vi "Civ idle2-2.vi"() -> ()   [LabVIEW 2013]
uses:
  <vilib>/Analysis/Matrix/Numeric/Conversions/Matrix To Array - RM.vi
  <vilib>/Analysis/Matrix/NI_Matrix.lvlib
panel:
  out "SP income":dbl
  out "EP income":dbl
  out "Land conversion rate":dbl
  out "BP income":dbl
  in  "Ticks/s":i32
  out "Gold upkeep":dbl
  out "Gold income/s":dbl format="%#_13g"
  out "BP upkeep":dbl
  out "Trading level":i32
  out "Build points":dbl
  out "Gold":dbl format="%#_13g"
  in  "?":T1(tab)
  in  "%Crafters":dbl
  in  "%Engineers":dbl
  in  "%Scientists":dbl
  in  "%Builders":dbl
  in  "%Warriors":dbl
  in  "%Hunters":dbl
  in  "Taxes level 0":bool
  in  "Taxes level 1":bool
  in  "Taxes level 2":bool
  in  "Taxes level 3":bool
  out "Taxation\nlevel":dbl format="%#_13g"
  in  "Taxes level 4":bool
  out "Food consumption\nmultiplier":dbl
  out "Food dissent mod":dbl
  in  "Normal food\nconsumption":bool
  in  "Highest food\nconsumption":bool
  in  "Higher food\nconsumption":bool
  out "Military\nScience level":i32
  out "Governance\nlevel":i32
  in  "Military science":bool
  in  "Governance":bool
  in  "Physics":bool
  in  "Construction":bool
  out "Physics level":i32
  out "Construction\nlevel":i32
  out "Economics\nlevel":i32
  in  "Economics":bool
  in  "Biology":bool
  out "Biology\nlevel":i32
  out "# of level 1 sciences":i32
  out "# of level 2 sciences":i32
  out "# of level 3 sciences":i32
  out "# of level 4 sciences":i32
  out "# of level 5 sciences":i32
  out "# of level 6 sciences":i32
  out "# of level 7 sciences":i32
  out "# of level 8 sciences":i32
  out "# of level 9 sciences":i32
  out "# of level 10 sciences":i32
  out "Production\nlevel":i32
  in  "Production":bool
  out "Spear level":i32
  out "Net level":i32
  in  "Sharpened stick":bool
  in  "Net 1":bool
  in  "Net 2":bool
  in  "Stone\nspear":bool
  in  "Bronze\nSpear":bool
  in  "Iron\nSpear":bool
  out "Bow level":i32
  in  "Bow 1":bool
  in  "Bow 2":bool
  out "Boat level":i32
  in  "Raft":bool
  in  "Trireme":bool
  out "Construction\ntools level":i32
  in  "Stone tools":bool
  in  "Basic\nmetal\ntools":bool
  out "Medicine level":i32
  in  "Medicine 1":bool
  in  "Medicine 2":bool
  in  "Medicine 3":bool
  in  "Advanced\nmetal\ntools":bool
  in  "Longbow":bool
  in  "Farming 1":bool
  out "Farming level":i32
  in  "Farming 2":bool
  out "Writing level":i32
  in  "Writing level 3":bool
  in  "Writing level 2":bool
  in  "Writing level 1":bool
  out "Animal\ndomestication\nlevel":i32
  in  "Livestock":bool
  in  "Selective\nbreeding":bool
  in  "Horses":bool
  out "Sword level":i32
  in  "Steel sword":bool
  in  "Iron sword":bool
  in  "Bronze sword":bool
  out "Tax method\nlevel":i32
  in  "Income tax":bool
  in  "Sales tax":bool
  in  "Tariffs":bool
  out "Siege weapon\nlevel":i32
  out "Chariot level":i32
  in  "Reinforced\nchariot":bool
  in  "Simple\nchariot":bool
  in  "Caravan":bool
  in  "Trebuchet":bool
  in  "Catapult":bool
  in  "Ballista":bool
  in  "Cannon":bool
  in  "Howitzer":bool
  in  "Rocket artillery":bool
  in  "Democracy":bool
  in  "Theocracy":bool
  in  "Warrior\nSociety":bool
  in  "Democracy 2":bool
  in  "Theocracy 2":bool
  in  "Warrior\nSociety 2":bool
  in  "Kingdom":bool
  in  "Republic":bool
  in  "Confederacy":bool
  in  "Senate":bool
  in  "Caste system":bool
  in  "Feudalism":bool
  out "Brick house level":i32
  out "Road level":i32
  out "Hut level":i32
  in  "Hut level 0":bool
  in  "Hut level 1":bool
  in  "Hut level 2":bool
  in  "Hut level 3":bool
  out "Road invested points":dbl
  out "Hut invested points":dbl
  in  "Road level 0":bool
  in  "Road level 3":bool
  in  "Road level 2":bool
  in  "Road level 1":bool
  out "Aqueduct level":i32
  out "Circus\ninvested points":dbl
  out "Circus/arena level":i32
  out "Aqueduct\ninvested points":dbl
  out "Harbor\ninvested points":dbl
  out "Harbor level":i32
  out "School invested points":dbl
  in  "School\nlevel 1":bool
  in  "School\nlevel 2":bool
  in  "School\nlevel 3":bool
  in  "School\nlevel 0":bool
  out "School level":i32
  in  "Wall level 1":bool
  in  "Wall level 2":bool
  in  "Wall level 3":bool
  in  "Wall level 0":bool
  out "Barracks level":i32
  out "Walls level":i32
  out "Wall invested points":dbl
  out "Barracks\ninvested points":dbl
  in  "Barracks\nlevel 3":bool
  in  "Barracks\nlevel 1":bool
  in  "Barracks\nlevel 0":bool
  in  "Barracks\nlevel 2":bool
  out "University level":i32
  in  "University\nlevel 0":bool
  in  "University\nlevel 3":bool
  in  "University\nlevel 2":bool
  in  "University\nlevel 1":bool
  out "University\ninvested points":dbl
  out "Mansion level":i32
  out "Temple level":i32
  out "Mansion\ninvested points":dbl
  out "Temple\ninvested points":dbl
  in  "Make Tier 2\nproducts":bool
  out "Tier 2\nproducts\nupkeep":dbl format="%#_13g"
  out "Tier 3\nproducts\nupkeep":dbl format="%#_13g"
  out "Tier 4\nproducts\nupkeep":dbl format="%#_13g"
  out "Tier 1\nproducts":dbl format="%#_13g"
  out "Tier 2\nproducts":dbl format="%#_13g"
  out "Tier 3\nproducts":dbl format="%#_13g"
  out "Tier 4\nproducts":dbl format="%#_13g"
  out "Tier 1\nproducts\nupkeep":dbl format="%#_13g"
  in  "Make Tier3\nproducts":bool
  in  "Make Tier 4\nproducts":bool
  out "hunting b":dbl
  out "hunting a":dbl
  out "warrior a":dbl
  out "warrior b":dbl
  out "warrior c":dbl
  out "1-Dissent/100":dbl format="%#_13g"
  out "Dissent multiplier":dbl
  out "Land conv mult":dbl
  out "Warrior b Gov mult":dbl
  out "Gov Economy\nbuildings mod":dbl
  out "-dissent per\nmilitary building":dbl
  out "Temp land change/s":dbl
  out "Year":i32
  out "Day":i32
  out "Military Modifier":dbl format="%#_13g"
  out "Taxation\nModifier":dbl format="%#_13g"
  out "Non-land production multiplier":dbl
  out "Hut non-land prod mod":dbl
  out "Hut upkeep":dbl
  out "Hut dissent mod":dbl
  out "Dissent addition modifiers":dbl
  out "Road land prod mod":dbl
  out "Road upkeep":dbl
  out "Road expansion bonus":dbl
  out "Trading level no mod":i32
  out "Taxes dissent mod":dbl
  out "Barracks military bonus":dbl
  out "Barracks upkeep":dbl
  out "Wall upkeep":dbl
  out "Wall dissent mod":dbl
  out "Construction multiplier":dbl
  out "Wall warrior % equivalent":dbl
  out "Gov building\nupkeep mod":dbl
  out "School dissent mod":dbl
  out "School upkeep":dbl
  out "School engineer equivalent":dbl
  out "School SP/EP multiplier":dbl
  out "Medicine dissent mod":i32
  out "Gov populist\nbuildings mod":dbl
  out "Gov elitist\nbuildings mod":dbl
  out "University SP multiplier":dbl
  out "University dissent mod":dbl
  out "University upkeep":dbl
  out "University scientist equivalent":dbl
  out "food income":dbl
  out "Aqueduct dissent mod":dbl
  out "Aqueduct upkeep":dbl
  out "Mansion dissent mod":dbl
  out "Mansion upkeep":dbl
  out "Harbor dissent mod":dbl
  out "Harbor upkeep":dbl
  out "Circus dissent mod":dbl
  out "Circus upkeep":dbl
  out "Temple dissent mod":dbl
  out "Temple upkeep":dbl
  out "Harbor military mod":dbl
  out "SP/EP multiplier":dbl
  out "Government":string
  out "Dissent":dbl
  out "SP":dbl
  out "EP":dbl
  in  "Percentage or absolute":bool
  out "Engineers":i32
  out "Crafters":i32
  out "Scientists":i32
  in  "#Merchants":dbl
  in  "Assign Merchant":bool
  in  "#Engineers":dbl
  in  "Assign Engineer":bool
  in  "#Scientists":dbl
  in  "Assign Scientist":bool
  out "Warriors":i32
  in  "Assign Builder":bool
  in  "#Builders":dbl
  out "Builders":i32
  in  "Assign Warrior":bool
  in  "#Warriors":dbl
  out "Unassigned workers":i32
  in  "Assign Hunters":bool
  in  "#Hunters":dbl
  in  "# people":i32
  in  "Increase\nPopulation":bool
  out "Conquered\nland":dbl
  out "Max hunters":i32
  out "Hunters":i32
  out "Food/s":dbl
  out "Permanent\nland":dbl
  out "People":i64
  in  "Stop Loop":bool
  out "Food":dbl
  # "Produces food, but your permanent land cannot support too many hunters"
  # "Conquers land, starting at 1km^2 per warrior, but has diminishing returns"
  # "Produces 1 BP/s, needed for buildings\nand for building upkeep"
  # "Produces 0.1 SP/s, used for abstract research which unlock upgrades and provide bonuses"
  # "Produces 0.1 EP/s, used for designing useful tools and upgrades"
  # "Produces Products, used mostly for late game upgrades.  Production scales with permanent land"
  # "Medium income from population, 8% dissent modifier"
  # "High income from population, 15% dissent modifier"
  # "Highest  income from population, 25% dissent modifier"
  # "No income from population, no dissent modifier"
  # "Low income from population, 3% dissent modifier"
  # "2 food/s/person,\n-10% dissent"
  # "1 food/s/person, no dissent mod"
  # "1.5 food/s/person,\n-5% dissent"
  # "Requires Governance 2"
  # "Each level costs 1000 *10^current level SP"
  # "Reduces diminishing returns \nfrom military size, unlocks \nnew weapons/tactics"
  # "Slightly decreases dissent,\nunlocks new governments"
  # "Increases EP and SP generation, \nunlocks various upgrades"
  # "Decreases building upkeep costs,\nunlocks buildings"
  # "Increase gold generation,\nunlocks gold and taxation"
  # "Increase food production,\nunlocks farming and medicine"
  # "Increases production by 20%\nper tier per level"
  # "Costs 2,000EP\nHunters and warriors are more effective"
  # "Costs 10,000EP\nRequires military 1,\nHunters and warriors are more effective"
  # "Costs 50,000EP\nRequires military 2,\nWarriors are more effective"
  # "Costs 2,000,000EP\nRequires military 4,\nWarriors are more effective"
  # "Costs 10,000EP\nHunters can produce more food"
  # "Costs 100,000EP\nHunters can produce more food"
  # "Costs 100,000EP\nRequires military 3,\nWarriors are much more effective, hunters can produce more food"
  # "Costs 300,000EP\nRequires military 3, physics 3\nWarriors and Hunters are more effective"
  # "Costs 30M EP\nRequires military 5, physics 4\nWarriors are more effective"
  # "Costs 300,000EP\nRequires physics 3,\nImproves trade and hunting"
  # "Costs 3,000,000EP\nRequires physics 4, military 3\nImproves trade and warriors"
  # "Costs 30,000EP\nRequires physics 2, construction 2\nBuilders produce 0.5 more BP/s"
  # "Costs 500,000EP\nRequires physics 3,\nconstruction 3,Builders produce 0.5 more BP/s"
  # "Costs 200M EP\nRequires physics 5,\nconstruction 5,Builders produce 1 more BP/s"
  # "Costs 30,000EP\nRequires biology 2,\nreduces dissent by another 1% (2% total)"
  # "Costs 3M EP\nRequires biology 4,\nreduces dissent by another 2% (4% total)"
  # "Costs 3,000EP\nRequires biology 1,\nreduces dissent by 1%"
  # "Costs 10M EP\nRequires Biology 3\nRenames hunters to farmers, massive improvements to food production, increases food from tribute"
  # "Costs 100M EP\nRequires Biology 4\nLarge improvements to food production, increases food from tribute"
  # "Costs 10k EP\nImproves EP and SP production by 10%"
  # "Costs 1M EP\nImproves EP and SP production by 10%"
  # "Costs 100M EP\nImproves EP and SP production by 10%"
  # "Costs 30M EP\nRequires Biology 3\nImproves warrior effectiveness,  builder BP/s by 0.5"
  # "Costs 30k EP\nRequires Biology 1\nImproves hunter food production"
  # "Costs 1M EP\nRequires Biology 2\nImproves warrior effectiveness,  builder BP/s by 0.5"
  # "Costs 1M EP\nRequires Military 3\nImproves warrior effectiveness"
  # "Costs 30M EP\nRequires Military 4\nImproves warrior effectiveness"
  # "Costs 1B EP\nRequires Military 6\nImproves warrior effectiveness"
  # "Costs 1M EP\nRequires Economics 3\nImproves taxation effectiveness by 50%"
  # "Costs 30M EP\nRequires Economics 4\nImproves taxation effectiveness by 50%"
  # "Costs 1B EP\nRequires Economics 6\nImproves taxation effectiveness by 50%"
  # "Costs 500k EP\nRequires Military 3, Physics 3, Improves warrior effectiveness"
  # "Costs 5M EP\nRequires Military 3, Physics 4, Improves warrior effectiveness"
  # "Costs 10M EP\nRequires Economics 4, Physics 4, Increases trade level"
  # "Costs 5M EP\nRequires Military 3, Physics 4, Improves\nwarrior effectiveness"
  # "Costs 30M EP\nRequires Military 3, Physics 5, Improves\nwarrior effectiveness"
  # "Costs 300M EP\nRequires Military 4, Physics 6, Improves\nwarrior effectiveness"
  # "Costs 3B EP\nRequires Military 6, Physics 7, Improves\nwarrior effectiveness"
  # "Costs 30B EP\nRequires Military 7, Physics 8, Improves\nwarrior effectiveness"
  # "Costs 300B EP\nRequires Military 8, Physics 9, Improves\nwarrior effectiveness"
  # "Costs 1000SP\nRequires Governance 1"
  # "Costs 25000SP\nRequires Governance 2"
  # "Costs 5M SP\nRequires Governance 4"
  # "Reduces dissent by 2,4,6%\nImproves non-land production by 10,20,30%\nRequires Construction 1"
  # "Upkeep:        0                          0.01BP                0.03BP              0.15BP"
  # "Cost:             0                          10k   BP              30k BP            150k BP"
  # "Increases trade level by 1,2,3\nImproves land production\n by 10,20,30%\nImproves land conversion\nrate by 20,50,100%\nRequires Construction 1"
  # "Upkeep:        0                          0.02BP                0.06BP              0.2BP"
  # "Cost:             0                          50k BP              150k BP             500k BP"
  # "Increases military effectiveness (b) by 10,20,30%\nRequires Construction 2, Military 2"
  # "Upkeep:        0                          0.001GP             0.003GP             0.01GP"
  # "Cost:             0                          100k BP             300k BP              1M BP"
  # "Adds to the base strength of your military, giving the equivalent of 2,4,6% of your population as warriors\nReduces dissent by 2,4,6%\nRequires Construction 3, Military 2"
  # "Upkeep:        0                          0.002GP            0.006GP            0.02GP"
  # "Cost:             0                          1M BP              3M BP               10M BP"
  # "Provides a 5,10,15% bonus to SP/EP production, reduces dissent by 1,2,3%, adds 1,2,3% of population to base  engineer\nRequires Construction 2, Governance 2"
  # "Upkeep:        0                          0.001GP             0.003GP           0.01GP"
  # "Cost:              0                          200k BP             600k BP            2M BP"
  # "Provides a 5,10,15% bonus to SP/EP production, reduces dissent by 1,2,3%, adds 1,2,3% of population to base  engineer\nRequires Construction 2, Governance 2"
  # "Upkeep:        0                          0.005GP             0.015GP          0.05GP"
  # "Cost:              0                          600k BP             2M BP             5M BP"
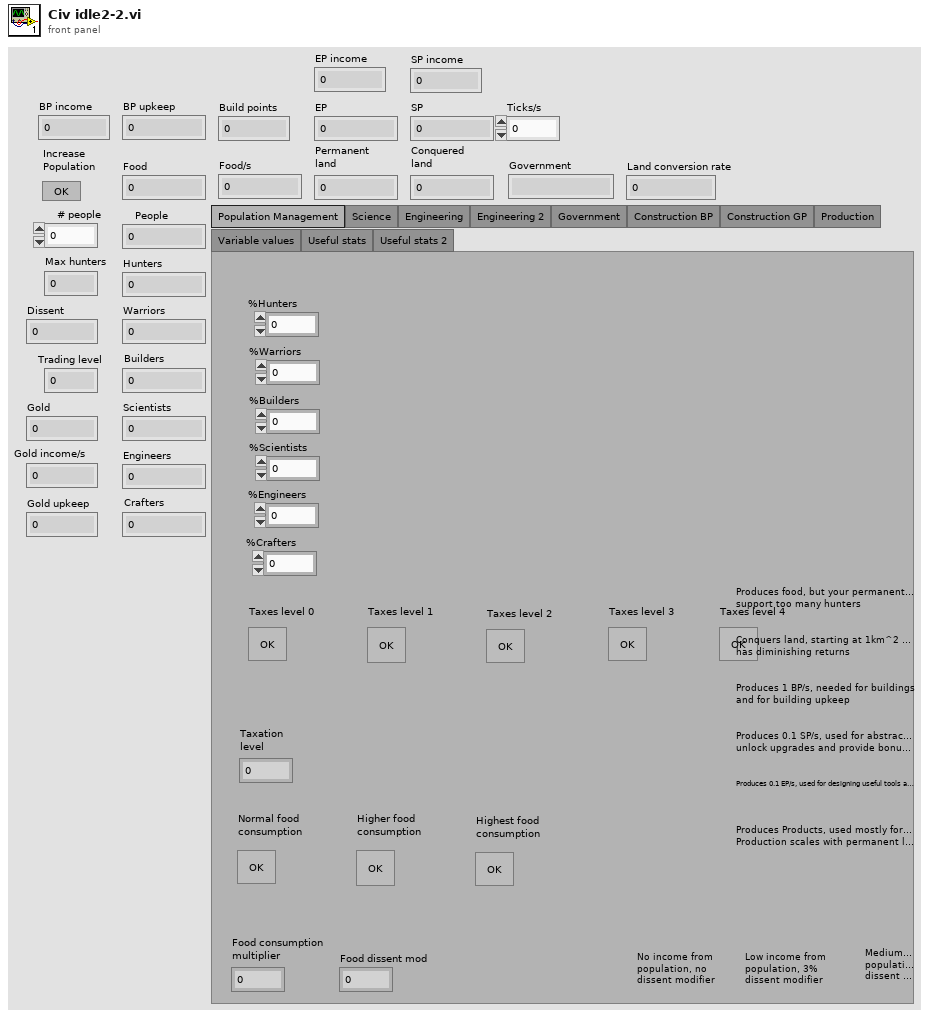
[diagram p1: front panel]
types:
  T1 = enum32{"Population Management", "Science", "Engineering", "Engineering 2", "Government", "Construction BP", "Construction GP", "Production", "Variable values", "Useful stats", "Useful stats 2"}
  T2 = typedef "NI_Matrix.lvlib/RealMatrix.ctl" = dbl[][]
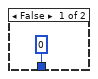
[diagram p2: hidden frame]
diagram:
  n1 = while {
    i -> [w1520]
    stop <- "Stop Loop" stop-if-true
    w168 = 10000000 ("y")
    w179 = 10000000 ("y")
    w200 = 10000000 ("y")
    w237 = 10000000 ("y")
    w226 = 5000000 ("y")
    w217 = 500000 ("y")
    w270 = 10000000 ("y")
    w281 = 5000000 ("y")
    w290 = 500000 ("y")
    w306 = 1000000000 ("y")
    w317 = 30000000 ("y")
    w326 = 1000000 ("y")
    w384 = 1000000000 ("y")
    w373 = 30000000 ("y")
    w364 = 1000000 ("y")
    w393 = 30000000 ("y")
    w404 = 1000000 ("y")
    w413 = 30000 ("y")
    w444 = 100000000 ("y")
    w433 = 1000000 ("y")
    w424 = 10000 ("y")
    w473 = 1 ("y")
    w465 = 2 ("y")
    w464 = 1.5 ("y")
    w508 = 0 ("y")
    w509 = 3 ("y")
    w528 = 2 ("y")
    w529 = 1 ("y")
    w568 = 30000000 ("y")
    w584 = 500000 ("y")
    w602 = 3000000 ("y")
    w613 = 30000 ("y")
    w628 = 3000 ("y")
    w685 = 0 ("y")
    w684 = 3 ("y")
    w665 = 2 ("y")
    w664 = 1 ("y")
    w711 = "Senate" ("y")
    w735 = "Caste system" ("y")
    w748 = "Feudalism" ("y")
    w786 = "Kingdom" ("y")
    w762 = "Republic" ("y")
    w749 = "Confederacy" ("y")
    w801 = 3 ("y")
    w818 = 500000 ("y")
    w829 = 30000 ("y")
    w877 = 0 ("y")
    w878 = 3 ("y")
    w897 = 2 ("y")
    w898 = 1 ("y")
    w941 = 0 ("y")
    w942 = 3 ("y")
    w961 = 2 ("y")
    w962 = 1 ("y")
    w1004 = 0 ("y")
    w1005 = 3 ("y")
    w1020 = 2 ("y")
    w1021 = 1 ("y")
    w1126 = 3 ("y")
    w1137 = 2 ("y")
    w1175 = 0 ("y")
    w1174 = 3 ("y")
    w1155 = 2 ("y")
    w1154 = 1 ("y")
    w1195 = 0 ("y")
    w1196 = 1 ("y")
    w1208 = 100000000 ("y")
    w1235 = 10000000 ("y")
    w1258 = 3000000 ("y")
    w1269 = 300000 ("y")
    w1301 = 300000 ("y")
    w1327 = 100000 ("y")
    w1330 = 2000000 ("y")
    w1329 = 50000 ("y")
    w1393 = "Warrior Society 2" ("y")
    w1417 = "Theocracy 2" ("y")
    w1430 = "Democracy 2" ("y")
    w1437 = "Warrior Society" ("y")
    w1450 = "Theocracy" ("y")
    w1466 = "Democracy" ("y")
    w1490 = 2000 ("y")
    # "Constructions initial build"
    # "SCIENCES"
    # "GOVERNMENTS"
    # "ENGINEERING"
    n2 = local read "Food consumption\nmultiplier"() -> (w474:dbl)
    n3 = local read "Barracks\ninvested points"() -> (w1036:dbl)
    n4 = local read "Wall invested points"() -> (w921:dbl)
    n5 = local read "Food consumption\nmultiplier"() -> (w466:dbl)
    n6 = local read "Governance\nlevel"() -> (w471:i32)
    n7 = local read "Military\nScience level"() -> (w863:i32)
    n8 = local read "Governance\nlevel"() -> (w479:i32)
    n9 = local read "Construction\nlevel"() -> (w1186:i32)
    n10 = local read "Construction\nlevel"() -> (w889:i32)
    n11 = local read "Construction\nlevel"() -> (w1163:i32)
    n12 = local read "Military\nScience level"() -> (w850:i32)
    n13 = local read "Construction\nlevel"() -> (w866:i32)
    n14 = local read "Build points"() -> (w917:dbl)
    n15 = local read "Barracks level"() -> (w1181:i32)
    n16 = local read "Build points"() -> (w1040:dbl)
    n17 = local read "Military\nScience level"() -> (w844:i32)
    n18 = local read "Walls level"() -> (w871:i32)
    n19 = local read "Build points"() -> (w1180:dbl)
    n20 = local read "Build points"() -> (w872:dbl)
    n21 = local read "Walls level"() -> (w894:i32)
    n22 = local read "Barracks level"() -> (w1158:i32)
    n23 = Subtract(x=3000000 ("y"), y=w921) -> (x-y=w914:dbl)
    n24 = Subtract(x=300000 ("y"), y=w1036) -> (x-y=w1043:dbl)
    n25 = Greater Or Equal?(x=w479, y=2) -> (x >= y?=w481:bool)
    n26 = And(x="Normal food\nconsumption", y=w481) -> (x .and. y?=w477:bool)
    n27 = Greater Or Equal?(x=w471, y=2) -> (x >= y?=w483:bool)
    n28 = And(x="Highest food\nconsumption", y=w483) -> (x .and. y?=w469:bool)
    n29 = local read "Food consumption\nmultiplier"() -> (w455:dbl)
    n30 = local read "Ticks/s"() -> (w792:i32)
    n31 = Not Equal?(x=w474, y=w473) -> (x != y?=w476:bool)
    n32 = And(x=w476, y=w477) -> (x .and. y?=w475:bool)
    n33 = Max & Min(x=w914, y=0.0) -> (max(x,y)=w919:dbl)  [unwired: 1 out]
    n34 = Greater Or Equal?(x=w863, y=2) -> (x >= y?=w861:bool)
    n35 = Not Equal?(x=w466, y=w465) -> (x != y?=w468:bool)
    n36 = And(x=w468, y=w469) -> (x .and. y?=w467:bool)
    n37 = Max & Min(x=w1043, y=0.0) -> (max(x,y)=w1038:dbl)  [unwired: 1 out]
    n38 = Greater Or Equal?(x=w917, y=w919) -> (x >= y?=w918:bool)
    n39 = local read "Military\nScience level"() -> (w857:i32)
    n40 = Greater Or Equal?(x=w1040, y=w1038) -> (x >= y?=w1039:bool)
    n41 = for {
      N: 1 -> [_]
      tunnel: [w2227] -> w1144 mode=indexing
      n42 = local read "Production\nlevel"() -> (w2223:i32)
      n43 = local read "Permanent\nland"() -> (w2224:dbl)
      n44 = local read "Construction multiplier"() -> (w2253:dbl)
      n45 = local read "University scientist equivalent"() -> (w2240:dbl)
      n46 = local read "Taxation\nlevel"() -> (w2290:dbl)
      n47 = local read "1-Dissent/100"() -> (w2222:dbl)
      n48 = local read "Conquered\nland"() -> (w2305:dbl)
      n49 = local read "Non-land production multiplier"() -> (w2198:dbl)
      n50 = local read "Tier 2\nproducts"() -> (w2213:dbl)
      n51 = local read "Government"() -> (w2308:string)
      n52 = local read "University SP multiplier"() -> (w2237:dbl)
      n53 = local read "Economics\nlevel"() -> (w2291:i32)
      n54 = local read "SP/EP multiplier"() -> (w2246:dbl)
      n55 = local read "People"() -> (w2227:i64)
      n56 = local read "Conquered\nland"() -> (w2294:dbl)
      n57 = local read "Crafters"() -> (w2228:i32)
      n58 = local read "Economics\nlevel"() -> (w2296:i32)
      n59 = local read "Trading level"() -> (w2295:i32)
      n60 = local read "Non-land production multiplier"() -> (w2279:dbl)
      n61 = local read "School engineer equivalent"() -> (w2249:dbl)
      n62 = local read "Taxation\nModifier"() -> (w2288:dbl)
      n63 = local read "Tax method\nlevel"() -> (w2231:i32)
      n64 = local read "1-Dissent/100"() -> (w2281:dbl)
      n65 = local read "Physics level"() -> (w2282:i32)
      n66 = local read "Tier 2\nproducts\nupkeep"() -> (w2204:dbl)
      n67 = Power Of X(1:w2227, 2:-0.5 ("y")) -> (0:w2225:dbl)
      n68 = Power Of X(1:1.2 ("x"), 2:w2223) -> (0:w2212:dbl)
      n69 = case shown="\"Tribe\", Default" w2308 {
        tunnel: w2227 -> [w2356 w2368 w2377 w2393 w2398 w2417 w2427 w2449 w2463 w2485 w2498 w2516 w2536 _ _ _ _ _ _ _ _ _ _ _ _ _ _ _]
        tunnel: w2224 -> [_ w2370 w2378 _ _ _ _ w2454 w2462 _ w2503 _ w2533 _ _ _ _ _ _ _ _ _ _ _ _ _ _ _]
        tunnel: [w2359 w2366 w2376 w2389 w2401 w2410 w2429 w2446 w2461 w2481 w2491 w2509 w2525 _ _ _ _ _ _ _ _ _ _ _ _ _ _ _] -> w2306
        tunnel: w2305 -> [_ _ _ _ _ w2421 w2428 w2453 _ _ w2502 w2519 _ _ _ _ _ _ _ _ _ _ _ _ _ _ _ _]
        tunnel: [1 0.85 0.7 1 1 2 3 1.5 ("y") 1.0 ("y") 2.0 ("y") 3.0 ("y") 6.0 ("y") 0.7 ("y") _ _ _ _ _ _ _ _ _ _ _ _ _ _ _] -> w2304
        tunnel: [1.0 2.0 4.0 1.0 1.0 0.2 0.05 1.5 ("y") 3.0 ("y") 1.0 ("y") 0.1 ("y") 0.025 ("y") 8.0 ("y") _ _ _ _ _ _ _ _ _ _ _ _ _ _ _] -> w2303
        tunnel: [1 1 1 0.5 0.333 1 1 1.0 ("y") 0.5 ("y") 0.5 ("y") 1.0 ("y") 1.0 ("y") 1.0 ("y") _ _ _ _ _ _ _ _ _ _ _ _ _ _ _] -> w2261
        tunnel: [1.0 ("y") 1.5 ("y") 2.0 ("y") 0.5 ("y") 0.33 ("y") 0.5 ("y") 0.5 ("y") 1.25 ("y") 2.0 ("y") 1.0 ("y") 0.5 ("y") 0.5 ("y") 2.5 ("y") _ _ _ _ _ _ _ _ _ _ _ _ _ _ _] -> w2252
        tunnel: [1.0 ("y") 0.75 ("y") 0.5 ("y") 1.5 ("y") 2.0 ("y") 1.5 ("y") 1.5 ("y") 1.25 ("y") 0.5 ("y") 1.0 ("y") 1.5 ("y") 2.0 ("y") 0.5 ("y") _ _ _ _ _ _ _ _ _ _ _ _ _ _ _] -> w2245
        tunnel: [0.0 ("y") _ _ 0.5 ("y") 0.5 ("y") 1.0 ("y") 1.0 ("y") 1.0 ("y") _ 0.5 ("y") 1.0 ("y") 0.0 ("y") 0.0 ("y") _ _ _ _ _ _ _ _ _ _ _ _ _ _ _] -> w2244
        tunnel: [1.0 ("y") _ _ _ _ _ _ 1.25 ("y") 1.5 ("y") 0.7 ("y") 0.5 ("y") 0.5 ("y") 1.0 ("y") _ _ _ _ _ _ _ _ _ _ _ _ _ _ _] -> w2243
        frame "Tribe", Default {
          n70 = Divide(x=w2356, y=i64 2) -> (x/y=w2354:dbl)
          n71 = Subtract(x=w2354, y=i64 50) -> (x-y=w2359:dbl)
        }
        frame "Democracy" {
          n72 = Square Root(x=w2370) -> (sqrt(x)=w2369:dbl)
          n73 = Divide(x=w2368, y=w2369) -> (x/y=w2367:dbl)
          n74 = Square Root(x=w2367) -> (sqrt(x)=w2372:dbl)
          n75 = Multiply(x=2, y=w2372) -> (x*y=w2366:dbl)
        }
        frame "Democracy 2" {
          n76 = Square Root(x=w2378) -> (sqrt(x)=w2382:dbl)
          n77 = Divide(x=w2377, y=w2382) -> (x/y=w2381:dbl)
          n78 = Square Root(x=w2381) -> (sqrt(x)=w2376:dbl)
        }
        frame "Theocracy" {
          n79 = Y-th Root of X(1:w2393, 2:i64 3 ("y")) -> (0:w2390:dbl)
          n80 = Add(x=w2390, y=15.0) -> (x+y=w2389:dbl)
        }
        frame "Theocracy 2" {
          n81 = Y-th Root of X(1:w2398, 2:3.5 ("y")) -> (0:w2404:dbl)
          n82 = Add(x=w2404, y=15.0) -> (x+y=w2401:dbl)
        }
        frame "Warrior Society" {
          n83 = Square Root(x=w2417) -> (sqrt(x)=w2414:dbl)
          n84 = Y-th Root of X(1:w2421, 2:3.0 ("y")) -> (0:w2420:dbl)
          n85 = Multiply(x=0.5, y=w2414) -> (x*y=w2413:dbl)
          n86 = Add(x=w2413, y=10.0) -> (x+y=w2412:dbl)
          n87 = Multiply(x=w2420, y=2.0) -> (x*y=w2411:dbl)
          n88 = Subtract(x=w2412, y=w2411) -> (x-y=w2410:dbl)
        }
        frame "Warrior Society 2" {
          n89 = Square Root(x=w2427) -> (sqrt(x)=w2437:dbl)
          n90 = Y-th Root of X(1:w2428, 2:2.5 ("y")) -> (0:w2433:dbl)
          n91 = Multiply(x=0.4, y=w2437) -> (x*y=w2438:dbl)
          n92 = Add(x=w2438, y=10.0) -> (x+y=w2439:dbl)
          n93 = Multiply(x=w2433, y=1.0) -> (x*y=w2440:dbl)
          n94 = Subtract(x=w2439, y=w2440) -> (x-y=w2429:dbl)
        }
        frame "Senate" {
          n95 = Multiply(x=w2454, y=w2453) -> (x*y=w2452:dbl)
          n96 = Power Of X(1:w2452, 2:0.3 ("y")) -> (0:w2450:dbl)
          n97 = Divide(x=w2449, y=w2450) -> (x/y=w2448:dbl)
          n98 = Y-th Root of X(1:w2448, 2:2.0 ("y")) -> (0:w2444:dbl)
          n99 = Multiply(x=1.5, y=w2444) -> (x*y=w2446:dbl)
        }
        frame "Republic" {
          n100 = Power Of X(1:w2462, 2:0.6 ("y")) -> (0:w2468:dbl)
          n101 = Divide(x=w2463, y=w2468) -> (x/y=w2467:dbl)
          n102 = Y-th Root of X(1:w2467, 2:2.0 ("y")) -> (0:w2464:dbl)
          n103 = Multiply(x=1.5, y=w2464) -> (x*y=w2461:dbl)
        }
        frame "Kingdom" {
          n104 = Power Of X(1:w2485, 2:0.2564 ("y")) -> (0:w2482:dbl)
          n105 = Add(x=w2482, y=5.0) -> (x+y=w2481:dbl)
        }
        frame "Feudalism" {
          n106 = Multiply(x=w2503, y=w2502) -> (x*y=w2501:dbl)
          n107 = Y-th Root of X(1:w2498, 2:3.0 ("y")) -> (0:w2497:dbl)
          n108 = Y-th Root of X(1:w2501, 2:7.0 ("y")) -> (0:w2492:dbl)
          n109 = Divide(x=w2497, y=2.0) -> (x/y=w2495:dbl)
          n110 = Add(x=w2495, y=5.0) -> (x+y=w2493:dbl)
          n111 = Subtract(x=w2493, y=w2492) -> (x-y=w2491:dbl)
        }
        frame "Caste system" {
          n112 = Y-th Root of X(1:w2516, 2:3.5 ("y")) -> (0:w2515:dbl)
          n113 = Y-th Root of X(1:w2519, 2:4.5 ("y")) -> (0:w2510:dbl)
          n114 = Multiply(x=w2515, y=0.7) -> (x*y=w2513:dbl)
          n115 = Add(x=w2513, y=10.0) -> (x+y=w2511:dbl)
          n116 = Subtract(x=w2511, y=w2510) -> (x-y=w2509:dbl)
        }
        frame "Confederacy" {
          n117 = Power Of X(1:w2536, 2:0.9 ("y")) -> (0:w2534:dbl)
          n118 = Square Root(x=w2533) -> (sqrt(x)=w2537:dbl)
          n119 = Divide(x=w2534, y=w2537) -> (x/y=w2526:dbl)
          n120 = Power Of X(1:w2526, 2:0.55 ("y")) -> (0:w2525:dbl)
        }
        frame "Imperialism" {
        }
        frame "Empire" {
        }
        frame "Free market capitalism" {
        }
        frame "Corporatism" {
        }
        frame "Fascism" {
        }
        frame "Communist dictatorship" {
        }
        frame "Socialism" {
        }
        frame "Advanced democracy?" {
        }
        frame "Advanced imperialism?" {
        }
        frame "Meritocracy" {
        }
        frame "Genetically optimized workforce" {
        }
        frame "Future democracy?" {
        }
        frame "Hivemind" {
        }
        frame "AI overlord" {
        }
        frame "Robots do all work" {
        }
      }
      n121 = local read "Build points"() -> (w2255:dbl)
      n122 = local read "Build points"() -> (w2262:dbl)
      n123 = Compound Arithmetic op=MULTIPLY(w2228, w2198, w2225, w2224, w2212, w2222, 0.001 ("x")) -> (w2220:dbl)
      n124 = local read "Builders"() -> (w2264:i32)
      n125 = local read "Tier 3\nproducts"() -> (w2210:dbl)
      n126 = local read "Tier 1\nproducts"() -> (w2219:dbl)
      n127 = local read "Tier 1\nproducts\nupkeep"() -> (w2216:dbl)
      n128 = Add(x=w2220, y=w2219) -> (x+y=w2217:dbl)
      n129 = local read "Dissent"() -> (w2300:dbl)
      n130 = local read "Tier 3\nproducts\nupkeep"() -> (w2202:dbl)
      n131 = local read "Tier 4\nproducts\nupkeep"() -> (w2201:dbl)
      n132 = Power Of X(1:2 ("x"), 2:w2231) -> (0:w2229:dbl)
      n133 = Compound Arithmetic op=MULTIPLY(w2296, w2295, w2294, 0.001 ("value")) -> (w2260:dbl)
      n134 = local write "Gov populist\nbuildings mod"(w2252) -> ()
      n135 = local write "-dissent per\nmilitary building"(w2244) -> ()
      n136 = Compound Arithmetic op=MULTIPLY(w2227, w2291, w2290, w2288, 0.0005 ("value"), w2229) -> (w2259:dbl)
      n137 = local write "Gov elitist\nbuildings mod"(w2245) -> ()
      n138 = local read "Gold"() -> (w2292:dbl)
      n139 = Power Of X(1:1.1 ("x"), 2:w2282) -> (0:w2266:dbl)
      n140 = Subtract(x=w2217, y=w2216) -> (x-y=w2197:dbl)
      n141 = Divide(x=w2255, y=10.0) -> (x/y=w2254:dbl)
      n142 = Compound Arithmetic op=ADD(w2292, w2260, w2259) -> (w2283:dbl)
      n143 = Divide(x=w2300, y=100.0) -> (x/y=w2302:dbl)
      n144 = Compound Arithmetic op=MULTIPLY(w2266, w2281, 0.1, w2279, w2246) -> (w2267:dbl)
      n145 = Divide(x=w2267, y=w2266) -> (x/y=w2265:dbl)
      n146 = Compound Arithmetic op=MULTIPLY(w2265, 10.0 ("value"), w2264, w2253, w2246) -> (w2251:dbl)
      n147 = Add(x=w2251, y=w2262) -> (x+y=w2263:dbl)
      n148 = Less?(x=w2283, y=-50.0) -> (x < y?=w2286:bool)
      n149 = local read "Tier 4\nproducts"() -> (w2207:dbl)
      n150 = Greater?(x=w2197, y=0.0) -> (0:w2195:bool)
      n151 = Subtract(x=1.0, y=w2302) -> (x-y=w2298:dbl)
      n152 = Add(x=w2260, y=w2259) -> (x+y=w2258:dbl)
      n153 = local read "Dissent addition modifiers"() -> (w2275:dbl)
      n154 = local read "Engineers"() -> (w2248:i32)
      n155 = And(x="Make Tier 2\nproducts", y=w2195) -> (x .and. y?=w2193:bool)
      n156 = local write "Build points"(w2263) -> ()
      n157 = local write "Gold income/s"(w2258) -> ()
      n158 = case shown="True" w2286 {
        tunnel: w2283 -> [_ w2344]
        tunnel: w2227 -> [_ w2348]
        tunnel: [0 w2345] -> w2272
        frame False {
        }
        frame True {
          n159 = Negate(x=w2344) -> (-x=w2343:dbl)
          n160 = Divide(x=w2343, y=w2348) -> (x/y=w2347:dbl)
          n161 = Max & Min(x=w2347, y=20.0) -> (min(x,y)=w2345:dbl)  [unwired: 1 out]
        }
      }
      n162 = local read "Scientists"() -> (w2241:i32)
      n163 = local write "Gold"(w2283) -> ()
      n164 = Less?(x=w2254, y=-50.0) -> (x < y?=w2274:bool)
      n165 = local write "1-Dissent/100"(w2298) -> ()
      n166 = local read "Dissent multiplier"() -> (w2307:dbl)
      n167 = local write "Warrior b Gov mult"(w2304) -> ()
      n168 = Multiply(x=w2306, y=w2307) -> (x*y=w2277:dbl)
      n169 = case shown="True" w2193 {
        tunnel: w2197 -> [w2328 w2334]
        tunnel: w2212 -> [_ w2331]
        tunnel: [w2328 w2330] -> w2218
        tunnel: [0.0 w2329] -> w2214
        frame False {
        }
        frame True {
          n170 = Divide(x=100.0 ("y"), y=w2331) -> (x/y=w2333:dbl)
          n171 = Quotient & Remainder(x=w2334, y=w2333) -> (x-y*floor(x/y)=w2330:dbl, floor(x/y)=w2329:dbl)
        }
      }
      n172 = Add(x=w2214, y=w2213) -> (x+y=w2205:dbl)
      n173 = Subtract(x=w2205, y=w2204) -> (x-y=w2191:dbl)
      n174 = Greater?(x=w2191, y=0.0) -> (0:w2190:bool)
      n175 = And(x="Make Tier3\nproducts", y=w2190) -> (x .and. y?=w2188:bool)
      n176 = case shown="True" w2188 {
        tunnel: w2191 -> [w2320 w2326]
        tunnel: w2212 -> [_ w2323]
        tunnel: [w2320 w2322] -> w2211
        tunnel: [0.0 w2321] -> w2209
        frame False {
        }
        frame True {
          n177 = Divide(x=100.0 ("y"), y=w2323) -> (x/y=w2325:dbl)
          n178 = Quotient & Remainder(x=w2326, y=w2325) -> (x-y*floor(x/y)=w2322:dbl, floor(x/y)=w2321:dbl)
        }
      }
      n179 = local write "Tier 2\nproducts"(w2211) -> ()
      n180 = Add(x=w2209, y=w2210) -> (x+y=w2203:dbl)
      n181 = Subtract(x=w2203, y=w2202) -> (x-y=w2183:dbl)
      n182 = Greater?(x=w2183, y=0.0) -> (0:w2187:bool)
      n183 = And(x="Make Tier 4\nproducts", y=w2187) -> (x .and. y?=w2184:bool)
      n184 = case shown="True" w2184 {
        tunnel: w2183 -> [w2312 w2318]
        tunnel: w2212 -> [_ w2316]
        tunnel: [w2312 w2315] -> w2208
        tunnel: [0.0 w2314] -> w2200
        frame False {
        }
        frame True {
          n185 = Divide(x=100.0 ("y"), y=w2316) -> (x/y=w2313:dbl)
          n186 = Quotient & Remainder(x=w2318, y=w2313) -> (x-y*floor(x/y)=w2315:dbl, floor(x/y)=w2314:dbl)
        }
      }
      n187 = local write "Land conv mult"(w2303) -> ()
      n188 = Multiply(x=w2227, y=w2240) -> (x*y=w2239:dbl)
      n189 = case shown="True" w2274 {
        tunnel: w2227 -> [_ w2341]
        tunnel: [0 w2338] -> w2268
        tunnel: w2254 -> [_ w2336]
        frame False {
        }
        frame True {
          n190 = Negate(x=w2336) -> (-x=w2337:dbl)
          n191 = Divide(x=w2337, y=w2341) -> (x/y=w2340:dbl)
          n192 = Max & Min(x=w2340, y=20.0) -> (min(x,y)=w2338:dbl)  [unwired: 1 out]
        }
      }
      n193 = Add(x=w2272, y=w2268) -> (x+y=w2271:dbl)
      n194 = Add(x=w2277, y=w2275) -> (x+y=w2276:dbl)
      n195 = local read "EP"() -> (w2310:dbl)
      n196 = Multiply(x=w2249, y=w2227) -> (x*y=w2250:dbl)
      n197 = Subtract(x=w2200, y=w2201) -> (x-y=w2199:dbl)
      n198 = Add(x=w2199, y=w2207) -> (x+y=w2206:dbl)
      n199 = local read "SP"() -> (w2242:dbl)
      n200 = local write "Gov Economy\nbuildings mod"(w2243) -> ()
      n201 = Add(x=w2248, y=w2250) -> (x+y=w2247:dbl)
      n202 = Multiply(x=w2267, y=w2247) -> (x*y=w2236:dbl)
      n203 = local write "Gov building\nupkeep mod"(w2261) -> ()
      n204 = Max & Min(x=0.0, y=w2276) -> (max(x,y)=w2284:dbl)  [unwired: 1 out]
      n205 = Add(x=w2239, y=w2241) -> (x+y=w2238:dbl)
      n206 = Compound Arithmetic op=MULTIPLY(w2267, w2237, w2238) -> (w2235:dbl)
      n207 = Max & Min(x=w2271, y=20.0) -> (min(x,y)=w2269:dbl)  [unwired: 1 out]
      n208 = Add(x=w2269, y=w2284) -> (x+y=w2234:dbl)
      n209 = Add(x=w2310, y=w2236) -> (x+y=w2309:dbl)
      n210 = Add(x=w2242, y=w2235) -> (x+y=w2278:dbl)
      n211 = local write "Tier 3\nproducts"(w2208) -> ()
      n212 = Max & Min(x=90.0, y=w2234) -> (min(x,y)=w2232:dbl)  [unwired: 1 out]
      n213 = local write "Tier 4\nproducts"(w2206) -> ()
      n214 = local write "Tier 1\nproducts"(w2218) -> ()
      n215 = local write "BP income"(w2251) -> ()
      n216 = local write "EP"(w2309) -> ()
      n217 = local write "SP"(w2278) -> ()
      n218 = local write "SP income"(w2235) -> ()
      n219 = local write "EP income"(w2236) -> ()
      n220 = local write "Dissent"(w2232) -> ()
    }
    n221 = Greater Or Equal?(x=w1186, y=2) -> (x >= y?=w1177:bool)
    n222 = Greater Or Equal?(x=w866, y=3) -> (x >= y?=w875:bool)
    n223 = Greater Or Equal?(x=w1180, y=0) -> (x >= y?=w1178:bool)
    n224 = Greater Or Equal?(x=w872, y=0) -> (x >= y?=w874:bool)
    n225 = case shown="True" w475 {
      tunnel: w473 -> [_ w1665]
      frame False {
      }
      frame True {
        n226 = local write "Food consumption\nmultiplier"(w1665) -> ()
        n227 = local write "Food dissent mod"(0.0 ("Taxes dissent add mod")) -> ()
      }
    }
    n228 = Greater Or Equal?(x=w889, y=3) -> (x >= y?=w895:bool)
    n229 = Greater Or Equal?(x=w850, y=2) -> (x >= y?=w849:bool)
    n230 = Greater Or Equal?(x=w1163, y=2) -> (x >= y?=w1157:bool)
    n231 = case shown="True" w467 {
      tunnel: w465 -> [_ w1667]
      frame False {
      }
      frame True {
        n232 = local write "Food consumption\nmultiplier"(w1667) -> ()
        n233 = local write "Food dissent mod"(-10.0 ("Taxes dissent add mod")) -> ()
      }
    }
    n234 = Not Equal?(x=w1181, y=w1175) -> (x != y?=w1183:bool)
    n235 = Not Equal?(x=w871, y=w877) -> (x != y?=w869:bool)
    n236 = Greater Or Equal?(x=w844, y=2) -> (x >= y?=w843:bool)
    n237 = Not Equal?(x=w894, y=w897) -> (x != y?=w892:bool)
    n238 = Not Equal?(x=w1158, y=w1155) -> (x != y?=w1160:bool)
    n239 = local read "Road land prod mod"() -> (w1121:dbl)
    n240 = Max & Min(x=w792, y=0.1) -> (max(x,y)=w791:dbl)  [unwired: 1 out]
    n241 = local read "People"() -> (w456:i64)
    n242 = local read "hunting b"() -> (w1543:dbl)
    n243 = local read "hunting b"() -> (w1542:dbl)
    n244 = Compound Arithmetic op=AND(w1177, w1178, w861) -> (w1176:bool)
    n245 = And(x="Barracks\nlevel 0", y=w1176) -> (x .and. y?=w1184:bool)
    n246 = And(x=w1183, y=w1184) -> (x .and. y?=w1182:bool)
    n247 = case shown="True" w1182 {
      tunnel: w1175 -> [_ w1958]
      frame False {
      }
      frame True {
        n248 = local write "Barracks level"(w1958) -> ()
        n249 = local write "Barracks military bonus"(1.0 ("Hut dissent add mod")) -> ()
        n250 = local write "Barracks upkeep"(0.0 ("Hut non-land prod mod")) -> ()
      }
    }
    n251 = Compound Arithmetic op=AND(w875, w874, w849) -> (w876:bool)
    n252 = And(x="Wall level 0", y=w876) -> (x .and. y?=w868:bool)
    n253 = And(x=w869, y=w868) -> (x .and. y?=w870:bool)
    n254 = case shown="True" w870 {
      tunnel: w877 -> [_ w1816]
      frame False {
      }
      frame True {
        n255 = local write "Wall warrior % equivalent"(0.0 ("Hut dissent add mod")) -> ()
        n256 = local write "Walls level"(w1816) -> ()
        n257 = local write "Wall dissent mod"(0.0 ("Hut non-land prod mod")) -> ()
        n258 = local write "Wall upkeep"(0.0 ("Hut non-land prod mod")) -> ()
      }
    }
    n259 = Compound Arithmetic op=AND(w895, w918, w843) -> (w896:bool)
    n260 = And(x="Wall level 2", y=w896) -> (x .and. y?=w891:bool)
    n261 = And(x=w892, y=w891) -> (x .and. y?=w893:bool)
    n262 = case shown="True" w893 {
      tunnel: w897 -> [_ w1834]
      tunnel: w919 -> [_ w1830]
      tunnel: w921 -> [_ w1829]
      frame False {
      }
      frame True {
        n263 = local read "Build points"() -> (w1833:dbl)
        n264 = Add(x=w1830, y=w1829) -> (x+y=w1831:dbl)
        n265 = local write "Wall warrior % equivalent"(4.0 ("Hut dissent add mod")) -> ()
        n266 = local write "Walls level"(w1834) -> ()
        n267 = local write "Wall dissent mod"(-4.0 ("Hut non-land prod mod")) -> ()
        n268 = local write "Wall invested points"(w1831) -> ()
        n269 = local write "Wall upkeep"(0.006 ("Hut non-land prod mod")) -> ()
        n270 = Subtract(x=w1833, y=w1830) -> (x-y=w1832:dbl)
        n271 = local write "Build points"(w1832) -> ()
      }
    }
    n272 = local read "1-Dissent/100"() -> (w1385:dbl)
    n273 = Reciprocal(x=w791) -> (1/x=w788:dbl)
    n274 = case shown="False" "Percentage or absolute" {
      frame False {
        n275 = Add(x="%Hunters", y="%Warriors") -> (x+y=w2547:dbl)
        n276 = Add(x="%Builders", y="%Scientists") -> (x+y=w2548:dbl)
        n277 = Add(x="%Engineers", y="%Crafters") -> (x+y=w2545:dbl)
        n278 = Add(x=w2547, y=w2548) -> (x+y=w2546:dbl)
        n279 = Add(x=w2546, y=w2545) -> (x+y=w2550:dbl)
        n280 = Less Or Equal?(x=w2550, y=100.0) -> (x <= y?=w2551:bool)
        n281 = case shown="True" w2551 {
          tunnel: "%Hunters" -> [_ w2573]
          tunnel: "%Warriors" -> [_ w2572]
          tunnel: "%Builders" -> [_ w2571]
          tunnel: "%Scientists" -> [_ w2570]
          tunnel: "%Engineers" -> [_ w2569]
          tunnel: "%Crafters" -> [_ w2568]
          frame False {
          }
          frame True {
            n282 = local read "People"() -> (w2555:i64)
            n283 = Divide(x=w2555, y=100.0) -> (x/y=w2566:dbl)
            n284 = Multiply(x=w2571, y=w2566) -> (x*y=w2559:dbl)
            n285 = Multiply(x=w2573, y=w2566) -> (x*y=w2553:dbl)
            n286 = Multiply(x=w2572, y=w2566) -> (x*y=w2560:dbl)
            n287 = Multiply(x=w2566, y=w2570) -> (x*y=w2563:dbl)
            n288 = Multiply(x=w2566, y=w2569) -> (x*y=w2562:dbl)
            n289 = Multiply(x=w2566, y=w2568) -> (x*y=w2561:dbl)
            n290 = local write "Scientists"(w2563) -> ()
            n291 = local write "Warriors"(w2560) -> ()
            n292 = local write "Builders"(w2559) -> ()
            n293 = local write "Engineers"(w2562) -> ()
            n294 = local write "Crafters"(w2561) -> ()
            n295 = Add(x=w2553, y=w2560) -> (x+y=w2565:dbl)
            n296 = Add(x=w2563, y=w2562) -> (x+y=w2564:dbl)
            n297 = Add(x=w2565, y=w2559) -> (x+y=w2558:dbl)
            n298 = Add(x=w2564, y=w2561) -> (x+y=w2557:dbl)
            n299 = Add(x=w2558, y=w2557) -> (x+y=w2556:dbl)
            n300 = Subtract(x=w2555, y=w2556) -> (x-y=w2554:dbl)
            n301 = Add(x=w2553, y=w2554) -> (x+y=w2552:dbl)
            n302 = local write "Hunters"(w2552) -> ()
          }
        }
      }
      frame True {
        n303 = local read "Unassigned workers"() -> (w2637:i32)
        n304 = local read "Unassigned workers"() -> (w2646:i32)
        n305 = local read "Unassigned workers"() -> (w2611:i32)
        n306 = local read "Unassigned workers"() -> (w2601:i32)
        n307 = local read "Unassigned workers"() -> (w2630:i32)
        n308 = local read "Unassigned workers"() -> (w2591:i32)
        n309 = local read "Hunters"() -> (w2614:i32)
        n310 = local read "Scientists"() -> (w2602:i32)
        n311 = local read "Engineers"() -> (w2592:i32)
        n312 = local read "Warriors"() -> (w2616:i32)
        n313 = local read "Builders"() -> (w2615:i32)
        n314 = local read "Crafters"() -> (w2582:i32)
        n315 = Greater Or Equal?(x="#Hunters", y=0.0) -> (x >= y?=w2643:bool)
        n316 = Greater Or Equal?(x="#Scientists", y=0.0) -> (x >= y?=w2608:bool)
        n317 = Greater Or Equal?(x="#Warriors", y=0.0) -> (x >= y?=w2634:bool)
        n318 = Greater Or Equal?(x="#Engineers", y=0.0) -> (x >= y?=w2598:bool)
        n319 = Greater Or Equal?(x="#Builders", y=0.0) -> (x >= y?=w2627:bool)
        n320 = Greater Or Equal?(x="#Merchants", y=0.0) -> (x >= y?=w2588:bool)
        n321 = Add(x=w2646, y=w2614) -> (x+y=w2645:i32)
        n322 = Add(x=w2611, y=w2602) -> (x+y=w2610:i32)
        n323 = Add(x=w2637, y=w2616) -> (x+y=w2636:i32)
        n324 = Add(x=w2601, y=w2592) -> (x+y=w2600:i32)
        n325 = Add(x=w2630, y=w2615) -> (x+y=w2629:i32)
        n326 = Add(x=w2591, y=w2582) -> (x+y=w2590:i32)
        n327 = Greater Or Equal?(x=w2645, y="#Hunters") -> (x >= y?=w2642:bool)
        n328 = Greater Or Equal?(x=w2610, y="#Scientists") -> (x >= y?=w2607:bool)
        n329 = Greater Or Equal?(x=w2636, y="#Warriors") -> (x >= y?=w2633:bool)
        n330 = Greater Or Equal?(x=w2600, y="#Engineers") -> (x >= y?=w2597:bool)
        n331 = Greater Or Equal?(x=w2629, y="#Builders") -> (x >= y?=w2626:bool)
        n332 = Greater Or Equal?(x=w2590, y="#Merchants") -> (x >= y?=w2587:bool)
        n333 = And(x=w2642, y=w2643) -> (x .and. y?=w2641:bool)
        n334 = And(x=w2607, y=w2608) -> (x .and. y?=w2606:bool)
        n335 = And(x=w2633, y=w2634) -> (x .and. y?=w2632:bool)
        n336 = And(x=w2597, y=w2598) -> (x .and. y?=w2596:bool)
        n337 = And(x=w2626, y=w2627) -> (x .and. y?=w2625:bool)
        n338 = And(x=w2587, y=w2588) -> (x .and. y?=w2586:bool)
        n339 = And(x=w2641, y="Assign Hunters") -> (x .and. y?=w2639:bool)
        n340 = And(x=w2606, y="Assign Scientist") -> (x .and. y?=w2604:bool)
        n341 = And(x=w2632, y="Assign Warrior") -> (x .and. y?=w2631:bool)
        n342 = And(x=w2596, y="Assign Engineer") -> (x .and. y?=w2594:bool)
        n343 = And(x=w2625, y="Assign Builder") -> (x .and. y?=w2624:bool)
        n344 = And(x=w2586, y="Assign Merchant") -> (x .and. y?=w2584:bool)
        n345 = case shown="True" w2639 {
          tunnel: "#Hunters" -> [_ w2658]
          tunnel: [w2657 w2658] -> w2622
          tunnel: w2614 -> [w2657 _]
          frame False {
          }
          frame True {
            n346 = local write "Hunters"(w2658) -> ()
          }
        }
        n347 = case shown="True" w2604 {
          tunnel: "#Scientists" -> [_ w2652]
          tunnel: [w2651 w2652] -> w2579
          tunnel: w2602 -> [w2651 _]
          frame False {
          }
          frame True {
            n348 = local write "Scientists"(w2652) -> ()
          }
        }
        n349 = case shown="True" w2631 {
          tunnel: "#Warriors" -> [_ w2656]
          tunnel: [w2655 w2656] -> w2617
          tunnel: w2616 -> [w2655 _]
          frame False {
          }
          frame True {
            n350 = local write "Warriors"(w2656) -> ()
          }
        }
        n351 = case shown="True" w2594 {
          tunnel: "#Engineers" -> [_ w2650]
          tunnel: [w2649 w2650] -> w2578
          tunnel: w2592 -> [w2649 _]
          frame False {
          }
          frame True {
            n352 = local write "Engineers"(w2650) -> ()
          }
        }
        n353 = case shown="True" w2624 {
          tunnel: "#Builders" -> [_ w2654]
          tunnel: [w2653 w2654] -> w2580
          tunnel: w2615 -> [w2653 _]
          frame False {
          }
          frame True {
            n354 = local write "Builders"(w2654) -> ()
          }
        }
        n355 = case shown="True" w2584 {
          tunnel: "#Merchants" -> [_ w2648]
          tunnel: [w2647 w2648] -> w2577
          tunnel: w2582 -> [w2647 _]
          frame False {
          }
          frame True {
            n356 = local write "Crafters"(w2648) -> ()
          }
        }
        n357 = local read "People"() -> (w2619:i64)
        n358 = Add(x=w2578, y=w2577) -> (x+y=w2576:dbl)
        n359 = Add(x=w2580, y=w2579) -> (x+y=w2575:dbl)
        n360 = Add(x=w2622, y=w2617) -> (x+y=w2621:dbl)
        n361 = Add(x=w2575, y=w2576) -> (x+y=w2574:dbl)
        n362 = Add(x=w2621, y=w2574) -> (x+y=w2620:dbl)
        n363 = Subtract(x=w2619, y=w2620) -> (x-y=w2618:dbl)
        n364 = local write "Unassigned workers"(w2618) -> ()
      }
    }
    n365 = local read "Military\nScience level"() -> (w846:i32)
    n366 = local read "Permanent\nland"() -> (w1250:dbl)
    n367 = local read "Biology\nlevel"() -> (w1220:i32)
    n368 = local read "Food"() -> (w1541:dbl)
    n369 = Multiply(x=w456, y=w455) -> (x*y=w453:dbl)
    n370 = local read "Hunters"() -> (w1386:i32)
    n371 = Greater Or Equal?(x=w857, y=2) -> (x >= y?=w855:bool)
    n372 = Compound Arithmetic op=AND(w1157, w1039, w855) -> (w1156:bool)
    n373 = And(x="Barracks\nlevel 2", y=w1156) -> (x .and. y?=w1161:bool)
    n374 = And(x=w1160, y=w1161) -> (x .and. y?=w1159:bool)
    n375 = case shown="True" w1159 {
      tunnel: w1155 -> [_ w1974]
      tunnel: w1038 -> [_ w1970]
      tunnel: w1036 -> [_ w1969]
      frame False {
      }
      frame True {
        n376 = local read "Build points"() -> (w1973:dbl)
        n377 = Add(x=w1970, y=w1969) -> (x+y=w1971:dbl)
        n378 = local write "Barracks level"(w1974) -> ()
        n379 = local write "Barracks military bonus"(1.2 ("Hut dissent add mod")) -> ()
        n380 = local write "Barracks\ninvested points"(w1971) -> ()
        n381 = local write "Barracks upkeep"(0.003 ("Hut non-land prod mod")) -> ()
        n382 = Subtract(x=w1973, y=w1970) -> (x-y=w1972:dbl)
        n383 = local write "Build points"(w1972) -> ()
      }
    }
    n384 = Multiply(x=w788, y=1000.0) -> (x*y=w790:dbl)
    n385 = local read "hunting a"() -> (w1540:dbl)
    n386 = local read "Military\nScience level"() -> (w859:i32)
    n387 = local read "Barracks\ninvested points"() -> (w1037:dbl)
    n388 = local read "Wall invested points"() -> (w920:dbl)
    n389 = Wait (ms)(milliseconds to wait=w790) -> ()  [unwired: 1 out]
    n390 = Greater Or Equal?(x=w846, y=2) -> (x >= y?=w847:bool)
    n391 = Compound Arithmetic op=MULTIPLY(w1386, w1121, w1385) -> (w1384:dbl)
    n392 = Power Of X(1:1.05 ("x"), 2:w1220) -> (0:w451:dbl)
    n393 = local read "1-Dissent/100"() -> (w1391:dbl)
    n394 = local read "Barracks\ninvested points"() -> (w1029:dbl)
    n395 = local read "Wall invested points"() -> (w928:dbl)
    n396 = local read "hunting a"() -> (w1392:dbl)
    n397 = Multiply(x=w1250, y=w1543) -> (x*y=w1562:dbl)
    n398 = local read "Governance\nlevel"() -> (w458:i32)
    n399 = local read "Construction\nlevel"() -> (w906:i32)
    n400 = Multiply(x=w1540, y=w1384) -> (x*y=w1553:dbl)
    n401 = local read "Food consumption\nmultiplier"() -> (w463:dbl)
    n402 = Multiply(x=w1562, y=5) -> (x*y=w1560:dbl)
    n403 = local read "Build points"() -> (w1046:dbl)
    n404 = local read "Build points"() -> (w911:dbl)
    n405 = local read "Construction\nlevel"() -> (w1146:i32)
    n406 = Multiply(x=w1553, y=0.1 ("x")) -> (x*y=w1565:dbl)
    n407 = Subtract(x=100000 ("y"), y=w1037) -> (x-y=w1049:dbl)
    n408 = Subtract(x=1000000 ("y"), y=w920) -> (x-y=w908:dbl)
    n409 = local read "Wall warrior % equivalent"() -> (w804:dbl)
    n410 = Multiply(x=w1392, y=w1391) -> (x*y=w1390:dbl)
    n411 = Quotient & Remainder(x=w1560, y=w1390) -> (floor(x/y)=→"Max hunters":dbl)  [unwired: 1 out]
    n412 = local read "Construction\nlevel"() -> (w886:i32)
    n413 = local read "Construction\nlevel"() -> (w1166:i32)
    n414 = local read "Build points"() -> (w922:dbl)
    n415 = local read "Barracks level"() -> (w1151:i32)
    n416 = Divide(x=w1565, y=w1250) -> (x/y=w1564:dbl)
    n417 = local read "Walls level"() -> (w881:i32)
    n418 = local read "Barracks level"() -> (w1171:i32)
    n419 = local read "Build points"() -> (w1035:dbl)
    n420 = local read "Walls level"() -> (w901:i32)
    n421 = Greater Or Equal?(x=w859, y=2) -> (x >= y?=w858:bool)
    n422 = Greater Or Equal?(x=w1146, y=2) -> (x >= y?=w1152:bool)
    n423 = Subtract(x=10000000 ("y"), y=w928) -> (x-y=w925:dbl)
    n424 = Max & Min(x=w1049, y=0.0) -> (max(x,y)=w1044:dbl)  [unwired: 1 out]
    n425 = Max & Min(x=w908, y=0.0) -> (max(x,y)=w913:dbl)  [unwired: 1 out]
    n426 = Multiply(x=100, y="# people") -> (x*y=w1525:i32)
    n427 = Subtract(x=1000000 ("y"), y=w1029) -> (x-y=w1032:dbl)
    n428 = Subtract(x=w1542, y=w1564) -> (x-y=w1563:dbl)
    n429 = local read "Conquered\nland"() -> (w1249:dbl)
    n430 = Greater Or Equal?(x=w1046, y=w1044) -> (x >= y?=w1045:bool)
    n431 = Greater Or Equal?(x=w911, y=w913) -> (x >= y?=w912:bool)
    n432 = Multiply(x=w1553, y=w1563) -> (x*y=w1552:dbl)
    n433 = local read "Farming level"() -> (w1218:i32)
    n434 = local read "Trading level"() -> (w1119:i32)
    n435 = local read "Road land prod mod"() -> (w1120:dbl)
    n436 = Max & Min(x=w925, y=0.0) -> (max(x,y)=w927:dbl)  [unwired: 1 out]
    n437 = Greater Or Equal?(x=w458, y=2) -> (x >= y?=w482:bool)
    n438 = And(x="Higher food\nconsumption", y=w482) -> (x .and. y?=w460:bool)
    n439 = Max & Min(x=w1032, y=0.0) -> (max(x,y)=w1030:dbl)  [unwired: 1 out]
    n440 = Greater Or Equal?(x=w922, y=w927) -> (x >= y?=w926:bool)
    n441 = Greater Or Equal?(x=w886, y=3) -> (x >= y?=w880:bool)
    n442 = Greater Or Equal?(x=w1035, y=w1030) -> (x >= y?=w1031:bool)
    n443 = Greater Or Equal?(x=w906, y=3) -> (x >= y?=w900:bool)
    n444 = Compound Arithmetic op=AND(w1152, w1045, w858) -> (w1153:bool)
    n445 = And(x="Barracks\nlevel 1", y=w1153) -> (x .and. y?=w1148:bool)
    n446 = Compound Arithmetic op=AND(w900, w912, w847) -> (w899:bool)
    n447 = And(x="Wall level 1", y=w899) -> (x .and. y?=w904:bool)
    n448 = Greater Or Equal?(x=w1166, y=2) -> (x >= y?=w1172:bool)
    n449 = Not Equal?(x=w463, y=w464) -> (x != y?=w461:bool)
    n450 = And(x=w461, y=w460) -> (x .and. y?=w462:bool)
    n451 = Not Equal?(x=w881, y=w878) -> (x != y?=w883:bool)
    n452 = Not Equal?(x=w1151, y=w1154) -> (x != y?=w1149:bool)
    n453 = And(x=w1149, y=w1148) -> (x .and. y?=w1150:bool)
    n454 = Not Equal?(x=w901, y=w898) -> (x != y?=w903:bool)
    n455 = And(x=w903, y=w904) -> (x .and. y?=w902:bool)
    n456 = Not Equal?(x=w1171, y=w1174) -> (x != y?=w1169:bool)
    n457 = case shown="True" w462 {
      tunnel: w464 -> [_ w1669]
      frame False {
      }
      frame True {
        n458 = local write "Food consumption\nmultiplier"(w1669) -> ()
        n459 = local write "Food dissent mod"(-5.0 ("Taxes dissent add mod")) -> ()
      }
    }
    n460 = local read "1-Dissent/100"() -> (w1388:dbl)
    n461 = local read "Military\nScience level"() -> (w842:i32)
    n462 = Multiply(x=w1119, y=0.5) -> (x*y=w1118:dbl)
    n463 = Increment(x=w1218) -> (x+1=w1216:i32)
    n464 = local read "Military\nScience level"() -> (w853:i32)
    n465 = case shown="True" w1150 {
      tunnel: w1154 -> [_ w1982]
      tunnel: w1037 -> [_ w1979]
      tunnel: w1044 -> [_ w1977]
      frame False {
      }
      frame True {
        n466 = local read "Build points"() -> (w1981:dbl)
        n467 = Add(x=w1977, y=w1979) -> (x+y=w1978:dbl)
        n468 = local write "Barracks level"(w1982) -> ()
        n469 = local write "Barracks military bonus"(1.1 ("Hut dissent add mod")) -> ()
        n470 = local write "Barracks\ninvested points"(w1978) -> ()
        n471 = local write "Barracks upkeep"(0.001 ("Hut non-land prod mod")) -> ()
        n472 = Subtract(x=w1981, y=w1977) -> (x-y=w1980:dbl)
        n473 = local write "Build points"(w1980) -> ()
      }
    }
    n474 = case shown="True" w902 {
      tunnel: w898 -> [_ w1843]
      tunnel: w920 -> [_ w1840]
      tunnel: w913 -> [_ w1838]
      frame False {
      }
      frame True {
        n475 = local read "Build points"() -> (w1842:dbl)
        n476 = Add(x=w1838, y=w1840) -> (x+y=w1839:dbl)
        n477 = local write "Walls level"(w1843) -> ()
        n478 = local write "Wall warrior % equivalent"(2.0 ("Hut dissent add mod")) -> ()
        n479 = local write "Wall invested points"(w1839) -> ()
        n480 = local write "Wall dissent mod"(-2.0 ("Hut non-land prod mod")) -> ()
        n481 = Subtract(x=w1842, y=w1838) -> (x-y=w1841:dbl)
        n482 = local write "Wall upkeep"(0.002 ("Hut non-land prod mod")) -> ()
        n483 = local write "Build points"(w1841) -> ()
      }
    }
    n484 = local read "Warriors"() -> (w807:i32)
    n485 = Increment(x=w1118) -> (x+1=w1217:dbl)
    n486 = local read "warrior a"() -> (w1389:dbl)
    n487 = Compound Arithmetic op=MULTIPLY(w1249, w1216, w1217) -> (w452:dbl)
    n488 = Add(x=w1552, y=w452) -> (x+y=w450:dbl)
    n489 = Multiply(x=w451, y=w450) -> (x*y=w449:dbl)
    n490 = Subtract(x=w449, y=w453) -> (x-y=w454:dbl)
    "Food/s" <- w454
    n491 = Add(x=w1541, y=w454) -> (x+y=w1524:dbl)
    n492 = Greater?(x=w1524, y=w1525) -> (0:w1528:bool)
    n493 = And(x=w1528, y="Increase\nPopulation") -> (x .and. y?=w1527:bool)
    n494 = case shown="False" w1527 {
      tunnel: w456 -> [_ w2702]
      tunnel: w1525 -> [_ w2700]
      tunnel: w1524 -> [w2684 w2699]
      tunnel: [w2683 w2698] -> w1522
      tunnel: "# people" -> [_ w2697]
      frame False {
        n495 = Less?(x=w2684, y=-100.0) -> (x < y?=w2686:bool)
        n496 = case shown="True" w2686 {
          tunnel: w2684 -> [w2687 w2691]
          tunnel: [w2687 w2688] -> w2683
          frame False {
          }
          frame True {
            n497 = local read "People"() -> (w2689:i64)
            n498 = Quotient & Remainder(x=w2691, y=100.0) -> (floor(x/y)=w2695:dbl)  [unwired: 1 out]
            n499 = Increment(x=w2695) -> (x+1=w2692:dbl)
            n500 = Add(x=w2689, y=w2692) -> (x+y=w2694:dbl)
            n501 = local write "People"(w2694) -> ()
            n502 = Multiply(x=w2692, y=-50.0) -> (x*y=w2690:dbl)
            n503 = Add(x=w2690, y=w2691) -> (x+y=w2688:dbl)
          }
        }
      }
      frame True {
        n504 = Add(x=w2702, y=w2697) -> (x+y=w2701:i64)
        n505 = Subtract(x=w2699, y=w2700) -> (x-y=w2698:dbl)
        n506 = local write "People"(w2701) -> ()
      }
    }
    n507 = Compound Arithmetic op=MULTIPLY(w456, 0.01 ("value"), w804) -> (w803:dbl)
    n508 = local write "food income"(w449) -> ()
    n509 = Greater Or Equal?(x=w842, y=2) -> (x >= y?=w840:bool)
    n510 = Compound Arithmetic op=AND(w880, w926, w840) -> (w879:bool)
    n511 = And(x="Wall level 3", y=w879) -> (x .and. y?=w884:bool)
    n512 = And(x=w883, y=w884) -> (x .and. y?=w882:bool)
    n513 = case shown="True" w882 {
      tunnel: w878 -> [_ w1825]
      tunnel: w927 -> [_ w1821]
      tunnel: w928 -> [_ w1820]
      frame False {
      }
      frame True {
        n514 = local read "Build points"() -> (w1824:dbl)
        n515 = Add(x=w1821, y=w1820) -> (x+y=w1822:dbl)
        n516 = local write "Walls level"(w1825) -> ()
        n517 = local write "Wall warrior % equivalent"(6.0 ("Hut dissent add mod")) -> ()
        n518 = local write "Wall invested points"(w1822) -> ()
        n519 = local write "Wall dissent mod"(-6.0 ("Hut non-land prod mod")) -> ()
        n520 = Subtract(x=w1824, y=w1821) -> (x-y=w1823:dbl)
        n521 = local write "Wall upkeep"(0.02 ("Hut non-land prod mod")) -> ()
        n522 = local write "Build points"(w1823) -> ()
      }
    }
    n523 = Add(x=w803, y=w807) -> (x+y=w806:dbl)
    n524 = Compound Arithmetic op=MULTIPLY(w1389, w1120, w1388) -> (w1387:dbl)
    n525 = Multiply(x=w806, y=w1387) -> (x*y=w1559:dbl)
    n526 = local read "School invested points"() -> (w641:dbl)
    n527 = Greater Or Equal?(x=w853, y=2) -> (x >= y?=w852:bool)
    n528 = Compound Arithmetic op=AND(w1172, w1031, w852) -> (w1173:bool)
    n529 = And(x="Barracks\nlevel 3", y=w1173) -> (x .and. y?=w1168:bool)
    n530 = And(x=w1169, y=w1168) -> (x .and. y?=w1170:bool)
    n531 = case shown="True" w1170 {
      tunnel: w1174 -> [_ w1966]
      tunnel: w1030 -> [_ w1962]
      tunnel: w1029 -> [_ w1961]
      frame False {
      }
      frame True {
        n532 = local read "Build points"() -> (w1965:dbl)
        n533 = Add(x=w1962, y=w1961) -> (x+y=w1963:dbl)
        n534 = local write "Barracks level"(w1966) -> ()
        n535 = local write "Barracks\ninvested points"(w1963) -> ()
        n536 = local write "Barracks military bonus"(1.3 ("Hut dissent add mod")) -> ()
        n537 = local write "Barracks upkeep"(0.01 ("Hut non-land prod mod")) -> ()
        n538 = Subtract(x=w1965, y=w1962) -> (x-y=w1964:dbl)
        n539 = local write "Build points"(w1964) -> ()
      }
    }
    n540 = local read "Barracks military bonus"() -> (w864:dbl)
    n541 = local read "warrior c"() -> (w1535:dbl)
    n542 = local read "Warrior b Gov mult"() -> (w1315:dbl)
    n543 = local read "Construction\nlevel"() -> (w673:i32)
    n544 = Add(x=w1559, y=50.0) -> (x+y=w1557:dbl)
    n545 = local read "Hut invested points"() -> (w1058:dbl)
    n546 = local read "Construction\nlevel"() -> (w696:i32)
    n547 = for {
      tunnel: w1144 -> [w2036] mode=indexing
      # "Construction upkeep"
      n548 = local read "Road upkeep"() -> (w2041:dbl)
      n549 = local read "Gov building\nupkeep mod"() -> (w2037:dbl)
      n550 = local read "Hut upkeep"() -> (w2042:dbl)
      n551 = local read "Barracks upkeep"() -> (w2035:dbl)
      n552 = local read "University upkeep"() -> (w2008:dbl)
      n553 = local read "School upkeep"() -> (w2009:dbl)
      n554 = local read "Construction\nlevel"() -> (w2046:i32)
      n555 = local read "Wall upkeep"() -> (w2034:dbl)
      n556 = local read "Build points"() -> (w2052:dbl)
      n557 = Compound Arithmetic op=ADD(w2042, w2041) -> (w2040:dbl)
      n558 = Compound Arithmetic op=ADD(w2035, w2034, w2009, w2008) -> (w2033:dbl)
      n559 = Multiply(x=w2036, y=w2040) -> (x*y=w2039:dbl)
      n560 = Multiply(x=0.05, y=w2046) -> (x*y=w2045:dbl)
      n561 = Multiply(x=w2036, y=w2033) -> (x*y=w2032:dbl)
      n562 = Subtract(x=1.0, y=w2045) -> (x-y=w2038:dbl)
      n563 = Compound Arithmetic op=MULTIPLY(w2039, w2038, w2037) -> (w2023:dbl)
      n564 = Subtract(x=w2052, y=w2023) -> (x-y=w2044:dbl)
      n565 = Compound Arithmetic op=MULTIPLY(w2038, w2037, w2032) -> (w2029:dbl)
      n566 = local read "Gold"() -> (w2031:dbl)
      n567 = local write "Build points"(w2044) -> ()
      n568 = local write "BP upkeep"(w2023) -> ()
      n569 = local write "Gold upkeep"(w2029) -> ()
      n570 = Subtract(x=w2031, y=w2029) -> (x-y=w2030:dbl)
      n571 = local write "Gold"(w2030) -> ()
      n572 = local read "School dissent mod"() -> (w2022:dbl)
      n573 = local read "-dissent per\nmilitary building"() -> (w2020:dbl)
      n574 = local read "Barracks level"() -> (w2018:i32)
      n575 = local read "Walls level"() -> (w2019:i32)
      n576 = local read "Gov elitist\nbuildings mod"() -> (w2011:dbl)
      n577 = local read "University dissent mod"() -> (w2013:dbl)
      n578 = local read "Taxes dissent mod"() -> (w2028:dbl)
      n579 = local read "Hut dissent mod"() -> (w2043:dbl)
      n580 = local read "Medicine dissent mod"() -> (w2004:i32)
      n581 = local read "Gov populist\nbuildings mod"() -> (w2026:dbl)
      n582 = local read "Wall dissent mod"() -> (w2021:dbl)
      n583 = Compound Arithmetic op=ADD(0.0 ("value"), w2013) -> (w2012:dbl)
      n584 = Compound Arithmetic op=ADD(w2019, w2018) -> (w2017:i32)
      n585 = Compound Arithmetic op=ADD(w2043, w2022) -> (w2027:dbl)
      n586 = Multiply(x=w2011, y=w2012) -> (x*y=w2010:dbl)
      n587 = Multiply(x=w2020, y=w2017) -> (x*y=w2016:dbl)
      n588 = Multiply(x=w2026, y=w2027) -> (x*y=w2025:dbl)
      n589 = Negate(x=w2016) -> (-x=w2015:dbl)
      n590 = local read "Writing level"() -> (w2000:i32)
      n591 = local read "School SP/EP multiplier"() -> (w2003:dbl)
      n592 = local read "Trading level no mod"() -> (w2051:i32)
      n593 = local read "Food dissent mod"() -> (w2007:dbl)
      n594 = Compound Arithmetic op=ADD(w2025, w2004, w2007, w2028, w2021, w2015, w2010) -> (w2024:dbl)
      n595 = local read "Hut non-land prod mod"() -> (w2006:dbl)
      n596 = local read "Road level"() -> (w2050:i32)
      n597 = Power Of X(1:1.1 ("x"), 2:w2000) -> (0:w1999:dbl)
      n598 = local write "Dissent addition modifiers"(w2024) -> ()
      n599 = Add(x=w2051, y=w2050) -> (x+y=w2049:i32)
      n600 = Compound Arithmetic op=MULTIPLY(w2003, w1999) -> (w2002:dbl)
      n601 = Compound Arithmetic op=ADD(w2006) -> (w2005:dbl)
      n602 = local write "Non-land production multiplier"(w2005) -> ()
      n603 = local write "SP/EP multiplier"(w2002) -> ()
      n604 = local write "Trading level"(w2049) -> ()
    }
    n605 = local read "Build points"() -> (w645:dbl)
    n606 = Reciprocal(x=w1535) -> (1/x=w1534:dbl)
    n607 = local read "Road invested points"() -> (w985:dbl)
    n608 = local read "Governance\nlevel"() -> (w699:i32)
    n609 = local read "School level"() -> (w691:i32)
    n610 = local read "School level"() -> (w668:i32)
    n611 = local read "Build points"() -> (w690:dbl)
    n612 = local read "Conquered\nland"() -> (w1537:dbl)
    n613 = Subtract(x=600000 ("y"), y=w641) -> (x-y=w648:dbl)
    n614 = local read "Governance\nlevel"() -> (w705:i32)
    n615 = local read "warrior b"() -> (w1316:dbl)
    n616 = Power Of X(1:w1557, 2:w1534) -> (0:w1554:dbl)
    n617 = Square Root(x=50.0) -> (sqrt(x)=w1555:dbl)
    n618 = local read "Economics\nlevel"() -> (w1014:i32)
    n619 = local read "Construction\nlevel"() -> (w953:i32)
    n620 = local read "Construction\nlevel"() -> (w1189:i32)
    n621 = Max & Min(x=w648, y=0.0) -> (max(x,y)=w643:dbl)  [unwired: 1 out]
    n622 = local read "Construction\nlevel"() -> (w1133:i32)
    n623 = Multiply(x=w1522, y=0.999) -> (x*y=w1521:dbl)
    n624 = Greater Or Equal?(x=w645, y=w643) -> (x >= y?=w644:bool)
    n625 = Subtract(x=w1554, y=w1555) -> (x-y=w1312:dbl)
    n626 = local read "Build points"() -> (w1060:dbl)
    n627 = local read "Taxation\nlevel"() -> (w1003:dbl)
    n628 = local read "Economics\nlevel"() -> (w998:i32)
    n629 = local read "Hut level"() -> (w1194:i32)
    n630 = Greater Or Equal?(x=w696, y=2) -> (x >= y?=w687:bool)
    n631 = local read "Hut level"() -> (w1136:i32)
    n632 = Greater Or Equal?(x=w690, y=0) -> (x >= y?=w688:bool)
    n633 = local read "Taxation\nlevel"() -> (w1019:dbl)
    n634 = Greater Or Equal?(x=w673, y=3) -> (x >= y?=w667:bool)
    n635 = local write "Food"(w1521) -> ()
    n636 = local read "Military Modifier"() -> (w1314:dbl)
    n637 = Greater Or Equal?(x=w699, y=2) -> (x >= y?=w700:bool)
    n638 = local read "Build points"() -> (w981:dbl)
    n639 = local read "Construction\nlevel"() -> (w930:i32)
    n640 = Subtract(x=30000 ("y"), y=w1058) -> (x-y=w1063:dbl)
    n641 = Not Equal?(x=w691, y=w685) -> (x != y?=w693:bool)
    n642 = Greater Or Equal?(x=w705, y=2) -> (x >= y?=w706:bool)
    n643 = local read "Road level"() -> (w958:i32)
    n644 = Not Equal?(x=w668, y=w665) -> (x != y?=w670:bool)
    n645 = local read "Road level"() -> (w935:i32)
    n646 = Subtract(x=150000 ("y"), y=w985) -> (x-y=w978:dbl)
    n647 = local read "Build points"() -> (w936:dbl)
    n648 = Compound Arithmetic op=MULTIPLY(w1314, w864, w1315, w1316, 0.064789, 2.0 ("y"), w1312) -> (w1313:dbl)
    n649 = Add(x=w1313, y=w1537) -> (x+y=w1533:dbl)
    n650 = Max & Min(x=w1063, y=0.0) -> (max(x,y)=w1057:dbl)  [unwired: 1 out]
    n651 = Greater Or Equal?(x=w1189, y=1) -> (x >= y?=w1143:bool)
    n652 = Greater Or Equal?(x=w1060, y=w1057) -> (x >= y?=w1059:bool)
    n653 = And(x="Hut level 0", y=w1143) -> (x .and. y?=w1191:bool)
    n654 = Compound Arithmetic op=AND(w687, w688, w700) -> (w686:bool)
    n655 = And(x="School\nlevel 0", y=w686) -> (x .and. y?=w694:bool)
    n656 = And(x=w693, y=w694) -> (x .and. y?=w692:bool)
    n657 = case shown="True" w692 {
      tunnel: w685 -> [_ w1737]
      frame False {
      }
      frame True {
        n658 = local write "School engineer equivalent"(0.0 ("Hut dissent add mod")) -> ()
        n659 = local write "School level"(w1737) -> ()
        n660 = local write "School SP/EP multiplier"(1.0 ("Hut non-land prod mod")) -> ()
        n661 = local write "School dissent mod"(0.0 ("Hut non-land prod mod")) -> ()
        n662 = local write "School upkeep"(0.0 ("Hut non-land prod mod")) -> ()
      }
    }
    n663 = Greater Or Equal?(x=w1133, y=1) -> (x >= y?=w1139:bool)
    n664 = Compound Arithmetic op=AND(w667, w644, w706) -> (w666:bool)
    n665 = And(x="School\nlevel 2", y=w666) -> (x .and. y?=w671:bool)
    n666 = And(x=w670, y=w671) -> (x .and. y?=w669:bool)
    n667 = Max & Min(x=w978, y=0.0) -> (max(x,y)=w983:dbl)  [unwired: 1 out]
    n668 = Greater Or Equal?(x=w998, y=1) -> (x >= y?=w996:bool)
    n669 = And(x="Taxes level 0", y=w996) -> (x .and. y?=w1000:bool)
    n670 = Greater Or Equal?(x=w981, y=w983) -> (x >= y?=w982:bool)
    n671 = Not Equal?(x=w1194, y=w1195) -> (x != y?=w1192:bool)
    n672 = And(x=w1192, y=w1191) -> (x .and. y?=w1193:bool)
    n673 = Greater Or Equal?(x=w1014, y=1) -> (x >= y?=w993:bool)
    n674 = And(x="Taxes level 2", y=w993) -> (x .and. y?=w1016:bool)
    n675 = Not Equal?(x=w1136, y=w1137) -> (x != y?=w1134:bool)
    n676 = Compound Arithmetic op=AND(w1134, "Hut level 2", w1139, w1059) -> (w1135:bool)
    n677 = Quotient & Remainder(x=w1520, y=365.0) -> (x-y*floor(x/y)=→"Day":dbl, floor(x/y)=→"Year":dbl)
    n678 = Greater Or Equal?(x=w953, y=1) -> (x >= y?=w959:bool)
    n679 = Not Equal?(x=w1003, y=w1004) -> (x != y?=w1001:bool)
    n680 = And(x=w1001, y=w1000) -> (x .and. y?=w1002:bool)
    n681 = Greater Or Equal?(x=w930, y=1) -> (x >= y?=w939:bool)
    n682 = Greater Or Equal?(x=w936, y=0) -> (x >= y?=w938:bool)
    n683 = local read "Governance\nlevel"() -> (w703:i32)
    n684 = local read "Gov populist\nbuildings mod"() -> (w562:dbl)
    n685 = Not Equal?(x=w1019, y=w1020) -> (x != y?=w1017:bool)
    n686 = And(x=w1017, y=w1016) -> (x .and. y?=w1018:bool)
    n687 = case shown="True" w1135 {
      tunnel: w1137 -> [_ w1955]
      tunnel: w1058 -> [_ w1950]
      tunnel: w1057 -> [_ w1949]
      tunnel: w562 -> [_ w1945]
      frame False {
      }
      frame True {
        n688 = local read "Build points"() -> (w1954:dbl)
        n689 = Multiply(x=w1945, y=0.2) -> (x*y=w1947:dbl)
        n690 = Add(x=w1949, y=w1950) -> (x+y=w1951:dbl)
        n691 = local write "Hut level"(w1955) -> ()
        n692 = Increment(x=w1947) -> (x+1=w1948:dbl)
        n693 = local write "Hut upkeep"(0.03 ("Hut dissent add mod")) -> ()
        n694 = local write "Hut non-land prod mod"(w1948) -> ()
        n695 = Subtract(x=w1954, y=w1949) -> (x-y=w1953:dbl)
        n696 = local write "Hut invested points"(w1951) -> ()
        n697 = local write "Hut dissent mod"(-4.0 ("Hut dissent add mod")) -> ()
        n698 = local write "Build points"(w1953) -> ()
      }
    }
    n699 = local read "Permanent\nland"() -> (w1548:dbl)
    n700 = Not Equal?(x=w958, y=w961) -> (x != y?=w956:bool)
    n701 = case shown="True" w1193 {
      tunnel: w1195 -> [_ w1986]
      frame False {
      }
      frame True {
        n702 = local write "Hut non-land prod mod"(1.0 ("Hut non-land prod mod")) -> ()
        n703 = local write "Hut dissent mod"(0.0 ("Hut dissent add mod")) -> ()
        n704 = local write "Hut level"(w1986) -> ()
        n705 = local write "Hut upkeep"(0.0 ("Hut dissent add mod")) -> ()
      }
    }
    n706 = Not Equal?(x=w935, y=w941) -> (x != y?=w933:bool)
    n707 = local read "Gov populist\nbuildings mod"() -> (w561:dbl)
    n708 = case shown="True" w669 {
      tunnel: w665 -> [_ w1763]
      tunnel: w643 -> [_ w1759]
      tunnel: w641 -> [_ w1758]
      tunnel: w561 -> [_ w1751]
      frame False {
      }
      frame True {
        n709 = Multiply(x=w1751, y=0.1) -> (x*y=w1754:dbl)
        n710 = Increment(x=w1754) -> (x+1=w1753:dbl)
        n711 = local read "Build points"() -> (w1762:dbl)
        n712 = Add(x=w1759, y=w1758) -> (x+y=w1760:dbl)
        n713 = local write "School engineer equivalent"(0.02 ("Hut dissent add mod")) -> ()
        n714 = local write "School level"(w1763) -> ()
        n715 = local write "School dissent mod"(-2.0 ("Hut non-land prod mod")) -> ()
        n716 = local write "School SP/EP multiplier"(w1753) -> ()
        n717 = local write "School invested points"(w1760) -> ()
        n718 = local write "School upkeep"(0.003 ("Hut non-land prod mod")) -> ()
        n719 = Subtract(x=w1762, y=w1759) -> (x-y=w1761:dbl)
        n720 = local write "Build points"(w1761) -> ()
      }
    }
    n721 = case shown="True" w1002 {
      tunnel: w1004 -> [_ w1876]
      frame False {
      }
      frame True {
        n722 = local write "Taxation\nlevel"(w1876) -> ()
        n723 = local write "Taxes dissent mod"(0.0 ("Taxes dissent add mod")) -> ()
      }
    }
    n724 = case shown="True" w1018 {
      tunnel: w1020 -> [_ w1880]
      frame False {
      }
      frame True {
        n725 = local write "Taxation\nlevel"(w1880) -> ()
        n726 = local write "Taxes dissent mod"(8.0 ("Taxes dissent add mod")) -> ()
      }
    }
    n727 = local read "School invested points"() -> (w642:dbl)
    n728 = local read "People"() -> (w1550:i64)
    n729 = And(x=w959, y=w982) -> (x .and. y?=w960:bool)
    n730 = And(x="Road level 2", y=w960) -> (x .and. y?=w955:bool)
    n731 = And(x=w956, y=w955) -> (x .and. y?=w957:bool)
    n732 = case shown="True" w957 {
      tunnel: w961 -> [_ w1865]
      tunnel: w983 -> [_ w1858]
      tunnel: w985 -> [_ w1857]
      frame False {
      }
      frame True {
        n733 = local read "Build points"() -> (w1864:dbl)
        n734 = Add(x=w1858, y=w1857) -> (x+y=w1860:dbl)
        n735 = local write "Road level"(w1865) -> ()
        n736 = local write "Road expansion bonus"(0.5 ("Hut dissent add mod")) -> ()
        n737 = local write "Road land prod mod"(1.2 ("Hut dissent add mod")) -> ()
        n738 = local write "Road invested points"(w1860) -> ()
        n739 = local write "Road upkeep"(0.06 ("Hut non-land prod mod")) -> ()
        n740 = Subtract(x=w1864, y=w1858) -> (x-y=w1863:dbl)
        n741 = local write "Build points"(w1863) -> ()
      }
    }
    n742 = And(x=w939, y=w938) -> (x .and. y?=w940:bool)
    n743 = And(x="Road level 0", y=w940) -> (x .and. y?=w932:bool)
    n744 = And(x=w933, y=w932) -> (x .and. y?=w934:bool)
    n745 = case shown="True" w934 {
      tunnel: w941 -> [_ w1847]
      frame False {
      }
      frame True {
        n746 = local write "Road level"(w1847) -> ()
        n747 = local write "Road expansion bonus"(0.0 ("Hut dissent add mod")) -> ()
        n748 = local write "Road land prod mod"(1.0 ("Hut dissent add mod")) -> ()
        n749 = local write "Road upkeep"(0.0 ("Hut non-land prod mod")) -> ()
      }
    }
    n750 = Greater Or Equal?(x=w703, y=2) -> (x >= y?=w702:bool)
    n751 = local read "School invested points"() -> (w634:dbl)
    n752 = local read "Road expansion bonus"() -> (w1123:dbl)
    n753 = Divide(x=w1550, y=w1548) -> (x/y=w1549:dbl)
    n754 = Divide(x=w1533, y=w1548) -> (x/y=w1547:dbl)
    n755 = Square(x=w1549) -> (x^2=w1546:dbl)
    n756 = Square(x=w1547) -> (x^2=w1545:dbl)
    n757 = local read "Construction\nlevel"() -> (w656:i32)
    n758 = local read "Land conv mult"() -> (w1465:dbl)
    n759 = local read "Road invested points"() -> (w984:dbl)
    n760 = local read "Build points"() -> (w651:dbl)
    n761 = local read "Hut invested points"() -> (w1064:dbl)
    n762 = Subtract(x=200000 ("y"), y=w642) -> (x-y=w654:dbl)
    n763 = local read "Hut invested points"() -> (w1051:dbl)
    n764 = Multiply(x=w1546, y=w1545) -> (x*y=w1531:dbl)
    n765 = local read "Construction\nlevel"() -> (w676:i32)
    n766 = local read "Road invested points"() -> (w992:dbl)
    n767 = local read "Build points"() -> (w640:dbl)
    n768 = local read "School level"() -> (w681:i32)
    n769 = local read "School level"() -> (w661:i32)
    n770 = local read "Economics\nlevel"() -> (w1027:i32)
    n771 = Subtract(x=2000000 ("y"), y=w634) -> (x-y=w637:dbl)
    n772 = Max & Min(x=w654, y=0.0) -> (max(x,y)=w649:dbl)  [unwired: 1 out]
    n773 = Y-th Root of X(1:w1533, 2:4.0 ("y")) -> (0:w1530:dbl)
    n774 = Multiply(x=w1531, y=w1530) -> (x*y=w1464:dbl)
    n775 = Greater Or Equal?(x=w651, y=w649) -> (x >= y?=w650:bool)
    n776 = local read "Construction\nlevel"() -> (w970:i32)
    n777 = local read "Build points"() -> (w975:dbl)
    n778 = local read "Construction\nlevel"() -> (w1201:i32)
    n779 = local read "Economics\nlevel"() -> (w1011:i32)
    n780 = Increment(x=w1123) -> (x+1=w1122:dbl)
    n781 = Compound Arithmetic op=MULTIPLY(w1465, w1122, w1464) -> (w1463:dbl)
    n782 = Multiply(x=w1463, y=1e-05) -> (x*y=w1433:dbl)
    "Land conversion rate" <- w1433
    n783 = Add(x=w1250, y=w1433) -> (x+y=w1539:dbl)
    n784 = local write "Permanent\nland"(w1539) -> ()
    n785 = local read "Construction\nlevel"() -> (w1130:i32)
    n786 = Max & Min(x=w637, y=0.0) -> (max(x,y)=w635:dbl)  [unwired: 1 out]
    n787 = Subtract(x=50000 ("y"), y=w984) -> (x-y=w972:dbl)
    n788 = local read "Build points"() -> (w1197:dbl)
    n789 = local read "Taxation\nlevel"() -> (w1022:dbl)
    n790 = local read "Taxation\nlevel"() -> (w1006:dbl)
    n791 = local read "Hut level"() -> (w1198:i32)
    n792 = Greater Or Equal?(x=w640, y=w635) -> (x >= y?=w636:bool)
    n793 = local read "Build points"() -> (w1056:dbl)
    n794 = local read "Construction\nlevel"() -> (w950:i32)
    n795 = Greater Or Equal?(x=w676, y=3) -> (x >= y?=w682:bool)
    n796 = Greater Or Equal?(x=w656, y=2) -> (x >= y?=w662:bool)
    n797 = local read "Build points"() -> (w986:dbl)
    n798 = Compound Arithmetic op=AND(w662, w650, w702) -> (w663:bool)
    n799 = And(x="School\nlevel 1", y=w663) -> (x .and. y?=w658:bool)
    n800 = Subtract(x=10000 ("y"), y=w1064) -> (x-y=w1066:dbl)
    n801 = local read "Road level"() -> (w945:i32)
    n802 = local read "Hut level"() -> (w1127:i32)
    n803 = Subtract(x=150000 ("y"), y=w1051) -> (x-y=w1053:dbl)
    n804 = Subtract(x=w1533, y=w1433) -> (x-y=w1435:dbl)
    n805 = Not Equal?(x=w681, y=w684) -> (x != y?=w679:bool)
    n806 = local read "Road level"() -> (w965:i32)
    n807 = Not Equal?(x=w661, y=w664) -> (x != y?=w659:bool)
    n808 = And(x=w659, y=w658) -> (x .and. y?=w660:bool)
    n809 = Subtract(x=500000 ("y"), y=w992) -> (x-y=w989:dbl)
    n810 = Max & Min(x=w972, y=0.0) -> (max(x,y)=w977:dbl)  [unwired: 1 out]
    n811 = Greater Or Equal?(x=w975, y=w977) -> (x >= y?=w976:bool)
    n812 = Max & Min(x=w1066, y=0.0) -> (max(x,y)=w1065:dbl)  [unwired: 1 out]
    n813 = local read "Governance\nlevel"() -> (w707:i32)
    n814 = Max & Min(x=w1053, y=0.0) -> (max(x,y)=w1050:dbl)  [unwired: 1 out]
    n815 = Greater Or Equal?(x=w1197, y=w1065) -> (x >= y?=w1140:bool)
    n816 = Greater Or Equal?(x=w1201, y=1) -> (x >= y?=w1141:bool)
    n817 = case shown="True" w660 {
      tunnel: w664 -> [_ w1776]
      tunnel: w642 -> [_ w1773]
      tunnel: w649 -> [_ w1771]
      tunnel: w561 -> [_ w1764]
      frame False {
      }
      frame True {
        n818 = Multiply(x=w1764, y=0.05) -> (x*y=w1766:dbl)
        n819 = Increment(x=w1766) -> (x+1=w1767:dbl)
        n820 = local read "Build points"() -> (w1775:dbl)
        n821 = Add(x=w1771, y=w1773) -> (x+y=w1772:dbl)
        n822 = local write "School level"(w1776) -> ()
        n823 = local write "School engineer equivalent"(0.01 ("Hut dissent add mod")) -> ()
        n824 = local write "School SP/EP multiplier"(w1767) -> ()
        n825 = local write "School invested points"(w1772) -> ()
        n826 = local write "School dissent mod"(-1.0 ("Hut non-land prod mod")) -> ()
        n827 = Subtract(x=w1775, y=w1771) -> (x-y=w1774:dbl)
        n828 = local write "School upkeep"(0.001 ("Hut non-land prod mod")) -> ()
        n829 = local write "Build points"(w1774) -> ()
      }
    }
    n830 = Greater Or Equal?(x=w1056, y=w1050) -> (x >= y?=w1052:bool)
    n831 = Max & Min(x=w989, y=0.0) -> (max(x,y)=w991:dbl)  [unwired: 1 out]
    n832 = Greater Or Equal?(x=w1130, y=1) -> (x >= y?=w1124:bool)
    n833 = Greater Or Equal?(x=w1027, y=1) -> (x >= y?=w995:bool)
    n834 = Greater Or Equal?(x=w1011, y=1) -> (x >= y?=w994:bool)
    n835 = And(x="Taxes level 1", y=w995) -> (x .and. y?=w1025:bool)
    n836 = And(x="Taxes level 3", y=w994) -> (x .and. y?=w1009:bool)
    n837 = Greater Or Equal?(x=w986, y=w991) -> (x >= y?=w990:bool)
    n838 = Not Equal?(x=w1198, y=w1196) -> (x != y?=w1200:bool)
    n839 = Compound Arithmetic op=AND(w1200, "Hut level 1", w1141, w1140) -> (w1199:bool)
    n840 = Greater Or Equal?(x=w950, y=1) -> (x >= y?=w944:bool)
    n841 = Not Equal?(x=w1127, y=w1126) -> (x != y?=w1129:bool)
    n842 = Multiply(x=w1435, y=0.01) -> (x*y=w1434:dbl)
    n843 = Compound Arithmetic op=AND(w1129, "Hut level 3", w1124, w1052) -> (w1128:bool)
    n844 = Not Equal?(x=w1022, y=w1021) -> (x != y?=w1024:bool)
    n845 = And(x=w1024, y=w1025) -> (x .and. y?=w1023:bool)
    n846 = Not Equal?(x=w1006, y=w1005) -> (x != y?=w1008:bool)
    n847 = And(x=w1008, y=w1009) -> (x .and. y?=w1007:bool)
    n848 = Greater Or Equal?(x=w970, y=1) -> (x >= y?=w964:bool)
    n849 = And(x=w964, y=w976) -> (x .and. y?=w963:bool)
    n850 = And(x="Road level 1", y=w963) -> (x .and. y?=w968:bool)
    n851 = Multiply(x=0.99, y=w1435) -> (x*y=w1538:dbl)
    n852 = Not Equal?(x=w945, y=w942) -> (x != y?=w947:bool)
    n853 = And(x=w944, y=w990) -> (x .and. y?=w943:bool)
    n854 = And(x="Road level 3", y=w943) -> (x .and. y?=w948:bool)
    n855 = And(x=w947, y=w948) -> (x .and. y?=w946:bool)
    n856 = case shown="True" w1199 {
      tunnel: w1196 -> [_ w1998]
      tunnel: w1065 -> [_ w1993]
      tunnel: w1064 -> [_ w1994]
      tunnel: w562 -> [_ w1988]
      frame False {
      }
      frame True {
        n857 = local read "Build points"() -> (w1997:dbl)
        n858 = Multiply(x=0.1, y=w1988) -> (x*y=w1989:dbl)
        n859 = local write "Hut level"(w1998) -> ()
        n860 = Add(x=w1993, y=w1994) -> (x+y=w1992:dbl)
        n861 = Increment(x=w1989) -> (x+1=w1991:dbl)
        n862 = local write "Hut upkeep"(0.01 ("Hut dissent add mod")) -> ()
        n863 = Subtract(x=w1997, y=w1993) -> (x-y=w1996:dbl)
        n864 = local write "Hut non-land prod mod"(w1991) -> ()
        n865 = local write "Build points"(w1996) -> ()
        n866 = local write "Hut invested points"(w1992) -> ()
        n867 = local write "Hut dissent mod"(-2.0 ("Hut dissent add mod")) -> ()
      }
    }
    n868 = case shown="True" w1128 {
      tunnel: w1126 -> [_ w1943]
      tunnel: w1051 -> [_ w1938]
      tunnel: w1050 -> [_ w1937]
      tunnel: w562 -> [_ w1933]
      frame False {
      }
      frame True {
        n869 = Multiply(x=w1933, y=0.3) -> (x*y=w1935:dbl)
        n870 = Increment(x=w1935) -> (x+1=w1936:dbl)
        n871 = local read "Build points"() -> (w1942:dbl)
        n872 = Add(x=w1937, y=w1938) -> (x+y=w1939:dbl)
        n873 = local write "Hut non-land prod mod"(w1936) -> ()
        n874 = local write "Hut level"(w1943) -> ()
        n875 = local write "Hut upkeep"(0.15 ("Hut dissent add mod")) -> ()
        n876 = Subtract(x=w1942, y=w1937) -> (x-y=w1941:dbl)
        n877 = local write "Hut invested points"(w1939) -> ()
        n878 = local write "Build points"(w1941) -> ()
        n879 = local write "Hut dissent mod"(-6.0 ("Hut dissent add mod")) -> ()
      }
    }
    n880 = Not Equal?(x=w965, y=w962) -> (x != y?=w967:bool)
    n881 = And(x=w967, y=w968) -> (x .and. y?=w966:bool)
    n882 = Add(x=w1434, y=w1433) -> (x+y=w1432:dbl)
    n883 = Subtract(x=w1313, y=w1432) -> (x-y=w1431:dbl)
    n884 = local write "Temp land change/s"(w1431) -> ()
    n885 = case shown="True" w1023 {
      tunnel: w1021 -> [_ w1882]
      frame False {
      }
      frame True {
        n886 = local write "Taxation\nlevel"(w1882) -> ()
        n887 = local write "Taxes dissent mod"(3.0 ("Taxes dissent add mod")) -> ()
      }
    }
    n888 = case shown="True" w1007 {
      tunnel: w1005 -> [_ w1878]
      frame False {
      }
      frame True {
        n889 = local write "Taxation\nlevel"(w1878) -> ()
        n890 = local write "Taxes dissent mod"(15.0 ("Taxes dissent add mod")) -> ()
      }
    }
    n891 = Greater Or Equal?(x=w707, y=2) -> (x >= y?=w709:bool)
    n892 = Compound Arithmetic op=AND(w682, w636, w709) -> (w683:bool)
    n893 = And(x="School\nlevel 3", y=w683) -> (x .and. y?=w678:bool)
    n894 = And(x=w679, y=w678) -> (x .and. y?=w680:bool)
    n895 = case shown="True" w680 {
      tunnel: w684 -> [_ w1750]
      tunnel: w635 -> [_ w1746]
      tunnel: w634 -> [_ w1745]
      tunnel: w561 -> [_ w1738]
      frame False {
      }
      frame True {
        n896 = Multiply(x=w1738, y=0.15) -> (x*y=w1741:dbl)
        n897 = local read "Build points"() -> (w1749:dbl)
        n898 = Add(x=w1746, y=w1745) -> (x+y=w1747:dbl)
        n899 = Increment(x=w1741) -> (x+1=w1740:dbl)
        n900 = local write "School level"(w1750) -> ()
        n901 = local write "School engineer equivalent"(0.03 ("Hut dissent add mod")) -> ()
        n902 = local write "School invested points"(w1747) -> ()
        n903 = local write "School SP/EP multiplier"(w1740) -> ()
        n904 = local write "School dissent mod"(-3.0 ("Hut non-land prod mod")) -> ()
        n905 = Subtract(x=w1749, y=w1746) -> (x-y=w1748:dbl)
        n906 = local write "School upkeep"(0.01 ("Hut non-land prod mod")) -> ()
        n907 = local write "Build points"(w1748) -> ()
      }
    }
    n908 = case shown="True" w946 {
      tunnel: w942 -> [_ w1856]
      tunnel: w991 -> [_ w1849]
      tunnel: w992 -> [_ w1848]
      frame False {
      }
      frame True {
        n909 = local read "Build points"() -> (w1855:dbl)
        n910 = Add(x=w1849, y=w1848) -> (x+y=w1850:dbl)
        n911 = local write "Road level"(w1856) -> ()
        n912 = local write "Road expansion bonus"(1.0 ("Hut dissent add mod")) -> ()
        n913 = local write "Road land prod mod"(1.3 ("Hut dissent add mod")) -> ()
        n914 = local write "Road invested points"(w1850) -> ()
        n915 = local write "Road upkeep"(0.2 ("Hut non-land prod mod")) -> ()
        n916 = Subtract(x=w1855, y=w1849) -> (x-y=w1854:dbl)
        n917 = local write "Build points"(w1854) -> ()
      }
    }
    n918 = local write "Conquered\nland"(w1538) -> ()
    n919 = case shown="True" w966 {
      tunnel: w962 -> [_ w1874]
      tunnel: w984 -> [_ w1868]
      tunnel: w977 -> [_ w1866]
      frame False {
      }
      frame True {
        n920 = local read "Build points"() -> (w1873:dbl)
        n921 = Add(x=w1866, y=w1868) -> (x+y=w1867:dbl)
        n922 = local write "Road level"(w1874) -> ()
        n923 = local write "Road expansion bonus"(0.2 ("Hut dissent add mod")) -> ()
        n924 = local write "Road land prod mod"(1.1 ("Hut dissent add mod")) -> ()
        n925 = local write "Road invested points"(w1867) -> ()
        n926 = local write "Road upkeep"(0.02 ("Hut non-land prod mod")) -> ()
        n927 = Subtract(x=w1873, y=w1866) -> (x-y=w1872:dbl)
        n928 = local write "Build points"(w1872) -> ()
      }
    }
    n929 = local read "University\ninvested points"() -> (w552:dbl)
    n930 = local read "Economics\nlevel"() -> (w795:i32)
    n931 = local read "Taxation\nlevel"() -> (w800:dbl)
    n932 = local read "Construction\nlevel"() -> (w520:i32)
    n933 = local read "Construction\nlevel"() -> (w497:i32)
    n934 = local read "University level"() -> (w502:i32)
    n935 = local read "Build points"() -> (w548:dbl)
    n936 = local read "University level"() -> (w525:i32)
    n937 = local read "Governance\nlevel"() -> (w494:i32)
    n938 = local read "Build points"() -> (w503:dbl)
    n939 = local read "Military\nScience level"() -> (w1307:i32)
    n940 = Subtract(x=600000 ("y"), y=w552) -> (x-y=w545:dbl)
    n941 = local read "Governance\nlevel"() -> (w488:i32)
    n942 = Greater Or Equal?(x=w795, y=1) -> (x >= y?=w802:bool)
    n943 = And(x="Taxes level 4", y=w802) -> (x .and. y?=w797:bool)
    n944 = Not Equal?(x=w800, y=w801) -> (x != y?=w798:bool)
    n945 = And(x=w798, y=w797) -> (x .and. y?=w799:bool)
    n946 = local read "Biology\nlevel"() -> (w1231:i32)
    n947 = local read "Physics level"() -> (w1273:i32)
    n948 = Max & Min(x=w545, y=0.0) -> (max(x,y)=w550:dbl)  [unwired: 1 out]
    n949 = Greater Or Equal?(x=w548, y=w550) -> (x >= y?=w549:bool)
    n950 = Greater Or Equal?(x=w497, y=2) -> (x >= y?=w506:bool)
    n951 = Greater Or Equal?(x=w503, y=0) -> (x >= y?=w505:bool)
    n952 = case shown="True" w799 {
      tunnel: w801 -> [_ w1802]
      frame False {
      }
      frame True {
        n953 = local write "Taxation\nlevel"(w1802) -> ()
        n954 = local write "Taxes dissent mod"(25.0 ("Taxes dissent add mod")) -> ()
      }
    }
    n955 = Greater Or Equal?(x=w520, y=3) -> (x >= y?=w526:bool)
    n956 = Greater Or Equal?(x=w494, y=2) -> (x >= y?=w493:bool)
    n957 = Not Equal?(x=w502, y=w508) -> (x != y?=w500:bool)
    n958 = Greater Or Equal?(x=w488, y=2) -> (x >= y?=w487:bool)
    n959 = Not Equal?(x=w525, y=w528) -> (x != y?=w523:bool)
    n960 = local read "Governance\nlevel"() -> (w1461:i32)
    n961 = local read "# of level 10 sciences"() -> (w1090:i32)
    n962 = local read "# of level 5 sciences"() -> (w1095:i32)
    n963 = local read "# of level 6 sciences"() -> (w1094:i32)
    n964 = local read "# of level 7 sciences"() -> (w1093:i32)
    n965 = local read "# of level 8 sciences"() -> (w1092:i32)
    n966 = local read "# of level 9 sciences"() -> (w1091:i32)
    n967 = local read "# of level 1 sciences"() -> (w1099:i32)
    n968 = local read "# of level 2 sciences"() -> (w1098:i32)
    n969 = local read "# of level 3 sciences"() -> (w1097:i32)
    n970 = local read "# of level 4 sciences"() -> (w1096:i32)
    n971 = local read "Governance\nlevel"() -> (w1448:i32)
    n972 = Compound Arithmetic op=AND(w506, w505, w493) -> (w507:bool)
    n973 = And(x="University\nlevel 0", y=w507) -> (x .and. y?=w499:bool)
    n974 = And(x=w500, y=w499) -> (x .and. y?=w501:bool)
    n975 = case shown="True" w501 {
      tunnel: w508 -> [_ w1674]
      frame False {
      }
      frame True {
        n976 = local write "University scientist equivalent"(0.0 ("Hut dissent add mod")) -> ()
        n977 = local write "University level"(w1674) -> ()
        n978 = local write "University SP multiplier"(1.0 ("Hut non-land prod mod")) -> ()
        n979 = local write "University dissent mod"(0.0 ("Hut non-land prod mod")) -> ()
        n980 = local write "University upkeep"(0.0 ("Hut non-land prod mod")) -> ()
      }
    }
    n981 = Compound Arithmetic op=AND(w526, w549, w487) -> (w527:bool)
    n982 = And(x="University\nlevel 2", y=w527) -> (x .and. y?=w522:bool)
    n983 = And(x=w523, y=w522) -> (x .and. y?=w524:bool)
    n984 = Greater Or Equal?(x=w1307, y=3.0) -> (x >= y?=w1311:bool)
    n985 = local read "Government"() -> (w1456:string)
    n986 = local read "Government"() -> (w1443:string)
    n987 = And(x="Bow 1", y=w1311) -> (x .and. y?=w1309:bool)
    n988 = local read "Farming level"() -> (w1238:i32)
    n989 = Greater Or Equal?(x=w1231, y=3.0) -> (x >= y?=w1230:bool)
    n990 = Greater Or Equal?(x=w1273, y=3.0) -> (x >= y?=w1274:bool)
    n991 = local read "Governance\nlevel"() -> (w490:i32)
    n992 = local read "Bow level"() -> (w1324:i32)
    n993 = local read "Boat level"() -> (w1266:i32)
    n994 = local read "Governance\nlevel"() -> (w1485:i32)
    n995 = local read "Government"() -> (w1472:string)
    n996 = local read "Spear level"() -> (w1507:i32)
    n997 = local read "SP"() -> (w1455:dbl)
    n998 = local read "SP"() -> (w1442:dbl)
    n999 = local read "Net level"() -> (w1500:i32)
    n1000 = local read "EP"() -> (w1326:dbl)
    n1001 = local read "EP"() -> (w1236:dbl)
    n1002 = local read "EP"() -> (w1268:dbl)
    n1003 = local read "SP"() -> (w1471:dbl)
    n1004 = local read "EP"() -> (w1514:dbl)
    n1005 = local read "Gov elitist\nbuildings mod"() -> (w560:dbl)
    n1006 = case shown="True" w524 {
      tunnel: w528 -> [_ w1700]
      tunnel: w550 -> [_ w1696]
      tunnel: w552 -> [_ w1695]
      tunnel: w560 -> [_ w1688]
      frame False {
      }
      frame True {
        n1007 = Multiply(x=w1688, y=0.3) -> (x*y=w1691:dbl)
        n1008 = Increment(x=w1691) -> (x+1=w1690:dbl)
        n1009 = local read "Build points"() -> (w1699:dbl)
        n1010 = Add(x=w1696, y=w1695) -> (x+y=w1697:dbl)
        n1011 = local write "University scientist equivalent"(0.04 ("Hut dissent add mod")) -> ()
        n1012 = local write "University level"(w1700) -> ()
        n1013 = local write "University dissent mod"(-2.0 ("Hut non-land prod mod")) -> ()
        n1014 = local write "University\ninvested points"(w1697) -> ()
        n1015 = local write "University upkeep"(0.015 ("Hut non-land prod mod")) -> ()
        n1016 = local write "University SP multiplier"(w1690) -> ()
        n1017 = Subtract(x=w1699, y=w1696) -> (x-y=w1698:dbl)
        n1018 = local write "Build points"(w1698) -> ()
      }
    }
    n1019 = local read "University\ninvested points"() -> (w551:dbl)
    n1020 = local read "EP"() -> (w1491:dbl)
    n1021 = Greater Or Equal?(x=w1461, y=1) -> (x >= y?=w1452:bool)
    n1022 = Greater Or Equal?(x=w1455, y=1000) -> (x >= y?=w1453:bool)
    n1023 = Greater Or Equal?(x=w1448, y=1) -> (x >= y?=w1439:bool)
    n1024 = Greater Or Equal?(x=w1442, y=1000) -> (x >= y?=w1440:bool)
    n1025 = Not Equal?(x=w1456, y=w1450) -> (x != y?=w1458:bool)
    n1026 = Greater Or Equal?(x=w1326, y=w1327) -> (x >= y?=w1319:bool)
    n1027 = Greater Or Equal?(x=w1236, y=w1235) -> (x >= y?=w1229:bool)
    n1028 = Greater Or Equal?(x=w1268, y=w1269) -> (x >= y?=w1275:bool)
    n1029 = Greater Or Equal?(x=w1514, y=10000) -> (x >= y?=w1516:bool)
    n1030 = Subtract(x=w1326, y=w1327) -> (x-y=w1328:dbl)
    n1031 = Subtract(x=w1236, y=w1235) -> (x-y=w1234:dbl)
    n1032 = And(x="Net 1", y=w1516) -> (x .and. y?=w1503:bool)
    n1033 = Subtract(x=w1268, y=w1269) -> (x-y=w1270:dbl)
    n1034 = Equal?(x=w1324, y=0.0) -> (x = y?=w1322:bool)
    n1035 = And(x=w1322, y=w1309) -> (x .and. y?=w1323:bool)
    n1036 = And(x=w1323, y=w1319) -> (x .and. y?=w1320:bool)
    n1037 = Equal?(x=w1238, y=0.0) -> (x = y?=w1233:bool)
    n1038 = Not Equal?(x=w1443, y=w1437) -> (x != y?=w1445:bool)
    n1039 = Equal?(x=w1266, y=0.0) -> (x = y?=w1271:bool)
    n1040 = Compound Arithmetic op=AND(w1233, "Farming 1", w1230, w1229) -> (w1228:bool)
    n1041 = Greater Or Equal?(x=w490, y=2) -> (x >= y?=w491:bool)
    n1042 = Compound Arithmetic op=AND(w1271, "Raft", w1274, w1275) -> (w1276:bool)
    n1043 = Increment(x=w1324) -> (x+1=w1325:i32)
    n1044 = Increment(x=w1238) -> (x+1=w1237:i32)
    n1045 = Greater Or Equal?(x=w1485, y=1) -> (x >= y?=w1468:bool)
    n1046 = Increment(x=w1266) -> (x+1=w1267:i32)
    n1047 = Greater Or Equal?(x=w1471, y=1000) -> (x >= y?=w1469:bool)
    n1048 = local read "University\ninvested points"() -> (w559:dbl)
    n1049 = Greater Or Equal?(x=w1491, y=w1490) -> (x >= y?=w1513:bool)
    n1050 = Subtract(x=w1491, y=w1490) -> (x-y=w1489:dbl)
    n1051 = Equal?(x=w1507, y=0.0) -> (x = y?=w1510:bool)
    n1052 = And(x=w1510, y="Sharpened stick") -> (x .and. y?=w1508:bool)
    n1053 = And(x=w1508, y=w1513) -> (x .and. y?=w1512:bool)
    n1054 = Build Array(0, w1099, w1098, w1097, w1096, w1095, w1094, w1093, w1092, w1091, w1090) -> (w1089:T2)
    n1055 = Increment(x=w1507) -> (x+1=w1506:i32)
    n1056 = Equal?(x=w1500, y=0.0) -> (x = y?=w1502:bool)
    n1057 = And(x=w1502, y=w1503) -> (x .and. y?=w1501:bool)
    n1058 = case shown="True" w1276 {
      tunnel: w1267 -> [_ w2094]
      tunnel: w1270 -> [_ w2093]
      frame False {
      }
      frame True {
        n1059 = local read "Trading level no mod"() -> (w2092:i32)
        n1060 = local read "hunting b"() -> (w2089:dbl)
        n1061 = local write "EP"(w2093) -> ()
        n1062 = local write "Boat level"(w2094) -> ()
        n1063 = Increment(x=w2092) -> (x+1=w2091:i32)
        n1064 = local write "Trading level no mod"(w2091) -> ()
        n1065 = Add(x=0.25, y=w2089) -> (x+y=w2090:dbl)
        n1066 = local write "hunting b"(w2090) -> ()
      }
    }
    n1067 = Not Equal?(x=w1472, y=w1466) -> (x != y?=w1482:bool)
    n1068 = And(x=w1452, y=w1453) -> (x .and. y?=w1451:bool)
    n1069 = And(x="Theocracy", y=w1451) -> (x .and. y?=w1459:bool)
    n1070 = And(x=w1458, y=w1459) -> (x .and. y?=w1457:bool)
    n1071 = case shown="True" w1457 {
      tunnel: w1450 -> [_ w2168]
      frame False {
      }
      frame True {
        n1072 = local read "SP"() -> (w2165:dbl)
        n1073 = local write "Government"(w2168) -> ()
        n1074 = Subtract(x=w2165, y=1000) -> (x-y=w2167:dbl)
        n1075 = local write "SP"(w2167) -> ()
      }
    }
    n1076 = And(x=w1439, y=w1440) -> (x .and. y?=w1438:bool)
    n1077 = And(x="Warrior\nSociety", y=w1438) -> (x .and. y?=w1446:bool)
    n1078 = And(x=w1445, y=w1446) -> (x .and. y?=w1444:bool)
    n1079 = case shown="True" w1320 {
      tunnel: w1325 -> [_ w2113]
      tunnel: w1328 -> [_ w2112]
      frame False {
      }
      frame True {
        w2117 = 0.25
        n1080 = local read "Military Modifier"() -> (w2116:dbl)
        n1081 = local write "EP"(w2112) -> ()
        n1082 = local read "hunting b"() -> (w2118:dbl)
        n1083 = local write "Bow level"(w2113) -> ()
        n1084 = Add(x=w2117, y=w2118) -> (x+y=w2114:dbl)
        n1085 = Add(x=w2117, y=w2116) -> (x+y=w2115:dbl)
        n1086 = local write "Military Modifier"(w2115) -> ()
        n1087 = local write "hunting b"(w2114) -> ()
      }
    }
    n1088 = case shown="True" w1228 {
      tunnel: w1237 -> [_ w2073]
      tunnel: w1234 -> [_ w2072]
      frame False {
      }
      frame True {
        n1089 = local read "hunting b"() -> (w2070:dbl)
        n1090 = local read "hunting a"() -> (w2067:dbl)
        n1091 = local write "EP"(w2072) -> ()
        n1092 = local write "Farming level"(w2073) -> ()
        n1093 = Add(x=1.5, y=w2067) -> (x+y=w2066:dbl)
        n1094 = Add(x=1.5, y=w2070) -> (x+y=w2071:dbl)
        n1095 = local write "hunting b"(w2071) -> ()
        n1096 = local write "hunting a"(w2066) -> ()
      }
    }
    n1097 = case shown="True" w1444 {
      tunnel: w1437 -> [_ w2164]
      frame False {
      }
      frame True {
        n1098 = local read "SP"() -> (w2163:dbl)
        n1099 = local write "Government"(w2164) -> ()
        n1100 = Subtract(x=w2163, y=1000) -> (x-y=w2161:dbl)
        n1101 = local write "SP"(w2161) -> ()
      }
    }
    n1102 = Increment(x=w1500) -> (x+1=w1499:i32)
    n1103 = case shown="True" w1512 {
      tunnel: w1506 -> [_ w2677]
      tunnel: w1489 -> [_ w2676]
      frame False {
      }
      frame True {
        w2681 = 0.25
        n1104 = local write "EP"(w2676) -> ()
        n1105 = local read "warrior a"() -> (w2680:dbl)
        n1106 = local read "hunting a"() -> (w2682:dbl)
        n1107 = local write "Spear level"(w2677) -> ()
        n1108 = Add(x=w2681, y=w2680) -> (x+y=w2679:dbl)
        n1109 = Add(x=w2681, y=w2682) -> (x+y=w2678:dbl)
        n1110 = local write "warrior a"(w2679) -> ()
        n1111 = local write "hunting a"(w2678) -> ()
      }
    }
    n1112 = case shown="True" w1501 {
      tunnel: w1514 -> [_ w2671]
      tunnel: w1499 -> [_ w2669]
      frame False {
      }
      frame True {
        n1113 = local read "hunting b"() -> (w2674:dbl)
        n1114 = local write "Net level"(w2669) -> ()
        n1115 = Subtract(x=w2671, y=10000.0) -> (x-y=w2670:dbl)
        n1116 = local write "EP"(w2670) -> ()
        n1117 = Add(x=w2674, y=0.25) -> (x+y=w2673:dbl)
        n1118 = local write "hunting b"(w2673) -> ()
      }
    }
    n1119 = And(x=w1468, y=w1469) -> (x .and. y?=w1467:bool)
    n1120 = And(x="Democracy", y=w1467) -> (x .and. y?=w1483:bool)
    n1121 = And(x=w1482, y=w1483) -> (x .and. y?=w1481:bool)
    n1122 = call-poly <vilib>:"Matrix To Array.vi"("Real Matrix"=w1089) -> ("Real 2D Array"=w1088:dbl[][])
    n1123 = case shown="True" w1481 {
      tunnel: w1466 -> [_ w2182]
      frame False {
      }
      frame True {
        n1124 = local write "Government"(w2182) -> ()
        n1125 = local read "SP"() -> (w2181:dbl)
        n1126 = Subtract(x=w2181, y=1000) -> (x-y=w2179:dbl)
        n1127 = local write "SP"(w2179) -> ()
      }
    }
    n1128 = local read "Construction\nlevel"() -> (w537:i32)
    n1129 = local read "Build points"() -> (w542:dbl)
    n1130 = Index Array(array=w1088, index (row)=0) -> (element=w144:dbl[])  [unwired: 1 in]
    n1131 = local read "Military\nScience level"() -> (w1488:i32)
    n1132 = Subtract(x=200000 ("y"), y=w551) -> (x-y=w539:dbl)
    n1133 = local read "Construction\nlevel"() -> (w517:i32)
    n1134 = local read "University level"() -> (w512:i32)
    n1135 = local read "University level"() -> (w532:i32)
    n1136 = local read "Build points"() -> (w553:dbl)
    n1137 = local read "Governance\nlevel"() -> (w1473:i32)
    n1138 = Subtract(x=2000000 ("y"), y=w559) -> (x-y=w556:dbl)
    n1139 = Max & Min(x=w539, y=0.0) -> (max(x,y)=w544:dbl)  [unwired: 1 out]
    n1140 = Greater Or Equal?(x=w542, y=w544) -> (x >= y?=w543:bool)
    n1141 = local read "Military\nScience level"() -> (w1360:i32)
    n1142 = Max & Min(x=w556, y=0.0) -> (max(x,y)=w558:dbl)  [unwired: 1 out]
    n1143 = Greater Or Equal?(x=w553, y=w558) -> (x >= y?=w557:bool)
    n1144 = Greater Or Equal?(x=w517, y=3) -> (x >= y?=w511:bool)
    n1145 = Greater Or Equal?(x=w537, y=2) -> (x >= y?=w531:bool)
    n1146 = Compound Arithmetic op=AND(w531, w543, w491) -> (w530:bool)
    n1147 = And(x="University\nlevel 1", y=w530) -> (x .and. y?=w535:bool)
    n1148 = local read "Governance\nlevel"() -> (w1406:i32)
    n1149 = local read "Governance\nlevel"() -> (w1404:i32)
    n1150 = Not Equal?(x=w512, y=w509) -> (x != y?=w514:bool)
    n1151 = Not Equal?(x=w532, y=w529) -> (x != y?=w534:bool)
    n1152 = And(x=w534, y=w535) -> (x .and. y?=w533:bool)
    n1153 = local read "SP"() -> (w1493:dbl)
    n1154 = Increment(x=w1488) -> (x+1=w1086:i32)
    n1155 = Index Array(array=w144, index=w1086) -> (element=w1084:dbl)
    n1156 = Power Of 10(x=w1488) -> (10^x=w1497:dbl)
    n1157 = local read "SP"() -> (w1475:dbl)
    n1158 = local read "Governance\nlevel"() -> (w1419:i32)
    n1159 = Power Of 10(x=w1473) -> (10^x=w1479:dbl)
    n1160 = Power Of 2(x=w1084) -> (2^x=w1085:dbl)
    n1161 = local read "Government"() -> (w1424:string)
    n1162 = local read "Governance\nlevel"() -> (w486:i32)
    n1163 = local read "Government"() -> (w1411:string)
    n1164 = local read "Government"() -> (w1399:string)
    n1165 = local read "Net level"() -> (w1379:i32)
    n1166 = case shown="True" w533 {
      tunnel: w529 -> [_ w1713]
      tunnel: w551 -> [_ w1710]
      tunnel: w544 -> [_ w1708]
      tunnel: w560 -> [_ w1701]
      frame False {
      }
      frame True {
        n1167 = Multiply(x=w1701, y=0.15) -> (x*y=w1703:dbl)
        n1168 = Increment(x=w1703) -> (x+1=w1704:dbl)
        n1169 = local read "Build points"() -> (w1712:dbl)
        n1170 = Add(x=w1708, y=w1710) -> (x+y=w1709:dbl)
        n1171 = local write "University level"(w1713) -> ()
        n1172 = local write "University scientist equivalent"(0.02 ("Hut dissent add mod")) -> ()
        n1173 = local write "University\ninvested points"(w1709) -> ()
        n1174 = local write "University SP multiplier"(w1704) -> ()
        n1175 = local write "University dissent mod"(-1.0 ("Hut non-land prod mod")) -> ()
        n1176 = local write "University upkeep"(0.005 ("Hut non-land prod mod")) -> ()
        n1177 = Subtract(x=w1712, y=w1708) -> (x-y=w1711:dbl)
        n1178 = local write "Build points"(w1711) -> ()
      }
    }
    n1179 = Compound Arithmetic op=MULTIPLY(w1497, 1000, w1085) -> (w1492:dbl)
    n1180 = local read "Military\nScience level"() -> (w1116:i32)
    n1181 = local read "Military\nScience level"() -> (w1306:i32)
    n1182 = local read "EP"() -> (w1373:dbl)
    n1183 = Greater?(x=w1493, y=w1492) -> (0:w1495:bool)
    n1184 = And(x="Military science", y=w1495) -> (x .and. y?=w1494:bool)
    n1185 = local read "SP"() -> (w1425:dbl)
    n1186 = local read "SP"() -> (w1412:dbl)
    n1187 = local read "SP"() -> (w1398:dbl)
    n1188 = local read "Physics level"() -> (w1281:i32)
    n1189 = local read "Physics level"() -> (w1254:i32)
    n1190 = local read "Biology\nlevel"() -> (w1212:i32)
    n1191 = Greater Or Equal?(x=w1373, y=100000) -> (x >= y?=w1371:bool)
    n1192 = And(x="Net 2", y=w1371) -> (x .and. y?=w1376:bool)
    n1193 = Greater Or Equal?(x=w1360, y=1.0) -> (x >= y?=w1359:bool)
    n1194 = case shown="True" w1494 {
      selector: w1494 -> [w2659 w2662]
      tunnel: w1493 -> [_ w2665]
      tunnel: w1492 -> [_ w2664]
      tunnel: w1086 -> [_ w2661]
      tunnel: [w2659 w2662] -> w1101
      tunnel: [0 w2661] -> w1112
      frame False {
      }
      frame True {
        n1195 = local read "warrior c"() -> (w2668:dbl)
        n1196 = Subtract(x=w2665, y=w2664) -> (x-y=w2663:dbl)
        n1197 = local write "SP"(w2663) -> ()
        n1198 = Subtract(x=w2668, y=0.05) -> (x-y=w2667:dbl)
        n1199 = local write "Military\nScience level"(w2661) -> ()
        n1200 = local write "warrior c"(w2667) -> ()
      }
    }
    n1201 = Increment(x=w1473) -> (x+1=w1081:i32)
    n1202 = Index Array(array=w144, index=w1081) -> (element=w1083:dbl)
    n1203 = Power Of 2(x=w1083) -> (2^x=w1082:dbl)
    n1204 = Compound Arithmetic op=MULTIPLY(w1479, 1000, w1082) -> (w1474:dbl)
    n1205 = Greater?(x=w1475, y=w1474) -> (0:w1477:bool)
    n1206 = And(x="Governance", y=w1477) -> (x .and. y?=w1476:bool)
    n1207 = case shown="True" w1476 {
      selector: w1476 -> [w2169 w2172]
      tunnel: w1475 -> [_ w2178]
      tunnel: w1474 -> [_ w2177]
      tunnel: w1081 -> [_ w2171]
      tunnel: [w2169 w2172] -> w1102
      tunnel: [0 w2171] -> w1111
      frame False {
      }
      frame True {
        n1208 = local read "Dissent multiplier"() -> (w2175:dbl)
        n1209 = Subtract(x=w2178, y=w2177) -> (x-y=w2176:dbl)
        n1210 = local write "SP"(w2176) -> ()
        n1211 = Subtract(x=w2175, y=0.05) -> (x-y=w2173:dbl)
        n1212 = local write "Governance\nlevel"(w2171) -> ()
        n1213 = local write "Dissent multiplier"(w2173) -> ()
      }
    }
    n1214 = Greater Or Equal?(x=w1419, y=2) -> (x >= y?=w1428:bool)
    n1215 = Greater Or Equal?(x=w1425, y=100000) -> (x >= y?=w1427:bool)
    n1216 = Greater Or Equal?(x=w1406, y=2) -> (x >= y?=w1415:bool)
    n1217 = Equal?(x=w1379, y=1.0) -> (x = y?=w1377:bool)
    n1218 = And(x=w1377, y=w1376) -> (x .and. y?=w1378:bool)
    n1219 = Greater Or Equal?(x=w1412, y=100000) -> (x >= y?=w1414:bool)
    n1220 = Greater Or Equal?(x=w1404, y=2) -> (x >= y?=w1395:bool)
    n1221 = Greater Or Equal?(x=w1398, y=100000) -> (x >= y?=w1396:bool)
    n1222 = And(x="Stone\nspear", y=w1359) -> (x .and. y?=w1357:bool)
    n1223 = Greater Or Equal?(x=w486, y=2) -> (x >= y?=w484:bool)
    n1224 = Compound Arithmetic op=AND(w511, w557, w484) -> (w510:bool)
    n1225 = And(x="University\nlevel 3", y=w510) -> (x .and. y?=w515:bool)
    n1226 = And(x=w514, y=w515) -> (x .and. y?=w513:bool)
    n1227 = case shown="True" w513 {
      tunnel: w509 -> [_ w1687]
      tunnel: w558 -> [_ w1683]
      tunnel: w559 -> [_ w1682]
      tunnel: w560 -> [_ w1675]
      frame False {
      }
      frame True {
        n1228 = Multiply(x=w1675, y=0.45) -> (x*y=w1678:dbl)
        n1229 = local read "Build points"() -> (w1686:dbl)
        n1230 = Add(x=w1683, y=w1682) -> (x+y=w1684:dbl)
        n1231 = Increment(x=w1678) -> (x+1=w1677:dbl)
        n1232 = local write "University level"(w1687) -> ()
        n1233 = local write "University scientist equivalent"(0.06 ("Hut dissent add mod")) -> ()
        n1234 = local write "University\ninvested points"(w1684) -> ()
        n1235 = local write "University dissent mod"(-3.0 ("Hut non-land prod mod")) -> ()
        n1236 = local write "University SP multiplier"(w1677) -> ()
        n1237 = local write "University upkeep"(0.05 ("Hut non-land prod mod")) -> ()
        n1238 = Subtract(x=w1686, y=w1683) -> (x-y=w1685:dbl)
        n1239 = local write "Build points"(w1685) -> ()
      }
    }
    n1240 = Not Equal?(x=w1424, y=w1430) -> (x != y?=w1422:bool)
    n1241 = local read "Spear level"() -> (w1363:i32)
    n1242 = Not Equal?(x=w1411, y=w1417) -> (x != y?=w1409:bool)
    n1243 = Not Equal?(x=w1399, y=w1393) -> (x != y?=w1401:bool)
    n1244 = Increment(x=w1379) -> (x+1=w1380:i32)
    n1245 = case shown="True" w1378 {
      tunnel: w1373 -> [_ w2144]
      tunnel: w1380 -> [_ w2142]
      frame False {
      }
      frame True {
        n1246 = local read "hunting b"() -> (w2147:dbl)
        n1247 = local write "Net level"(w2142) -> ()
        n1248 = Subtract(x=w2144, y=10000.0) -> (x-y=w2143:dbl)
        n1249 = local write "EP"(w2143) -> ()
        n1250 = Add(x=w2147, y=0.25) -> (x+y=w2146:dbl)
        n1251 = local write "hunting b"(w2146) -> ()
      }
    }
    n1252 = And(x=w1428, y=w1427) -> (x .and. y?=w1429:bool)
    n1253 = And(x="Democracy 2", y=w1429) -> (x .and. y?=w1421:bool)
    n1254 = And(x=w1422, y=w1421) -> (x .and. y?=w1423:bool)
    n1255 = local read "EP"() -> (w1368:dbl)
    n1256 = case shown="True" w1423 {
      tunnel: w1430 -> [_ w2160]
      frame False {
      }
      frame True {
        n1257 = local write "Government"(w2160) -> ()
        n1258 = local read "SP"() -> (w2157:dbl)
        n1259 = Subtract(x=w2157, y=100000) -> (x-y=w2159:dbl)
        n1260 = local write "SP"(w2159) -> ()
      }
    }
    n1261 = And(x=w1415, y=w1414) -> (x .and. y?=w1416:bool)
    n1262 = And(x="Theocracy 2", y=w1416) -> (x .and. y?=w1408:bool)
    n1263 = And(x=w1409, y=w1408) -> (x .and. y?=w1410:bool)
    n1264 = And(x=w1395, y=w1396) -> (x .and. y?=w1394:bool)
    n1265 = And(x="Warrior\nSociety 2", y=w1394) -> (x .and. y?=w1402:bool)
    n1266 = And(x=w1401, y=w1402) -> (x .and. y?=w1400:bool)
    n1267 = case shown="True" w1410 {
      tunnel: w1417 -> [_ w2156]
      frame False {
      }
      frame True {
        n1268 = local write "Government"(w2156) -> ()
        n1269 = local read "SP"() -> (w2155:dbl)
        n1270 = Subtract(x=w2155, y=100000) -> (x-y=w2153:dbl)
        n1271 = local write "SP"(w2153) -> ()
      }
    }
    n1272 = case shown="True" w1400 {
      tunnel: w1393 -> [_ w2152]
      frame False {
      }
      frame True {
        n1273 = local write "Government"(w2152) -> ()
        n1274 = local read "SP"() -> (w2149:dbl)
        n1275 = Subtract(x=w2149, y=100000) -> (x-y=w2151:dbl)
        n1276 = local write "SP"(w2151) -> ()
      }
    }
    n1277 = Greater Or Equal?(x=w1368, y=10000) -> (x >= y?=w1370:bool)
    n1278 = And(x=w1357, y=w1370) -> (x .and. y?=w1366:bool)
    n1279 = Equal?(x=w1363, y=1.0) -> (x = y?=w1365:bool)
    n1280 = And(x=w1365, y=w1366) -> (x .and. y?=w1364:bool)
    n1281 = Greater Or Equal?(x=w1281, y=3.0) -> (x >= y?=w1279:bool)
    n1282 = local read "Bow level"() -> (w1304:i32)
    n1283 = local read "Farming level"() -> (w1205:i32)
    n1284 = Greater Or Equal?(x=w1254, y=4.0) -> (x >= y?=w1253:bool)
    n1285 = local read "Boat level"() -> (w1261:i32)
    n1286 = Greater Or Equal?(x=w1116, y=3.0) -> (x >= y?=w1114:bool)
    n1287 = Greater Or Equal?(x=w1212, y=4.0) -> (x >= y?=w1213:bool)
    n1288 = Greater Or Equal?(x=w1306, y=3.0) -> (x >= y?=w1280:bool)
    n1289 = Increment(x=w1363) -> (x+1=w1362:i32)
    n1290 = local read "EP"() -> (w1302:dbl)
    n1291 = local read "EP"() -> (w1259:dbl)
    n1292 = case shown="True" w1364 {
      tunnel: w1368 -> [_ w2140]
      tunnel: w1362 -> [_ w2138]
      frame False {
      }
      frame True {
        w2134 = 0.25
        n1293 = local read "warrior a"() -> (w2135:dbl)
        n1294 = local read "hunting a"() -> (w2133:dbl)
        n1295 = local write "Spear level"(w2138) -> ()
        n1296 = Subtract(x=w2140, y=10000.0) -> (x-y=w2139:dbl)
        n1297 = local write "EP"(w2139) -> ()
        n1298 = Add(x=w2134, y=w2135) -> (x+y=w2136:dbl)
        n1299 = Add(x=w2134, y=w2133) -> (x+y=w2137:dbl)
        n1300 = local write "warrior a"(w2136) -> ()
        n1301 = local write "hunting a"(w2137) -> ()
      }
    }
    n1302 = local read "EP"() -> (w1207:dbl)
    n1303 = Greater Or Equal?(x=w1302, y=w1301) -> (x >= y?=w1278:bool)
    n1304 = Subtract(x=w1302, y=w1301) -> (x-y=w1300:dbl)
    n1305 = Equal?(x=w1304, y=1.0) -> (x = y?=w1285:bool)
    n1306 = Greater Or Equal?(x=w1259, y=w1258) -> (x >= y?=w1252:bool)
    n1307 = Compound Arithmetic op=AND(w1285, "Bow 2", w1280, w1279, w1278) -> (w1277:bool)
    n1308 = Increment(x=w1304) -> (x+1=w1303:i32)
    n1309 = Subtract(x=w1259, y=w1258) -> (x-y=w1257:dbl)
    n1310 = Equal?(x=w1261, y=1.0) -> (x = y?=w1256:bool)
    n1311 = Compound Arithmetic op=AND(w1256, "Trireme", w1253, w1114, w1252) -> (w1251:bool)
    n1312 = Greater Or Equal?(x=w1207, y=w1208) -> (x >= y?=w1214:bool)
    n1313 = Increment(x=w1261) -> (x+1=w1260:i32)
    n1314 = Subtract(x=w1207, y=w1208) -> (x-y=w1209:dbl)
    n1315 = Equal?(x=w1205, y=1.0) -> (x = y?=w1210:bool)
    n1316 = Compound Arithmetic op=AND(w1210, "Farming 2", w1213, w1214) -> (w1215:bool)
    n1317 = Increment(x=w1205) -> (x+1=w1206:i32)
    n1318 = case shown="True" w1251 {
      tunnel: w1260 -> [_ w2087]
      tunnel: w1257 -> [_ w2086]
      frame False {
      }
      frame True {
        n1319 = local read "Trading level no mod"() -> (w2085:i32)
        n1320 = local read "warrior b"() -> (w2082:dbl)
        n1321 = local write "EP"(w2086) -> ()
        n1322 = local write "Boat level"(w2087) -> ()
        n1323 = Increment(x=w2085) -> (x+1=w2084:i32)
        n1324 = local write "Trading level no mod"(w2084) -> ()
        n1325 = Add(x=0.5, y=w2082) -> (x+y=w2083:dbl)
        n1326 = local write "warrior b"(w2083) -> ()
      }
    }
    n1327 = local read "Military\nScience level"() -> (w563:i32)
    n1328 = case shown="True" w1277 {
      tunnel: w1303 -> [_ w2111]
      tunnel: w1300 -> [_ w2110]
      frame False {
      }
      frame True {
        w2105 = 0.5 ("x")
        n1329 = local read "hunting a"() -> (w2109:dbl)
        n1330 = local read "warrior a"() -> (w2106:dbl)
        n1331 = local write "EP"(w2110) -> ()
        n1332 = local write "Bow level"(w2111) -> ()
        n1333 = Add(x=w2105, y=w2109) -> (x+y=w2108:dbl)
        n1334 = Add(x=w2105, y=w2106) -> (x+y=w2107:dbl)
        n1335 = local write "hunting a"(w2108) -> ()
        n1336 = local write "warrior a"(w2107) -> ()
      }
    }
    n1337 = case shown="True" w1215 {
      tunnel: w1206 -> [_ w2060]
      tunnel: w1209 -> [_ w2059]
      frame False {
      }
      frame True {
        n1338 = local read "hunting b"() -> (w2057:dbl)
        n1339 = local read "hunting a"() -> (w2054:dbl)
        n1340 = local write "EP"(w2059) -> ()
        n1341 = local write "Farming level"(w2060) -> ()
        n1342 = Add(x=1.5, y=w2054) -> (x+y=w2053:dbl)
        n1343 = Add(x=1.5, y=w2057) -> (x+y=w2058:dbl)
        n1344 = local write "hunting b"(w2058) -> ()
        n1345 = local write "hunting a"(w2053) -> ()
      }
    }
    n1346 = local read "Physics level"() -> (w574:i32)
    n1347 = local read "Governance\nlevel"() -> (w773:i32)
    n1348 = local read "Governance\nlevel"() -> (w775:i32)
    n1349 = local read "Physics level"() -> (w1292:i32)
    n1350 = local read "Governance\nlevel"() -> (w760:i32)
    n1351 = local read "Construction\nlevel"() -> (w1299:i32)
    n1352 = local read "Government"() -> (w755:string)
    n1353 = local read "Government"() -> (w768:string)
    n1354 = local read "Government"() -> (w780:string)
    n1355 = local read "SP"() -> (w754:dbl)
    n1356 = local read "SP"() -> (w767:dbl)
    n1357 = local read "SP"() -> (w781:dbl)
    n1358 = local read "Military\nScience level"() -> (w1339:i32)
    n1359 = Greater Or Equal?(x=w574, y=4.0) -> (x >= y?=w576:bool)
    n1360 = local read "Bow level"() -> (w565:i32)
    n1361 = Greater Or Equal?(x=w760, y=4) -> (x >= y?=w751:bool)
    n1362 = Greater Or Equal?(x=w1339, y=2.0) -> (x >= y?=w1340:bool)
    n1363 = Greater Or Equal?(x=w754, y=5000000) -> (x >= y?=w752:bool)
    n1364 = Greater Or Equal?(x=w773, y=4) -> (x >= y?=w764:bool)
    n1365 = Greater Or Equal?(x=w767, y=5000000) -> (x >= y?=w765:bool)
    n1366 = Greater Or Equal?(x=w775, y=4) -> (x >= y?=w784:bool)
    n1367 = Greater Or Equal?(x=w781, y=5000000) -> (x >= y?=w783:bool)
    n1368 = Greater Or Equal?(x=w563, y=5.0) -> (x >= y?=w575:bool)
    n1369 = Not Equal?(x=w755, y=w749) -> (x != y?=w757:bool)
    n1370 = And(x="Bronze\nSpear", y=w1340) -> (x .and. y?=w1336:bool)
    n1371 = Not Equal?(x=w768, y=w762) -> (x != y?=w770:bool)
    n1372 = Not Equal?(x=w780, y=w786) -> (x != y?=w778:bool)
    n1373 = local read "SP"() -> (w1290:dbl)
    n1374 = local read "EP"() -> (w567:dbl)
    n1375 = local read "Spear level"() -> (w1350:i32)
    n1376 = Power Of 10(x=w1292) -> (10^x=w1287:dbl)
    n1377 = local read "SP"() -> (w1297:dbl)
    n1378 = And(x=w751, y=w752) -> (x .and. y?=w750:bool)
    n1379 = And(x="Confederacy", y=w750) -> (x .and. y?=w758:bool)
    n1380 = And(x=w757, y=w758) -> (x .and. y?=w756:bool)
    n1381 = Power Of 10(x=w1299) -> (10^x=w1294:dbl)
    n1382 = case shown="True" w756 {
      tunnel: w749 -> [_ w1800]
      frame False {
      }
      frame True {
        n1383 = local write "Government"(w1800) -> ()
        n1384 = local read "SP"() -> (w1797:dbl)
        n1385 = Subtract(x=w1797, y=5000000) -> (x-y=w1799:dbl)
        n1386 = local write "SP"(w1799) -> ()
      }
    }
    n1387 = And(x=w764, y=w765) -> (x .and. y?=w763:bool)
    n1388 = And(x="Republic", y=w763) -> (x .and. y?=w771:bool)
    n1389 = And(x=w770, y=w771) -> (x .and. y?=w769:bool)
    n1390 = And(x=w784, y=w783) -> (x .and. y?=w785:bool)
    n1391 = And(x="Kingdom", y=w785) -> (x .and. y?=w777:bool)
    n1392 = And(x=w778, y=w777) -> (x .and. y?=w779:bool)
    n1393 = case shown="True" w769 {
      tunnel: w762 -> [_ w1796]
      frame False {
      }
      frame True {
        n1394 = local write "Government"(w1796) -> ()
        n1395 = local read "SP"() -> (w1795:dbl)
        n1396 = Subtract(x=w1795, y=5000000) -> (x-y=w1793:dbl)
        n1397 = local write "SP"(w1793) -> ()
      }
    }
    n1398 = case shown="True" w779 {
      tunnel: w786 -> [_ w1792]
      frame False {
      }
      frame True {
        n1399 = local write "Government"(w1792) -> ()
        n1400 = local read "SP"() -> (w1789:dbl)
        n1401 = Subtract(x=w1789, y=5000000) -> (x-y=w1791:dbl)
        n1402 = local write "SP"(w1791) -> ()
      }
    }
    n1403 = local read "EP"() -> (w1355:dbl)
    n1404 = Greater Or Equal?(x=w567, y=w568) -> (x >= y?=w577:bool)
    n1405 = Subtract(x=w567, y=w568) -> (x-y=w569:dbl)
    n1406 = Equal?(x=w565, y=2.0) -> (x = y?=w570:bool)
    n1407 = Compound Arithmetic op=AND(w570, "Longbow", w575, w576, w577) -> (w578:bool)
    n1408 = Increment(x=w565) -> (x+1=w566:i32)
    n1409 = Greater Or Equal?(x=w1355, y=w1329) -> (x >= y?=w1356:bool)
    n1410 = And(x=w1336, y=w1356) -> (x .and. y?=w1353:bool)
    n1411 = Increment(x=w1292) -> (x+1=w1080:i32)
    n1412 = Index Array(array=w144, index=w1080) -> (element=w1079:dbl)
    n1413 = Power Of 2(x=w1079) -> (2^x=w1078:dbl)
    n1414 = Compound Arithmetic op=MULTIPLY(w1287, 1000, w1078) -> (w1291:dbl)
    n1415 = Greater?(x=w1290, y=w1291) -> (0:w1289:bool)
    n1416 = And(x="Physics", y=w1289) -> (x .and. y?=w1103:bool)
    n1417 = Equal?(x=w1350, y=2.0) -> (x = y?=w1352:bool)
    n1418 = And(x=w1352, y=w1353) -> (x .and. y?=w1351:bool)
    n1419 = local read "Physics level"() -> (w160:i32)
    n1420 = local read "Physics level"() -> (w187:i32)
    n1421 = local read "Military\nScience level"() -> (w162:i32)
    n1422 = case shown="True" w578 {
      tunnel: w566 -> [_ w1718]
      tunnel: w569 -> [_ w1717]
      frame False {
      }
      frame True {
        n1423 = local write "EP"(w1717) -> ()
        n1424 = local read "warrior a"() -> (w1715:dbl)
        n1425 = local write "Bow level"(w1718) -> ()
        n1426 = Add(x=0.5, y=w1715) -> (x+y=w1716:dbl)
        n1427 = local write "warrior a"(w1716) -> ()
      }
    }
    n1428 = local read "Military\nScience level"() -> (w185:i32)
    n1429 = local read "Physics level"() -> (w192:i32)
    n1430 = local read "Military\nScience level"() -> (w194:i32)
    n1431 = local read "Physics level"() -> (w251:i32)
    n1432 = local read "Military\nScience level"() -> (w208:i32)
    n1433 = local read "Physics level"() -> (w249:i32)
    n1434 = local read "Military\nScience level"() -> (w243:i32)
    n1435 = case shown="True" w1103 {
      tunnel: w1290 -> [_ w2104]
      tunnel: w1291 -> [_ w2103]
      tunnel: w1080 -> [_ w2101]
      tunnel: [0 w2101] -> w1110
      frame False {
      }
      frame True {
        n1436 = Subtract(x=w2104, y=w2103) -> (x-y=w2102:dbl)
        n1437 = local write "SP"(w2102) -> ()
        n1438 = local write "Physics level"(w2101) -> ()
      }
    }
    n1439 = local read "Physics level"() -> (w245:i32)
    n1440 = Increment(x=w1350) -> (x+1=w1349:i32)
    n1441 = local read "Military\nScience level"() -> (w211:i32)
    n1442 = Increment(x=w1299) -> (x+1=w1077:i32)
    n1443 = Index Array(array=w144, index=w1077) -> (element=w1076:dbl)
    n1444 = Power Of 2(x=w1076) -> (2^x=w1075:dbl)
    n1445 = Compound Arithmetic op=MULTIPLY(w1294, 1000, w1075) -> (w1298:dbl)
    n1446 = Greater?(x=w1297, y=w1298) -> (0:w1296:bool)
    n1447 = And(x="Construction", y=w1296) -> (x .and. y?=w1104:bool)
    n1448 = case shown="True" w1104 {
      tunnel: w1297 -> [_ w2099]
      tunnel: w1298 -> [_ w2098]
      tunnel: w1077 -> [_ w2096]
      tunnel: [0 w2096] -> w1109
      frame False {
      }
      frame True {
        n1449 = Subtract(x=w2099, y=w2098) -> (x-y=w2097:dbl)
        n1450 = local write "SP"(w2097) -> ()
        n1451 = local write "Construction\nlevel"(w2096) -> ()
      }
    }
    n1452 = case shown="True" w1351 {
      tunnel: w1355 -> [_ w2129]
      tunnel: w1349 -> [_ w2127]
      tunnel: w1329 -> [_ w2126]
      frame False {
      }
      frame True {
        n1453 = local read "warrior a"() -> (w2131:dbl)
        n1454 = local write "Spear level"(w2127) -> ()
        n1455 = Subtract(x=w2129, y=w2126) -> (x-y=w2128:dbl)
        n1456 = local write "EP"(w2128) -> ()
        n1457 = Add(x=w2131, y=0.5) -> (x+y=w2130:dbl)
        n1458 = local write "warrior a"(w2130) -> ()
      }
    }
    n1459 = local read "Economics\nlevel"() -> (w335:i32)
    n1460 = local read "Economics\nlevel"() -> (w336:i32)
    n1461 = local read "Economics\nlevel"() -> (w332:i32)
    n1462 = local read "Biology\nlevel"() -> (w607:i32)
    n1463 = local read "Biology\nlevel"() -> (w608:i32)
    n1464 = local read "Construction\nlevel"() -> (w579:i32)
    n1465 = local read "Construction\nlevel"() -> (w823:i32)
    n1466 = local read "Biology\nlevel"() -> (w633:i32)
    n1467 = local read "Construction\nlevel"() -> (w824:i32)
    n1468 = local read "Military\nScience level"() -> (w1334:i32)
    n1469 = local read "Physics level"() -> (w590:i32)
    n1470 = local read "Physics level"() -> (w812:i32)
    n1471 = local read "Physics level"() -> (w835:i32)
    n1472 = local read "Siege weapon\nlevel"() -> (w165:i32)
    n1473 = local read "Siege weapon\nlevel"() -> (w182:i32)
    n1474 = local read "Siege weapon\nlevel"() -> (w197:i32)
    n1475 = local read "Siege weapon\nlevel"() -> (w223:i32)
    n1476 = local read "Siege weapon\nlevel"() -> (w240:i32)
    n1477 = local read "Siege weapon\nlevel"() -> (w220:i32)
    n1478 = local read "Tax method\nlevel"() -> (w303:i32)
    n1479 = local read "Tax method\nlevel"() -> (w320:i32)
    n1480 = local read "Construction\ntools level"() -> (w581:i32)
    n1481 = local read "Construction\ntools level"() -> (w821:i32)
    n1482 = local read "Medicine level"() -> (w605:i32)
    n1483 = Greater Or Equal?(x=w160, y=9.0) -> (x >= y?=w158:bool)
    n1484 = local read "Medicine level"() -> (w610:i32)
    n1485 = Greater Or Equal?(x=w187, y=8.0) -> (x >= y?=w189:bool)
    n1486 = local read "Tax method\nlevel"() -> (w323:i32)
    n1487 = local read "Governance\nlevel"() -> (w724:i32)
    n1488 = Greater Or Equal?(x=w192, y=7.0) -> (x >= y?=w190:bool)
    n1489 = local read "Governance\nlevel"() -> (w722:i32)
    n1490 = local read "Construction\ntools level"() -> (w826:i32)
    n1491 = Greater Or Equal?(x=w251, y=6.0) -> (x >= y?=w253:bool)
    n1492 = Greater Or Equal?(x=w249, y=5.0) -> (x >= y?=w250:bool)
    n1493 = local read "Medicine level"() -> (w631:i32)
    n1494 = Greater Or Equal?(x=w245, y=4.0) -> (x >= y?=w247:bool)
    n1495 = Greater Or Equal?(x=w162, y=8.0) -> (x >= y?=w161:bool)
    n1496 = Greater Or Equal?(x=w185, y=7.0) -> (x >= y?=w186:bool)
    n1497 = Greater Or Equal?(x=w194, y=6.0) -> (x >= y?=w193:bool)
    n1498 = Greater Or Equal?(x=w208, y=3.0) -> (x >= y?=w207:bool)
    n1499 = Greater Or Equal?(x=w243, y=4.0) -> (x >= y?=w244:bool)
    n1500 = local read "Governance\nlevel"() -> (w737:i32)
    n1501 = Greater Or Equal?(x=w211, y=3.0) -> (x >= y?=w206:bool)
    n1502 = local read "Government"() -> (w742:string)
    n1503 = local read "Government"() -> (w729:string)
    n1504 = local read "Economics\nlevel"() -> (w1241:i32)
    n1505 = Greater Or Equal?(x=w335, y=4.0) -> (x >= y?=w339:bool)
    n1506 = local read "Government"() -> (w717:string)
    n1507 = Greater Or Equal?(x=w336, y=6.0) -> (x >= y?=w338:bool)
    n1508 = local read "Biology\nlevel"() -> (w1227:i32)
    n1509 = local read "EP"() -> (w167:dbl)
    n1510 = Greater Or Equal?(x=w332, y=3.0) -> (x >= y?=w340:bool)
    n1511 = local read "EP"() -> (w180:dbl)
    n1512 = Greater Or Equal?(x=w607, y=4.0) -> (x >= y?=w597:bool)
    n1513 = local read "EP"() -> (w199:dbl)
    n1514 = Greater Or Equal?(x=w608, y=2.0) -> (x >= y?=w618:bool)
    n1515 = local read "EP"() -> (w225:dbl)
    n1516 = Greater Or Equal?(x=w590, y=5.0) -> (x >= y?=w592:bool)
    n1517 = local read "EP"() -> (w238:dbl)
    n1518 = Greater Or Equal?(x=w812, y=3.0) -> (x >= y?=w810:bool)
    n1519 = local read "EP"() -> (w218:dbl)
    n1520 = Greater Or Equal?(x=w1334, y=4.0) -> (x >= y?=w1333:bool)
    n1521 = Greater Or Equal?(x=w835, y=2.0) -> (x >= y?=w837:bool)
    n1522 = Greater Or Equal?(x=w633, y=1.0) -> (x >= y?=w623:bool)
    n1523 = local read "SP"() -> (w743:dbl)
    n1524 = local read "EP"() -> (w603:dbl)
    n1525 = local read "SP"() -> (w730:dbl)
    n1526 = local read "Spear level"() -> (w1347:i32)
    n1527 = local read "EP"() -> (w612:dbl)
    n1528 = local read "SP"() -> (w716:dbl)
    n1529 = local read "EP"() -> (w305:dbl)
    n1530 = Greater Or Equal?(x=w579, y=5.0) -> (x >= y?=w591:bool)
    n1531 = local read "EP"() -> (w318:dbl)
    n1532 = Greater Or Equal?(x=w823, y=3.0) -> (x >= y?=w811:bool)
    n1533 = local read "EP"() -> (w325:dbl)
    n1534 = Greater Or Equal?(x=w824, y=2.0) -> (x >= y?=w836:bool)
    n1535 = local read "EP"() -> (w629:dbl)
    n1536 = Greater Or Equal?(x=w167, y=w168) -> (x >= y?=w172:bool)
    n1537 = Greater Or Equal?(x=w180, y=w179) -> (x >= y?=w175:bool)
    n1538 = Subtract(x=w167, y=w168) -> (x-y=w169:dbl)
    n1539 = Subtract(x=w180, y=w179) -> (x-y=w178:dbl)
    n1540 = Equal?(x=w165, y=5.0) -> (x = y?=w170:bool)
    n1541 = local read "EP"() -> (w583:dbl)
    n1542 = Greater Or Equal?(x=w199, y=w200) -> (x >= y?=w204:bool)
    n1543 = Compound Arithmetic op=AND(w170, "Rocket artillery", w161, w158, w172) -> (w173:bool)
    n1544 = local read "EP"() -> (w1342:dbl)
    n1545 = Equal?(x=w182, y=4.0) -> (x = y?=w177:bool)
    n1546 = Compound Arithmetic op=AND(w177, "Howitzer", w186, w189, w175) -> (w174:bool)
    n1547 = Increment(x=w165) -> (x+1=w166:i32)
    n1548 = local read "EP"() -> (w819:dbl)
    n1549 = Greater Or Equal?(x=w225, y=w226) -> (x >= y?=w230:bool)
    n1550 = Subtract(x=w199, y=w200) -> (x-y=w201:dbl)
    n1551 = Greater Or Equal?(x=w238, y=w237) -> (x >= y?=w233:bool)
    n1552 = Increment(x=w182) -> (x+1=w181:i32)
    n1553 = Equal?(x=w197, y=3.0) -> (x = y?=w202:bool)
    n1554 = Subtract(x=w225, y=w226) -> (x-y=w227:dbl)
    n1555 = Compound Arithmetic op=AND(w202, "Cannon", w193, w190, w204) -> (w205:bool)
    n1556 = local read "EP"() -> (w828:dbl)
    n1557 = Greater Or Equal?(x=w218, y=w217) -> (x >= y?=w213:bool)
    n1558 = Subtract(x=w238, y=w237) -> (x-y=w236:dbl)
    n1559 = Equal?(x=w223, y=1.0) -> (x = y?=w228:bool)
    n1560 = Increment(x=w197) -> (x+1=w198:i32)
    n1561 = Compound Arithmetic op=AND(w228, "Catapult", w207, w250, w230) -> (w231:bool)
    n1562 = Equal?(x=w240, y=2.0) -> (x = y?=w235:bool)
    n1563 = And(x="Iron\nSpear", y=w1333) -> (x .and. y?=w1331:bool)
    n1564 = Subtract(x=w218, y=w217) -> (x-y=w216:dbl)
    n1565 = Compound Arithmetic op=AND(w235, "Trebuchet", w244, w253, w233) -> (w232:bool)
    n1566 = Increment(x=w223) -> (x+1=w224:i32)
    n1567 = Equal?(x=w220, y=0.0) -> (x = y?=w215:bool)
    n1568 = Increment(x=w240) -> (x+1=w239:i32)
    n1569 = Compound Arithmetic op=AND(w215, "Ballista", w206, w247, w213) -> (w212:bool)
    n1570 = Increment(x=w220) -> (x+1=w219:i32)
    n1571 = Greater Or Equal?(x=w603, y=w602) -> (x >= y?=w596:bool)
    n1572 = Greater Or Equal?(x=w737, y=4) -> (x >= y?=w746:bool)
    n1573 = Greater Or Equal?(x=w743, y=5000000) -> (x >= y?=w745:bool)
    n1574 = Subtract(x=w603, y=w602) -> (x-y=w601:dbl)
    n1575 = Greater Or Equal?(x=w612, y=w613) -> (x >= y?=w619:bool)
    n1576 = Equal?(x=w605, y=2.0) -> (x = y?=w600:bool)
    n1577 = Greater Or Equal?(x=w305, y=w306) -> (x >= y?=w310:bool)
    n1578 = Compound Arithmetic op=AND(w600, "Medicine 3", w597, w596) -> (w595:bool)
    n1579 = Greater Or Equal?(x=w724, y=4) -> (x >= y?=w733:bool)
    n1580 = Subtract(x=w612, y=w613) -> (x-y=w614:dbl)
    n1581 = Increment(x=w605) -> (x+1=w604:i32)
    n1582 = Greater Or Equal?(x=w318, y=w317) -> (x >= y?=w313:bool)
    n1583 = Subtract(x=w305, y=w306) -> (x-y=w307:dbl)
    n1584 = Greater Or Equal?(x=w730, y=5000000) -> (x >= y?=w732:bool)
    n1585 = Greater Or Equal?(x=w722, y=4) -> (x >= y?=w713:bool)
    n1586 = Equal?(x=w610, y=1.0) -> (x = y?=w615:bool)
    n1587 = Compound Arithmetic op=AND(w615, "Medicine 2", w618, w619) -> (w620:bool)
    n1588 = Equal?(x=w303, y=2.0) -> (x = y?=w308:bool)
    n1589 = Greater Or Equal?(x=w716, y=5000000) -> (x >= y?=w714:bool)
    n1590 = Subtract(x=w318, y=w317) -> (x-y=w316:dbl)
    n1591 = Compound Arithmetic op=AND(w308, "Income tax", w338, w310) -> (w311:bool)
    n1592 = Increment(x=w610) -> (x+1=w611:i32)
    n1593 = Greater Or Equal?(x=w325, y=w326) -> (x >= y?=w330:bool)
    n1594 = Equal?(x=w320, y=1.0) -> (x = y?=w315:bool)
    n1595 = Increment(x=w303) -> (x+1=w304:i32)
    n1596 = Compound Arithmetic op=AND(w315, "Sales tax", w339, w313) -> (w312:bool)
    n1597 = Greater Or Equal?(x=w629, y=w628) -> (x >= y?=w622:bool)
    n1598 = Subtract(x=w325, y=w326) -> (x-y=w327:dbl)
    n1599 = Increment(x=w320) -> (x+1=w319:i32)
    n1600 = Equal?(x=w323, y=0.0) -> (x = y?=w328:bool)
    n1601 = Subtract(x=w629, y=w628) -> (x-y=w627:dbl)
    n1602 = Compound Arithmetic op=AND(w328, "Tariffs", w340, w330) -> (w331:bool)
    n1603 = Not Equal?(x=w742, y=w748) -> (x != y?=w740:bool)
    n1604 = Equal?(x=w631, y=0.0) -> (x = y?=w626:bool)
    n1605 = Increment(x=w323) -> (x+1=w324:i32)
    n1606 = Compound Arithmetic op=AND(w626, "Medicine 1", w623, w622) -> (w621:bool)
    n1607 = Greater Or Equal?(x=w1342, y=w1330) -> (x >= y?=w1341:bool)
    n1608 = And(x=w1331, y=w1341) -> (x .and. y?=w1344:bool)
    n1609 = Increment(x=w631) -> (x+1=w630:i32)
    n1610 = Not Equal?(x=w729, y=w735) -> (x != y?=w727:bool)
    n1611 = Not Equal?(x=w717, y=w711) -> (x != y?=w719:bool)
    n1612 = Greater Or Equal?(x=w583, y=w584) -> (x >= y?=w593:bool)
    n1613 = case shown="True" w173 {
      tunnel: w166 -> [_ w1576]
      tunnel: w169 -> [_ w1575]
      frame False {
      }
      frame True {
        n1614 = local write "EP"(w1575) -> ()
        n1615 = local read "warrior b"() -> (w1572:dbl)
        n1616 = local write "Siege weapon\nlevel"(w1576) -> ()
        n1617 = Add(x=w1572, y=1.0) -> (x+y=w1573:dbl)
        n1618 = local write "warrior b"(w1573) -> ()
      }
    }
    n1619 = case shown="True" w212 {
      tunnel: w219 -> [_ w1601]
      tunnel: w216 -> [_ w1600]
      frame False {
      }
      frame True {
        n1620 = local write "Siege weapon\nlevel"(w1601) -> ()
        n1621 = local write "EP"(w1600) -> ()
        n1622 = local read "warrior b"() -> (w1599:dbl)
        n1623 = Add(x=w1599, y=0.25) -> (x+y=w1598:dbl)
        n1624 = local write "warrior b"(w1598) -> ()
      }
    }
    n1625 = case shown="True" w174 {
      tunnel: w181 -> [_ w1581]
      tunnel: w178 -> [_ w1580]
      frame False {
      }
      frame True {
        n1626 = local write "EP"(w1580) -> ()
        n1627 = local read "warrior b"() -> (w1577:dbl)
        n1628 = local write "Siege weapon\nlevel"(w1581) -> ()
        n1629 = Add(x=w1577, y=1.0) -> (x+y=w1578:dbl)
        n1630 = local write "warrior b"(w1578) -> ()
      }
    }
    n1631 = Greater Or Equal?(x=w819, y=w818) -> (x >= y?=w809:bool)
    n1632 = Subtract(x=w583, y=w584) -> (x-y=w585:dbl)
    n1633 = Equal?(x=w581, y=2.0) -> (x = y?=w586:bool)
    n1634 = Subtract(x=w819, y=w818) -> (x-y=w817:dbl)
    n1635 = Compound Arithmetic op=AND(w586, "Advanced\nmetal\ntools", w591, w592, w593) -> (w594:bool)
    n1636 = case shown="True" w205 {
      tunnel: w198 -> [_ w1586]
      tunnel: w201 -> [_ w1585]
      frame False {
      }
      frame True {
        n1637 = local write "EP"(w1585) -> ()
        n1638 = local read "warrior b"() -> (w1582:dbl)
        n1639 = local write "Siege weapon\nlevel"(w1586) -> ()
        n1640 = Add(x=w1582, y=1.0) -> (x+y=w1583:dbl)
        n1641 = local write "warrior b"(w1583) -> ()
      }
    }
    n1642 = Greater Or Equal?(x=w828, y=w829) -> (x >= y?=w838:bool)
    n1643 = Equal?(x=w821, y=1.0) -> (x = y?=w816:bool)
    n1644 = Increment(x=w581) -> (x+1=w582:i32)
    n1645 = Compound Arithmetic op=AND(w816, "Basic\nmetal\ntools", w811, w810, w809) -> (w808:bool)
    n1646 = case shown="True" w231 {
      tunnel: w224 -> [_ w1596]
      tunnel: w227 -> [_ w1595]
      frame False {
      }
      frame True {
        n1647 = local write "EP"(w1595) -> ()
        n1648 = local read "warrior b"() -> (w1592:dbl)
        n1649 = local write "Siege weapon\nlevel"(w1596) -> ()
        n1650 = Add(x=w1592, y=0.5) -> (x+y=w1593:dbl)
        n1651 = local write "warrior b"(w1593) -> ()
      }
    }
    n1652 = Subtract(x=w828, y=w829) -> (x-y=w830:dbl)
    n1653 = case shown="True" w595 {
      tunnel: w604 -> [_ w1726]
      tunnel: w601 -> [_ w1725]
      frame False {
      }
      frame True {
        n1654 = local write "EP"(w1725) -> ()
        n1655 = local write "Medicine level"(w1726) -> ()
        n1656 = local write "Medicine dissent mod"(-4 ("Medicine dissent mod")) -> ()
      }
    }
    n1657 = case shown="True" w232 {
      tunnel: w239 -> [_ w1591]
      tunnel: w236 -> [_ w1590]
      frame False {
      }
      frame True {
        n1658 = local write "EP"(w1590) -> ()
        n1659 = local read "warrior b"() -> (w1589:dbl)
        n1660 = local write "Siege weapon\nlevel"(w1591) -> ()
        n1661 = Add(x=w1589, y=0.5) -> (x+y=w1588:dbl)
        n1662 = local write "warrior b"(w1588) -> ()
      }
    }
    n1663 = Increment(x=w821) -> (x+1=w820:i32)
    n1664 = Equal?(x=w826, y=0.0) -> (x = y?=w831:bool)
    n1665 = Equal?(x=w1347, y=3.0) -> (x = y?=w1345:bool)
    n1666 = And(x=w1345, y=w1344) -> (x .and. y?=w1346:bool)
    n1667 = Compound Arithmetic op=AND(w831, "Stone tools", w836, w837, w838) -> (w839:bool)
    n1668 = case shown="True" w620 {
      tunnel: w611 -> [_ w1729]
      tunnel: w614 -> [_ w1728]
      frame False {
      }
      frame True {
        n1669 = local write "EP"(w1728) -> ()
        n1670 = local write "Medicine level"(w1729) -> ()
        n1671 = local write "Medicine dissent mod"(-2 ("Medicine dissent mod")) -> ()
      }
    }
    n1672 = Increment(x=w826) -> (x+1=w827:i32)
    n1673 = And(x=w746, y=w745) -> (x .and. y?=w747:bool)
    n1674 = And(x="Feudalism", y=w747) -> (x .and. y?=w739:bool)
    n1675 = And(x=w740, y=w739) -> (x .and. y?=w741:bool)
    n1676 = case shown="True" w331 {
      tunnel: w324 -> [_ w1621]
      tunnel: w327 -> [_ w1620]
      frame False {
      }
      frame True {
        n1677 = local write "EP"(w1620) -> ()
        n1678 = local write "Tax method\nlevel"(w1621) -> ()
      }
    }
    n1679 = case shown="True" w741 {
      tunnel: w748 -> [_ w1788]
      frame False {
      }
      frame True {
        n1680 = local write "Government"(w1788) -> ()
        n1681 = local read "SP"() -> (w1785:dbl)
        n1682 = Subtract(x=w1785, y=5000000) -> (x-y=w1787:dbl)
        n1683 = local write "SP"(w1787) -> ()
      }
    }
    n1684 = And(x=w733, y=w732) -> (x .and. y?=w734:bool)
    n1685 = And(x="Caste system", y=w734) -> (x .and. y?=w726:bool)
    n1686 = And(x=w727, y=w726) -> (x .and. y?=w728:bool)
    n1687 = case shown="True" w621 {
      tunnel: w630 -> [_ w1732]
      tunnel: w627 -> [_ w1731]
      frame False {
      }
      frame True {
        n1688 = local write "EP"(w1731) -> ()
        n1689 = local write "Medicine level"(w1732) -> ()
        n1690 = local write "Medicine dissent mod"(-1 ("Medicine dissent mod")) -> ()
      }
    }
    n1691 = And(x=w713, y=w714) -> (x .and. y?=w712:bool)
    n1692 = And(x="Senate", y=w712) -> (x .and. y?=w720:bool)
    n1693 = And(x=w719, y=w720) -> (x .and. y?=w718:bool)
    n1694 = case shown="True" w311 {
      tunnel: w304 -> [_ w1617]
      tunnel: w307 -> [_ w1616]
      frame False {
      }
      frame True {
        n1695 = local write "EP"(w1616) -> ()
        n1696 = local write "Tax method\nlevel"(w1617) -> ()
      }
    }
    n1697 = case shown="True" w728 {
      tunnel: w735 -> [_ w1784]
      frame False {
      }
      frame True {
        n1698 = local write "Government"(w1784) -> ()
        n1699 = local read "SP"() -> (w1783:dbl)
        n1700 = Subtract(x=w1783, y=5000000) -> (x-y=w1781:dbl)
        n1701 = local write "SP"(w1781) -> ()
      }
    }
    n1702 = case shown="True" w312 {
      tunnel: w319 -> [_ w1619]
      tunnel: w316 -> [_ w1618]
      frame False {
      }
      frame True {
        n1703 = local write "EP"(w1618) -> ()
        n1704 = local write "Tax method\nlevel"(w1619) -> ()
      }
    }
    n1705 = local read "SP"() -> (w1225:dbl)
    n1706 = case shown="True" w718 {
      tunnel: w711 -> [_ w1780]
      frame False {
      }
      frame True {
        n1707 = local write "Government"(w1780) -> ()
        n1708 = local read "SP"() -> (w1777:dbl)
        n1709 = Subtract(x=w1777, y=5000000) -> (x-y=w1779:dbl)
        n1710 = local write "SP"(w1779) -> ()
      }
    }
    n1711 = local read "SP"() -> (w1243:dbl)
    n1712 = Power Of 10(x=w1227) -> (10^x=w1222:dbl)
    n1713 = Power Of 10(x=w1241) -> (10^x=w1247:dbl)
    n1714 = Increment(x=w1347) -> (x+1=w1348:i32)
    n1715 = case shown="True" w839 {
      tunnel: w827 -> [_ w1812]
      tunnel: w830 -> [_ w1811]
      frame False {
      }
      frame True {
        n1716 = local read "Construction multiplier"() -> (w1809:dbl)
        n1717 = local write "Construction\ntools level"(w1812) -> ()
        n1718 = local write "EP"(w1811) -> ()
        n1719 = Add(x=w1809, y=0.5) -> (x+y=w1808:dbl)
        n1720 = local write "Construction multiplier"(w1808) -> ()
      }
    }
    n1721 = case shown="True" w1346 {
      tunnel: w1342 -> [_ w2122]
      tunnel: w1348 -> [_ w2120]
      tunnel: w1330 -> [_ w2119]
      frame False {
      }
      frame True {
        n1722 = local read "warrior a"() -> (w2124:dbl)
        n1723 = local write "Spear level"(w2120) -> ()
        n1724 = Subtract(x=w2122, y=w2119) -> (x-y=w2121:dbl)
        n1725 = local write "EP"(w2121) -> ()
        n1726 = Add(x=w2124, y=0.5) -> (x+y=w2123:dbl)
        n1727 = local write "warrior a"(w2123) -> ()
      }
    }
    n1728 = case shown="True" w594 {
      tunnel: w582 -> [_ w1723]
      tunnel: w585 -> [_ w1722]
      frame False {
      }
      frame True {
        n1729 = local read "Construction multiplier"() -> (w1720:dbl)
        n1730 = local write "Construction\ntools level"(w1723) -> ()
        n1731 = local write "EP"(w1722) -> ()
        n1732 = Add(x=w1720, y=1.0) -> (x+y=w1721:dbl)
        n1733 = local write "Construction multiplier"(w1721) -> ()
      }
    }
    n1734 = case shown="True" w808 {
      tunnel: w820 -> [_ w1807]
      tunnel: w817 -> [_ w1806]
      frame False {
      }
      frame True {
        n1735 = local read "Construction multiplier"() -> (w1804:dbl)
        n1736 = local write "Construction\ntools level"(w1807) -> ()
        n1737 = local write "EP"(w1806) -> ()
        n1738 = Add(x=w1804, y=0.5) -> (x+y=w1805:dbl)
        n1739 = local write "Construction multiplier"(w1805) -> ()
      }
    }
    n1740 = Increment(x=w1227) -> (x+1=w1071:i32)
    n1741 = Index Array(array=w144, index=w1071) -> (element=w1070:dbl)
    n1742 = Power Of 2(x=w1070) -> (2^x=w1069:dbl)
    n1743 = Compound Arithmetic op=MULTIPLY(w1222, 1000, w1069) -> (w1226:dbl)
    n1744 = Greater?(x=w1225, y=w1226) -> (0:w1224:bool)
    n1745 = And(x="Biology", y=w1224) -> (x .and. y?=w1106:bool)
    n1746 = Increment(x=w1241) -> (x+1=w1074:i32)
    n1747 = Index Array(array=w144, index=w1074) -> (element=w1073:dbl)
    n1748 = Power Of 2(x=w1073) -> (2^x=w1072:dbl)
    n1749 = Compound Arithmetic op=MULTIPLY(w1247, 1000, w1072) -> (w1242:dbl)
    n1750 = Greater?(x=w1243, y=w1242) -> (0:w1245:bool)
    n1751 = And(x="Economics", y=w1245) -> (x .and. y?=w1244:bool)
    n1752 = case shown="True" w1106 {
      tunnel: w1225 -> [_ w2065]
      tunnel: w1226 -> [_ w2064]
      tunnel: w1071 -> [_ w2062]
      tunnel: [0 w2062] -> w1107
      frame False {
      }
      frame True {
        n1753 = Subtract(x=w2065, y=w2064) -> (x-y=w2063:dbl)
        n1754 = local write "SP"(w2063) -> ()
        n1755 = local write "Biology\nlevel"(w2062) -> ()
      }
    }
    n1756 = case shown="True" w1244 {
      selector: w1244 -> [w2074 w2077]
      tunnel: w1243 -> [_ w2080]
      tunnel: w1242 -> [_ w2079]
      tunnel: w1074 -> [_ w2076]
      tunnel: [w2074 w2077] -> w1105
      tunnel: [0 w2076] -> w1108
      frame False {
      }
      frame True {
        n1757 = Subtract(x=w2080, y=w2079) -> (x-y=w2078:dbl)
        n1758 = local write "SP"(w2078) -> ()
        n1759 = local write "Economics\nlevel"(w2076) -> ()
      }
    }
    n1760 = Compound Arithmetic op=OR(w1101, w1102, w1103, w1104, w1105, w1106) -> (w1113:bool)
    n1761 = local read "Military\nScience level"() -> (w346:i32)
    n1762 = local read "Military\nScience level"() -> (w345:i32)
    n1763 = local read "Physics level"() -> (w256:i32)
    n1764 = local read "Biology\nlevel"() -> (w357:i32)
    n1765 = local read "Military\nScience level"() -> (w299:i32)
    n1766 = local read "Physics level"() -> (w258:i32)
    n1767 = local read "Biology\nlevel"() -> (w352:i32)
    n1768 = local read "Military\nScience level"() -> (w349:i32)
    n1769 = local read "Physics level"() -> (w262:i32)
    n1770 = local read "Biology\nlevel"() -> (w355:i32)
    n1771 = local read "Military\nScience level"() -> (w296:i32)
    n1772 = local read "Economics\nlevel"() -> (w264:i32)
    n1773 = local read "Production\nlevel"() -> (w147:i32)
    n1774 = local read "Animal\ndomestication\nlevel"() -> (w390:i32)
    n1775 = local read "Animal\ndomestication\nlevel"() -> (w407:i32)
    n1776 = local read "Animal\ndomestication\nlevel"() -> (w410:i32)
    n1777 = local read "Writing level"() -> (w447:i32)
    n1778 = local read "Writing level"() -> (w430:i32)
    n1779 = local read "Writing level"() -> (w427:i32)
    n1780 = local read "Sword level"() -> (w387:i32)
    n1781 = local read "Sword level"() -> (w370:i32)
    n1782 = local read "Chariot level"() -> (w284:i32)
    n1783 = local read "Chariot level"() -> (w267:i32)
    n1784 = local read "Sword level"() -> (w367:i32)
    n1785 = local read "Chariot level"() -> (w287:i32)
    n1786 = Greater Or Equal?(x=w256, y=4.0) -> (x >= y?=w254:bool)
    n1787 = Greater Or Equal?(x=w357, y=1.0) -> (x >= y?=w356:bool)
    n1788 = Greater Or Equal?(x=w258, y=4.0) -> (x >= y?=w257:bool)
    n1789 = Greater Or Equal?(x=w352, y=3.0) -> (x >= y?=w350:bool)
    n1790 = Greater Or Equal?(x=w262, y=3.0) -> (x >= y?=w260:bool)
    n1791 = Greater Or Equal?(x=w355, y=2.0) -> (x >= y?=w351:bool)
    n1792 = Greater Or Equal?(x=w346, y=4.0) -> (x >= y?=w342:bool)
    n1793 = Greater Or Equal?(x=w345, y=6.0) -> (x >= y?=w343:bool)
    n1794 = Greater Or Equal?(x=w299, y=3.0) -> (x >= y?=w300:bool)
    n1795 = Greater Or Equal?(x=w264, y=4.0) -> (x >= y?=w263:bool)
    n1796 = local read "EP"() -> (w445:dbl)
    n1797 = Greater Or Equal?(x=w349, y=3.0) -> (x >= y?=w341:bool)
    n1798 = local read "EP"() -> (w432:dbl)
    n1799 = local read "SP"() -> (w149:dbl)
    n1800 = local read "EP"() -> (w425:dbl)
    n1801 = Greater Or Equal?(x=w296, y=3.0) -> (x >= y?=w301:bool)
    n1802 = Power Of 10(x=w147) -> (10^x=w152:dbl)
    n1803 = local read "EP"() -> (w392:dbl)
    n1804 = local read "EP"() -> (w405:dbl)
    n1805 = local read "EP"() -> (w412:dbl)
    n1806 = local read "EP"() -> (w385:dbl)
    n1807 = local read "EP"() -> (w372:dbl)
    n1808 = local read "EP"() -> (w365:dbl)
    n1809 = local read "EP"() -> (w282:dbl)
    n1810 = local read "EP"() -> (w269:dbl)
    n1811 = local read "EP"() -> (w289:dbl)
    n1812 = Greater Or Equal?(x=w445, y=w444) -> (x >= y?=w440:bool)
    n1813 = Greater Or Equal?(x=w432, y=w433) -> (x >= y?=w437:bool)
    n1814 = Subtract(x=w445, y=w444) -> (x-y=w443:dbl)
    n1815 = Equal?(x=w447, y=2.0) -> (x = y?=w442:bool)
    n1816 = Subtract(x=w432, y=w433) -> (x-y=w434:dbl)
    n1817 = Compound Arithmetic op=AND(w442, "Writing level 3", w440) -> (w439:bool)
    n1818 = Greater Or Equal?(x=w425, y=w424) -> (x >= y?=w420:bool)
    n1819 = Equal?(x=w430, y=1.0) -> (x = y?=w435:bool)
    n1820 = Increment(x=w447) -> (x+1=w446:i32)
    n1821 = Compound Arithmetic op=AND(w435, "Writing level 2", w437) -> (w438:bool)
    n1822 = Subtract(x=w425, y=w424) -> (x-y=w423:dbl)
    n1823 = Increment(x=w430) -> (x+1=w431:i32)
    n1824 = Equal?(x=w427, y=0.0) -> (x = y?=w422:bool)
    n1825 = Compound Arithmetic op=AND(w422, "Writing level 1", w420) -> (w419:bool)
    n1826 = Greater Or Equal?(x=w392, y=w393) -> (x >= y?=w397:bool)
    n1827 = Increment(x=w427) -> (x+1=w426:i32)
    n1828 = Greater Or Equal?(x=w405, y=w404) -> (x >= y?=w400:bool)
    n1829 = Subtract(x=w392, y=w393) -> (x-y=w394:dbl)
    n1830 = Equal?(x=w390, y=2.0) -> (x = y?=w395:bool)
    n1831 = Subtract(x=w405, y=w404) -> (x-y=w403:dbl)
    n1832 = Compound Arithmetic op=AND(w395, "Selective\nbreeding", w350, w397) -> (w398:bool)
    n1833 = Greater Or Equal?(x=w412, y=w413) -> (x >= y?=w417:bool)
    n1834 = Equal?(x=w407, y=1.0) -> (x = y?=w402:bool)
    n1835 = Increment(x=w390) -> (x+1=w391:i32)
    n1836 = Compound Arithmetic op=AND(w402, "Horses", w400, w351) -> (w399:bool)
    n1837 = Subtract(x=w412, y=w413) -> (x-y=w414:dbl)
    n1838 = Increment(x=w147) -> (x+1=w154:i32)
    n1839 = Index Array(array=w144, index=w154) -> (element=w155:dbl)
    n1840 = Power Of 2(x=w155) -> (2^x=w156:dbl)
    n1841 = Compound Arithmetic op=MULTIPLY(w152, 1000, w156) -> (w148:dbl)
    n1842 = Greater?(x=w149, y=w148) -> (0:w150:bool)
    n1843 = And(x="Production", y=w150) -> (x .and. y?=w145:bool)
    n1844 = Increment(x=w407) -> (x+1=w406:i32)
    n1845 = Equal?(x=w410, y=0.0) -> (x = y?=w415:bool)
    n1846 = Greater Or Equal?(x=w385, y=w384) -> (x >= y?=w380:bool)
    n1847 = Compound Arithmetic op=AND(w415, "Livestock", w417, w356) -> (w418:bool)
    n1848 = Increment(x=w410) -> (x+1=w411:i32)
    n1849 = Greater Or Equal?(x=w372, y=w373) -> (x >= y?=w377:bool)
    n1850 = Subtract(x=w385, y=w384) -> (x-y=w383:dbl)
    n1851 = Equal?(x=w387, y=2.0) -> (x = y?=w382:bool)
    n1852 = Subtract(x=w372, y=w373) -> (x-y=w374:dbl)
    n1853 = Compound Arithmetic op=AND(w382, "Steel sword", w343, w380) -> (w379:bool)
    n1854 = Greater Or Equal?(x=w365, y=w364) -> (x >= y?=w360:bool)
    n1855 = Equal?(x=w370, y=1.0) -> (x = y?=w375:bool)
    n1856 = Increment(x=w387) -> (x+1=w386:i32)
    n1857 = Compound Arithmetic op=AND(w375, "Iron sword", w342, w377) -> (w378:bool)
    n1858 = Subtract(x=w365, y=w364) -> (x-y=w363:dbl)
    n1859 = Greater Or Equal?(x=w282, y=w281) -> (x >= y?=w277:bool)
    n1860 = Increment(x=w370) -> (x+1=w371:i32)
    n1861 = Greater Or Equal?(x=w269, y=w270) -> (x >= y?=w274:bool)
    n1862 = Equal?(x=w367, y=0.0) -> (x = y?=w362:bool)
    n1863 = Compound Arithmetic op=AND(w362, "Bronze sword", w341, w360) -> (w359:bool)
    n1864 = Subtract(x=w282, y=w281) -> (x-y=w280:dbl)
    n1865 = Greater Or Equal?(x=w289, y=w290) -> (x >= y?=w294:bool)
    n1866 = Subtract(x=w269, y=w270) -> (x-y=w271:dbl)
    n1867 = Increment(x=w367) -> (x+1=w366:i32)
    n1868 = Equal?(x=w284, y=1.0) -> (x = y?=w279:bool)
    n1869 = Compound Arithmetic op=AND(w279, "Reinforced\nchariot", w300, w257, w277) -> (w276:bool)
    n1870 = Equal?(x=w267, y=2.0) -> (x = y?=w272:bool)
    n1871 = Subtract(x=w289, y=w290) -> (x-y=w291:dbl)
    n1872 = Compound Arithmetic op=AND(w272, "Caravan", w263, w254, w274) -> (w275:bool)
    n1873 = case shown="True" w419 {
      tunnel: w426 -> [_ w1663]
      tunnel: w423 -> [_ w1662]
      frame False {
      }
      frame True {
        n1874 = local write "EP"(w1662) -> ()
        n1875 = local write "Writing level"(w1663) -> ()
      }
    }
    n1876 = Increment(x=w284) -> (x+1=w283:i32)
    n1877 = Equal?(x=w287, y=0.0) -> (x = y?=w292:bool)
    n1878 = Increment(x=w267) -> (x+1=w268:i32)
    n1879 = Compound Arithmetic op=AND(w292, "Simple\nchariot", w301, w260, w294) -> (w295:bool)
    n1880 = Increment(x=w287) -> (x+1=w288:i32)
    n1881 = case shown="True" w439 {
      tunnel: w446 -> [_ w1659]
      tunnel: w443 -> [_ w1658]
      frame False {
      }
      frame True {
        n1882 = local write "EP"(w1658) -> ()
        n1883 = local write "Writing level"(w1659) -> ()
      }
    }
    n1884 = case shown="True" w418 {
      tunnel: w411 -> [_ w1657]
      tunnel: w414 -> [_ w1656]
      frame False {
      }
      frame True {
        n1885 = local write "Animal\ndomestication\nlevel"(w1657) -> ()
        n1886 = local read "hunting b"() -> (w1655:dbl)
        n1887 = local write "EP"(w1656) -> ()
        n1888 = Add(x=w1655, y=0.25) -> (x+y=w1654:dbl)
        n1889 = local write "hunting b"(w1654) -> ()
      }
    }
    n1890 = case shown="True" w438 {
      tunnel: w431 -> [_ w1661]
      tunnel: w434 -> [_ w1660]
      frame False {
      }
      frame True {
        n1891 = local write "EP"(w1660) -> ()
        n1892 = local write "Writing level"(w1661) -> ()
      }
    }
    n1893 = case shown="True" w398 {
      tunnel: w391 -> [_ w1644]
      tunnel: w394 -> [_ w1643]
      frame False {
      }
      frame True {
        n1894 = local write "Animal\ndomestication\nlevel"(w1644) -> ()
        n1895 = local read "warrior a"() -> (w1640:dbl)
        n1896 = local read "Construction multiplier"() -> (w1638:dbl)
        n1897 = local write "EP"(w1643) -> ()
        n1898 = Add(x=w1638, y=0.5) -> (x+y=w1639:dbl)
        n1899 = Add(x=w1640, y=0.25) -> (x+y=w1642:dbl)
        n1900 = local write "Construction multiplier"(w1639) -> ()
        n1901 = local write "warrior a"(w1642) -> ()
      }
    }
    n1902 = case shown="True" w399 {
      tunnel: w406 -> [_ w1652]
      tunnel: w403 -> [_ w1651]
      frame False {
      }
      frame True {
        n1903 = local write "Animal\ndomestication\nlevel"(w1652) -> ()
        n1904 = local write "EP"(w1651) -> ()
        n1905 = local read "warrior b"() -> (w1648:dbl)
        n1906 = local read "Construction multiplier"() -> (w1646:dbl)
        n1907 = Add(x=w1646, y=0.5) -> (x+y=w1645:dbl)
        n1908 = Add(x=w1648, y=0.25) -> (x+y=w1649:dbl)
        n1909 = local write "Construction multiplier"(w1645) -> ()
        n1910 = local write "warrior b"(w1649) -> ()
      }
    }
    n1911 = case shown="True" w145 {
      tunnel: w149 -> [_ w1571]
      tunnel: w148 -> [_ w1570]
      tunnel: w154 -> [_ w1568]
      tunnel: [0 w1568] -> w146
      frame False {
      }
      frame True {
        n1912 = Subtract(x=w1571, y=w1570) -> (x-y=w1569:dbl)
        n1913 = local write "SP"(w1569) -> ()
        n1914 = local write "Production\nlevel"(w1568) -> ()
      }
    }
    n1915 = case shown="True" w1113 {
      tunnel: w1112 -> [_ w1896]
      tunnel: w1111 -> [_ w1899]
      tunnel: w1110 -> [_ w1902]
      tunnel: w1109 -> [_ w1905]
      tunnel: w1108 -> [_ w1908]
      tunnel: w1107 -> [_ w1911]
      tunnel: w1106 -> [_ w1910]
      tunnel: w1105 -> [_ w1907]
      tunnel: w1104 -> [_ w1904]
      tunnel: w1103 -> [_ w1901]
      tunnel: w1102 -> [_ w1898]
      tunnel: w1101 -> [_ w1895]
      tunnel: w146 -> [_ w1884]
      tunnel: w145 -> [_ w1883]
      frame False {
      }
      frame True {
        n1916 = Boolean To (0,1)(Boolean=w1895) -> (0, 1=w1894:i16)
        n1917 = Boolean To (0,1)(Boolean=w1898) -> (0, 1=w1897:i16)
        n1918 = Boolean To (0,1)(Boolean=w1901) -> (0, 1=w1900:i16)
        n1919 = Boolean To (0,1)(Boolean=w1910) -> (0, 1=w1909:i16)
        n1920 = Boolean To (0,1)(Boolean=w1904) -> (0, 1=w1903:i16)
        n1921 = Boolean To (0,1)(Boolean=w1907) -> (0, 1=w1906:i16)
        n1922 = Boolean To (0,1)(Boolean=w1883) -> (0, 1=w1886:i16)
        n1923 = Multiply(x=w1894, y=w1896) -> (x*y=w1893:i32)
        n1924 = Multiply(x=w1897, y=w1899) -> (x*y=w1892:i32)
        n1925 = Multiply(x=w1900, y=w1902) -> (x*y=w1891:i32)
        n1926 = Multiply(x=w1909, y=w1911) -> (x*y=w1888:i32)
        n1927 = Multiply(x=w1903, y=w1905) -> (x*y=w1890:i32)
        n1928 = Multiply(x=w1906, y=w1908) -> (x*y=w1889:i32)
        n1929 = Multiply(x=w1886, y=w1884) -> (x*y=w1885:i32)
        n1930 = Compound Arithmetic op=ADD(w1893, w1892, w1891, w1890, w1889, w1888, w1885) -> (w1887:i32)
        n1931 = case shown="1" w1887 {
          frame 0, Default {
          }
          frame 1 {
            n1932 = local read "# of level 1 sciences"() -> (w1913:i32)
            n1933 = Increment(x=w1913) -> (x+1=w1912:i32)
            n1934 = local write "# of level 1 sciences"(w1912) -> ()
          }
          frame 2 {
            n1935 = local read "# of level 2 sciences"() -> (w1915:i32)
            n1936 = Increment(x=w1915) -> (x+1=w1914:i32)
            n1937 = local write "# of level 2 sciences"(w1914) -> ()
          }
          frame 3 {
            n1938 = local read "# of level 3 sciences"() -> (w1917:i32)
            n1939 = Increment(x=w1917) -> (x+1=w1916:i32)
            n1940 = local write "# of level 3 sciences"(w1916) -> ()
          }
          frame 4 {
            n1941 = local read "# of level 4 sciences"() -> (w1919:i32)
            n1942 = Increment(x=w1919) -> (x+1=w1918:i32)
            n1943 = local write "# of level 4 sciences"(w1918) -> ()
          }
          frame 5 {
            n1944 = local read "# of level 5 sciences"() -> (w1921:i32)
            n1945 = Increment(x=w1921) -> (x+1=w1920:i32)
            n1946 = local write "# of level 5 sciences"(w1920) -> ()
          }
          frame 6 {
            n1947 = local read "# of level 6 sciences"() -> (w1923:i32)
            n1948 = Increment(x=w1923) -> (x+1=w1922:i32)
            n1949 = local write "# of level 6 sciences"(w1922) -> ()
          }
          frame 7 {
            n1950 = local read "# of level 7 sciences"() -> (w1925:i32)
            n1951 = Increment(x=w1925) -> (x+1=w1924:i32)
            n1952 = local write "# of level 7 sciences"(w1924) -> ()
          }
          frame 8 {
            n1953 = local read "# of level 8 sciences"() -> (w1927:i32)
            n1954 = Increment(x=w1927) -> (x+1=w1926:i32)
            n1955 = local write "# of level 8 sciences"(w1926) -> ()
          }
          frame 9 {
            n1956 = local read "# of level 9 sciences"() -> (w1929:i32)
            n1957 = Increment(x=w1929) -> (x+1=w1928:i32)
            n1958 = local write "# of level 9 sciences"(w1928) -> ()
          }
          frame 10 {
            n1959 = local read "# of level 10 sciences"() -> (w1931:i32)
            n1960 = Increment(x=w1931) -> (x+1=w1930:i32)
            n1961 = local write "# of level 10 sciences"(w1930) -> ()
          }
        }
      }
    }
    n1962 = case shown="True" w359 {
      tunnel: w366 -> [_ w1636]
      tunnel: w363 -> [_ w1635]
      frame False {
      }
      frame True {
        n1963 = local write "EP"(w1635) -> ()
        n1964 = local read "warrior b"() -> (w1634:dbl)
        n1965 = local write "Sword level"(w1636) -> ()
        n1966 = Add(x=w1634, y=0.25) -> (x+y=w1632:dbl)
        n1967 = local write "warrior b"(w1632) -> ()
      }
    }
    n1968 = case shown="True" w379 {
      tunnel: w386 -> [_ w1626]
      tunnel: w383 -> [_ w1625]
      frame False {
      }
      frame True {
        n1969 = local read "warrior a"() -> (w1622:dbl)
        n1970 = local write "EP"(w1625) -> ()
        n1971 = local write "Sword level"(w1626) -> ()
        n1972 = Add(x=w1622, y=0.25) -> (x+y=w1624:dbl)
        n1973 = local write "warrior a"(w1624) -> ()
      }
    }
    n1974 = case shown="True" w295 {
      tunnel: w288 -> [_ w1615]
      tunnel: w291 -> [_ w1614]
      frame False {
      }
      frame True {
        n1975 = local write "EP"(w1614) -> ()
        n1976 = local read "warrior b"() -> (w1613:dbl)
        n1977 = local write "Chariot level"(w1615) -> ()
        n1978 = Add(x=w1613, y=0.25) -> (x+y=w1612:dbl)
        n1979 = local write "warrior b"(w1612) -> ()
      }
    }
    n1980 = case shown="True" w378 {
      tunnel: w371 -> [_ w1631]
      tunnel: w374 -> [_ w1630]
      frame False {
      }
      frame True {
        n1981 = local write "EP"(w1630) -> ()
        n1982 = local read "warrior a"() -> (w1627:dbl)
        n1983 = local write "Sword level"(w1631) -> ()
        n1984 = Add(x=w1627, y=0.25) -> (x+y=w1628:dbl)
        n1985 = local write "warrior a"(w1628) -> ()
      }
    }
    n1986 = case shown="True" w276 {
      tunnel: w283 -> [_ w1610]
      tunnel: w280 -> [_ w1609]
      frame False {
      }
      frame True {
        n1987 = local write "EP"(w1609) -> ()
        n1988 = local read "warrior a"() -> (w1606:dbl)
        n1989 = local write "Chariot level"(w1610) -> ()
        n1990 = Add(x=w1606, y=0.25) -> (x+y=w1607:dbl)
        n1991 = local write "warrior a"(w1607) -> ()
      }
    }
    n1992 = case shown="True" w275 {
      tunnel: w268 -> [_ w1605]
      tunnel: w271 -> [_ w1604]
      frame False {
      }
      frame True {
        n1993 = local read "Trading level no mod"() -> (w1603:i32)
        n1994 = local write "EP"(w1604) -> ()
        n1995 = local write "Chariot level"(w1605) -> ()
        n1996 = Increment(x=w1603) -> (x+1=w1602:i32)
        n1997 = local write "Trading level no mod"(w1602) -> ()
      }
    }
  }
  "warrior a" <- 1.0 ("warrior a")
  "hunting b" <- 2.0 ("hunting b")
  "hunting a" <- 1.0 ("hunting a")
  "warrior b" <- 1.0 ("warrior b")
  "Food" <- 0.0
  "People" <- 10
  "Permanent\nland" <- 5.0 ("Permanent\nland")
  "Conquered\nland" <- 0.0 ("Temporary\nland")
  "warrior c" <- 2.0 ("Numeric")
  "Hunters" <- 10 ("Hunters")
  "Unassigned workers" <- 0 ("Unassigned workers")
  "Builders" <- 0 ("Builders")
  "Warriors" <- 0 ("Warriors")
  "Scientists" <- 0 ("Hunters")
  "Crafters" <- 0 ("Builders")
  "Engineers" <- 0 ("Warriors")
  "EP" <- 0.0 ("Engineering\nPoints")
  "Spear level" <- 0 ("Spear level")
  "Net level" <- 0 ("Net level")
  "SP" <- 0.0 ("Numeric")
  "Military\nScience level" <- 0 ("Military level")
  "Dissent" <- 0 ("Dissent")
  "Government" <- "Tribe" ("String")
  "Governance\nlevel" <- 0 ("Numeric")
  "Dissent multiplier" <- 1 ("Numeric")
  "Warrior b Gov mult" <- 1 ("Warrior a Gov mult")
  "Land conv mult" <- 0 ("Land conv mult")
  "Temp land change/s" <- 0 ("Temp land captured/s")
  "1-Dissent/100" <- 1.0 ("1-dissent")
  "Bow level" <- 0 ("Numeric")
  "Military Modifier" <- 1.0 ("Military Modifier")
  "Physics level" <- 0 ("Military level")
  "Construction\nlevel" <- 0 ("Numeric")
  "Boat level" <- 0 ("Spear level")
  "Trading level no mod" <- 0 ("Spear level")
  "Economics\nlevel" <- 0 ("Economic\nlevel")
  "Gold" <- 0.0 ("Gold")
  "Taxation\nlevel" <- 0.0 ("Numeric")
  "Taxation\nModifier" <- 1.0 ("Numeric")
  "Farming level" <- 0 ("Numeric")
  "Biology\nlevel" <- 0 ("Numeric")
  "Hut level" <- 0 ("Numeric")
  "Road level" <- 0 ("Numeric")
  "Brick house level" <- 0 ("Numeric")
  "Build points" <- 0 ("Numeric")
  "Non-land production multiplier" <- 1 ("Numeric")
  "Dissent addition modifiers" <- 0 ("Dissent addition modifiers")
  "Hut non-land prod mod" <- 1 ("Numeric")
  "Hut upkeep" <- 0 ("Numeric")
  "Hut dissent mod" <- 0 ("Numeric")
  "Road land prod mod" <- 1 ("Numeric")
  "Road upkeep" <- 0 ("Numeric")
  "Road expansion bonus" <- 0 ("Numeric")
  "Trading level" <- 0 ("Spear level")
  "Gov building\nupkeep mod" <- 1 ("Numeric")
  "BP upkeep" <- 0.0 ("BP/s")
  "# of level 1 sciences" <- 0 ("Numeric")
  "# of level 2 sciences" <- 0 ("Numeric")
  "# of level 3 sciences" <- 0 ("Numeric")
  "# of level 4 sciences" <- 0 ("Numeric")
  "# of level 5 sciences" <- 0 ("Numeric")
  "# of level 6 sciences" <- 0 ("Numeric")
  "# of level 7 sciences" <- 0 ("Numeric")
  "# of level 8 sciences" <- 0 ("Numeric")
  "# of level 9 sciences" <- 0 ("Numeric")
  "# of level 10 sciences" <- 0 ("Numeric")
  "Hut invested points" <- 0 ("Numeric")
  "Road invested points" <- 0 ("Numeric")
  "Taxes dissent mod" <- 0 ("Numeric")
  "Gold income/s" <- 0.0 ("1-dissent")
  "Barracks level" <- 0 ("Numeric")
  "Barracks military bonus" <- 1 ("Numeric")
  "Barracks upkeep" <- 0 ("Numeric")
  "Walls level" <- 0 ("Numeric")
  "Wall warrior % equivalent" <- 0 ("Numeric")
  "Wall upkeep" <- 0 ("Numeric")
  "Wall dissent mod" <- 0 ("Numeric")
  "Barracks\ninvested points" <- 0 ("Numeric")
  "Wall invested points" <- 0 ("Numeric")
  "Construction\ntools level" <- 0 ("Numeric")
  "Gold upkeep" <- 0 ("Land conv mult")
  "Construction multiplier" <- 1 ("Construction multiplier")
  "BP income" <- 0.0 ("Construction multiplier")
  "School level" <- 0 ("Numeric")
  "School engineer equivalent" <- 0 ("Numeric")
  "School upkeep" <- 0 ("Numeric")
  "School dissent mod" <- 0 ("Numeric")
  "School invested points" <- 0 ("Numeric")
  "School SP/EP multiplier" <- 1 ("Numeric")
  "Medicine level" <- 0 ("Spear level")
  "Medicine dissent mod" <- 0 ("Spear level")
  "University level" <- 0 ("Numeric")
  "University scientist equivalent" <- 0 ("Numeric")
  "University upkeep" <- 0 ("Numeric")
  "University dissent mod" <- 0 ("Numeric")
  "University\ninvested points" <- 0 ("Numeric")
  "University SP multiplier" <- 1 ("Numeric")
  "Gov populist\nbuildings mod" <- 1 ("Numeric")
  "Gov elitist\nbuildings mod" <- 1 ("Numeric")
  "-dissent per\nmilitary building" <- 1 ("Numeric")
  "Gov Economy\nbuildings mod" <- 1 ("Numeric")
  "Food dissent mod" <- 0 ("Numeric")
  "Food consumption\nmultiplier" <- 1 ("Numeric")
  "food income" <- 0 ("food check")
  "EP income" <- 0.0 ("Construction multiplier")
  "SP income" <- 0.0 ("Construction multiplier")
  "Animal\ndomestication\nlevel" <- 0 ("Numeric")
  "Sword level" <- 0 ("Numeric")
  "Tax method\nlevel" <- 0 ("Numeric")
  "Chariot level" <- 0 ("Numeric")
  "Siege weapon\nlevel" <- 0 ("Numeric")
  "Writing level" <- 0 ("Numeric")
  "Aqueduct level" <- 0 ("Numeric")
  "Aqueduct upkeep" <- 0 ("Numeric")
  "Aqueduct dissent mod" <- 0 ("Numeric")
  "Aqueduct\ninvested points" <- 0 ("Numeric")
  "Mansion level" <- 0 ("Numeric")
  "Mansion upkeep" <- 0 ("Numeric")
  "Mansion dissent mod" <- 0 ("Numeric")
  "Mansion\ninvested points" <- 0 ("Numeric")
  "Harbor level" <- 0 ("Numeric")
  "Harbor upkeep" <- 0 ("Numeric")
  "Harbor dissent mod" <- 0 ("Numeric")
  "Harbor\ninvested points" <- 0 ("Numeric")
  "Circus/arena level" <- 0 ("Numeric")
  "Circus upkeep" <- 0 ("Numeric")
  "Circus dissent mod" <- 0 ("Numeric")
  "Circus\ninvested points" <- 0 ("Numeric")
  "Temple level" <- 0 ("Numeric")
  "Temple upkeep" <- 0 ("Numeric")
  "Temple dissent mod" <- 0 ("Numeric")
  "Temple\ninvested points" <- 0 ("Numeric")
  "SP/EP multiplier" <- 0.0 ("Construction multiplier")
  "Harbor military mod" <- 0 ("Numeric")
  "Production\nlevel" <- 0 ("Numeric")
  "Tier 1\nproducts" <- 0.0 ("Gold")
  "Tier 2\nproducts" <- 0.0 ("Gold")
  "Tier 3\nproducts" <- 0.0 ("Gold")
  "Tier 4\nproducts" <- 0.0 ("Gold")
  "Tier 1\nproducts\nupkeep" <- 0.0 ("Gold")
  "Tier 2\nproducts\nupkeep" <- 0.0 ("Gold")
  "Tier 3\nproducts\nupkeep" <- 0.0 ("Gold")
  "Tier 4\nproducts\nupkeep" <- 0.0 ("Gold")
